vi "20191023_KEK_HEX5_events_new_config.vi"() -> ()   [LabVIEW 2017]
uses:
  <vilib>/DAQmx/create/channels.llb/DAQmx Create Channel (AI-Voltage-Basic).vi
  <vilib>/DAQmx/create/channels.llb/DAQmx Create Channel (AO-Voltage-Basic).vi
  <vilib>/DAQmx/miscellaneous.llb/DAQmx Fill In Error Info.vi
  Lake Shore Cryotronics 218.lvlib
panel:
  out "ref RAW":refnum<file>
  out "ref LSI-D":refnum<file>
  out "ref DAQ":refnum<file>
  in  "CSV filename suffix":string="Overnight_1030"
  in  "base path":path=path "C:/Users/TUCAN_rcnp/Desktop/Labview/KEK_20191023_HEX5/EXP"
  out "ref LSI-U":refnum<file>
  out "size(s)":i32[](array[numeric])=[11, 5]
  out "Cycle #":i32=311
  out "current time":timestamp=timestamp(3655268207.996145 s since 1904-01-01)
  in  "stop":bool
  in  "Tab Control":T1(tab)=enum." DAQ out"
  out "error out \n(LSIU)":errorcluster
  out "error out\n(file creation)":errorcluster
  out "error out\n(DAQ config)":errorcluster
  out "error out\n(DAQ OUT)":errorcluster
  out "error out \n(DAQ IN)":errorcluster
  out "error out \n(record LSIU)":errorcluster
  out "error out \n(record DAQ)":errorcluster
  out "error out DAQ close":errorcluster
  out "error out \n(LSID)":errorcluster
  out "error out \n(record LSID)":errorcluster
  out "errors plot cosmetic 1":errorcluster[](array[cluster])
  out "error plot content":errorcluster
  out "error plot cosmetic 2":errorcluster
  in  "comments DAQ (not recorded)":string[](array[string])=["", "", "", "", "", "", "The range of this is 0-10VDC", "", "", "", ""]
  in  "comments LSID (not recorded)":string[](array[string])=["", "", "", "", "Broken", "", "", ""]
  in  "comments LSIU (not recorded)":string[](array[string])=["", "", "", "", "", "", "", ""]
  in  "V_max(in)":dbl[](array[numeric])=[5.0, 0.15, 5.0, 5.0, 5.0, 5.0, 10.0, 5.0, 5.0, 5.0, 5.0]
  in  "NI DAQ AIN labels":string[](array[string])=["P_4KRES_COILIN", "LM_110", "DP_4He", "DP_3He", "FM_4He", "FM_3He", "LM_1700", "P_4He_IN", "Bar_anal", "bar_CDG1", "bar_CDG2"]
  in  "LSI-U CH labels":string[](array[string])=["4K_res", "HEX5_liq_IN", "HEX_liq_OUT", "1K_pot", "HEX5_gas_IN", "HEX5_gas_OUT", "JT_IN", "JT_OUT"]
  in  "LSI-D CH labels":string[](array[string])=["Hflex_low", "uper_duct", "Hflex_up", "DISABLED", "4K_res", "HEX5_liq_IN_PtCo", "HEX5_liq_OUT_PtCo", "1K_pot_PtCo"]
  in  "DAQ analog channels":tag[](array[tag])=["Dev1/ai1", "Dev1/ai2", "Dev1/ai3", "Dev1/ai4", "Dev1/ai5", "Dev1/ai6", "Dev1/ai7", "Dev1/ai16", "Dev1/ai18", "Dev1/ai19", "Dev1/ai20"]
  in  "V_min(in)":dbl[](array[numeric])=[0.0, 0.0, 0.0, 0.0, 0.0, 0.0, 0.0, 0.0, 0.0, 0.0, 0.0]
  out "DAQ CH OUT":string="O1"
  in  "DAQ  OUT":tag="Dev1/ao0"
  in  "DAQ OUT ON?":bool
  in  "V_min(out)":dbl
  in  "V_max(out)":dbl=5.0
  out "DAQ CH 2":string[](array[string])=["Q1", "Q2", "Q3", "Q4", "Q5", "Q6", "Q7", "Q8", "Q9", "Q10", "Q11"]
  out "LSI-D CH 2":string[](array[string])=["D1", "D2", "D3", "D4", "D5", "D6", "D7", "D8"]
  in  "DAQ sample #":i32=5
  out "LSI-U CH 2":string[](array[string])=["U1", "U2", "U3", "U4", "U5", "U6", "U7", "U8"]
  in  "VISA LSI218 UP":refnum<visa-resource-name>="GPIB0::3::INSTR"
  in  "VISA LSI218 DOWN":refnum<visa-resource-name>="GPIB0::11::INSTR"
  out "D idx":i32[](array[numeric])=[0, 1, 2, 3, 4, 5, 6, 7]
  out "LSI-U CH indic,":string[](array[string])=["4K_res", "HEX5_liq_IN", "HEX_liq_OUT", "1K_pot", "HEX5_gas_IN", "HEX5_gas_OUT", "JT_IN", "JT_OUT"]
  out "LSI-U out":dbl[](array[numeric])=[284.87, 0.0, 330.07, 0.718, 286.24, 89.901, 283.56, 272.5]
  in  "GraphU1 SEL":i32[](array[numeric])=[0, 1]
  out "LSI-D out":dbl[](array[numeric])=[296.51, 230.81, 237.57, 20.995, 4.242, 6.869, 297.3, 283.3]
  out "LSI-D CH indic.":string[](array[string])=["Hflex_low", "uper_duct", "Hflex_up", "DISABLED", "4K_res", "HEX5_liq_IN_PtCo", "HEX5_liq_OUT_PtCo", "1K_pot_PtCo"]
  in  "GraphU2 SEL":i32[](array[numeric])=[2, 3, 4]
  in  "GraphU3 SEL":i32[](array[numeric])=[5, 6, 6]
  in  "GraphD1 SEL":i32[](array[numeric])=[0, 1]
  in  "GraphD2 SEL":i32[](array[numeric])=[2, 3, 4]
  in  "GraphD3 SEL":i32[](array[numeric])=[5, 6, 6]
  out "LSI-D Grpah 1":cluster{dbl[], dbl[]}[](graph)=[{array[312 elements], [0.0, 296.61, 296.59, 296.63, 296.62, 296.61, 296.61, 296.61, 296.61, 296.61, 296.57, 296.65, 296.6, 296.66, 296.59, 296.6, 296.58, 296.64, 296.63, 296.66, 296.57, 296.61, 296.6, 296.6, 296.61, 296.61, 296.6, 296.6, 296.57, 296.62, 296.58, 296.59, 296.58, 296.61, 296.62, 296.57, 296.61, 296.63, 296.62, 296.64, 296.63, 296.6, 296.6, 296.57, 296.59, 296.59, 296.6, 296.59, 296.56, 296.6, 296.59, 296.61, 296.59, 296.58, 296.57, 296.59, 296.62, 296.59, 296.61, 296.6, 296.55, 296.6, 296.59, 296.59, 296.6, 296.61, 296.59, 296.57, 296.64, 296.67, 296.57, 296.62, 296.57, 296.58, 296.62, 296.61, 296.58, 296.55, 296.56, 296.59, 296.59, 296.6, 296.58, 296.57, 296.61, 296.58, 296.53, 296.54, 296.59, 296.55, 296.53, 296.59, 296.58, 296.58, 296.58, 296.55, 296.56, 296.56, 296.59, 296.53, 296.61, 296.62, 296.6, 296.58, 296.56, 296.53, 296.55, 296.59, 296.58, 296.6, 296.55, 296.59, 296.56, 296.56, 296.58, 296.57, 296.61, 296.55, 296.61, 296.57, 296.57, 296.58, 296.51, 296.55, 296.6, 296.6, 296.58, 296.56, 296.58, 296.57, 296.59, 296.55, 296.55, 296.56, 296.59, 296.52, 296.54, 296.58, 296.52, 296.54, 296.57, 296.54, 296.59, 296.52, 296.53, 296.55, 296.49, 296.54, 296.63, 296.56, 296.53, 296.54, 296.55, 296.58, 296.56, 296.51, 296.55, 296.57, 296.53, 296.52, 296.56, 296.58, 296.55, 296.61, 296.55, 296.58, 296.53, 296.58, 296.57, 296.52, 296.48, 296.53, 296.52, 296.54, 296.59, 296.53, 296.56, 296.55, 296.58, 296.56, 296.51, 296.52, 296.57, 296.54, 296.55, 296.55, 296.57, 296.59, 296.6, 296.55, 296.54, 296.51, 296.52, 296.55, 296.55, 296.54, 296.51, 296.49, 296.57, 296.55, 296.54, 296.56, 296.55, 296.53, 296.5, 296.55, 296.53, 296.54, 296.57, 296.52, 296.55, 296.55, 296.52, 296.5, 296.53, 296.53, 296.52, 296.54, 296.53, 296.52, 296.53, 296.51, 296.58, 296.49, 296.52, 296.55, 296.48, 296.51, 296.55, 296.48, 296.55, 296.5, 296.51, 296.55, 296.52, 296.54, 296.5, 296.54, 296.52, 296.53, 296.55, 296.53, 296.48, 296.58, 296.55, 296.52, 296.51, 296.49, 296.53, 296.5, 296.56, 296.53, 296.48, 296.54, 296.52, 296.56, 296.53, 296.5, 296.51, 296.5, 296.51, 296.47, 296.47, 296.57, 296.53, 296.49, 296.56, 296.55, 296.55, 296.51, 296.5, 296.52, 296.52, 296.48, 296.51, 296.54, 296.5, 296.49, 296.55, 296.5, 296.52, 296.54, 296.5, 296.51, 296.5, 296.53, 296.49, 296.51, 296.49, 296.54, 296.5, 296.51, 296.5, 296.54, 296.5, 296.48, 296.46, 296.5, 296.49, 296.49, 296.49, 296.51, 296.47, 296.49, 296.47, 296.49, 296.47, 296.49, 296.46, 296.49, 296.47, 296.51]}, {array[312 elements], [0.0, 246.36, 246.3, 246.25, 246.18, 246.13, 246.13, 246.1, 246.04, 246.01, 245.96, 245.88, 245.85, 245.76, 245.73, 245.71, 245.65, 245.59, 245.54, 245.5, 245.46, 245.41, 245.35, 245.32, 245.31, 245.24, 245.17, 245.15, 245.05, 245.05, 244.99, 244.94, 244.92, 244.85, 244.84, 244.72, 244.69, 244.62, 244.56, 244.56, 244.49, 244.46, 244.4, 244.4, 244.3, 244.3, 244.25, 244.17, 244.13, 244.08, 244.03, 243.99, 243.95, 243.89, 243.86, 243.79, 243.75, 243.69, 243.65, 243.6, 243.56, 243.49, 243.42, 243.43, 243.36, 243.34, 243.27, 243.21, 243.12, 243.17, 243.07, 243.05, 242.97, 242.87, 242.88, 242.8, 242.77, 242.72, 242.65, 242.64, 242.55, 242.51, 242.45, 242.46, 242.37, 242.29, 242.28, 242.21, 242.18, 242.14, 242.06, 242.07, 242.0, 241.92, 241.91, 241.84, 241.77, 241.71, 241.66, 241.64, 241.57, 241.52, 241.46, 241.4, 241.37, 241.32, 241.26, 241.23, 241.17, 241.15, 241.07, 241.0, 240.93, 240.92, 240.86, 240.78, 240.76, 240.7, 240.65, 240.57, 240.51, 240.46, 240.46, 240.37, 240.33, 240.29, 240.19, 240.16, 240.13, 240.09, 240.0, 239.96, 239.91, 239.87, 239.83, 239.75, 239.71, 239.63, 239.57, 239.52, 239.48, 239.39, 239.35, 239.35, 239.29, 239.2, 239.19, 239.07, 239.04, 239.02, 238.97, 238.87, 238.8, 238.79, 238.73, 238.67, 238.61, 238.57, 238.54, 238.45, 238.38, 238.36, 238.28, 238.24, 238.21, 238.17, 238.09, 238.05, 237.98, 237.95, 237.88, 237.82, 237.8, 237.73, 237.64, 237.6, 237.58, 237.52, 237.49, 237.43, 237.33, 237.29, 237.26, 237.22, 237.17, 237.11, 237.06, 237.01, 236.97, 236.91, 236.84, 236.8, 236.75, 236.69, 236.64, 236.56, 236.53, 236.45, 236.43, 236.38, 236.33, 236.28, 236.23, 236.16, 236.13, 236.07, 236.01, 235.93, 235.93, 235.88, 235.82, 235.78, 235.72, 235.63, 235.6, 235.57, 235.52, 235.47, 235.43, 235.34, 235.32, 235.25, 235.23, 235.16, 235.11, 235.07, 235.02, 234.92, 234.93, 234.85, 234.8, 234.75, 234.71, 234.65, 234.62, 234.52, 234.5, 234.47, 234.42, 234.38, 234.32, 234.23, 234.19, 234.14, 234.08, 234.06, 234.03, 233.95, 233.91, 233.85, 233.79, 233.74, 233.73, 233.68, 233.61, 233.58, 233.51, 233.46, 233.41, 233.36, 233.32, 233.27, 233.24, 233.16, 233.11, 233.11, 233.03, 232.95, 232.9, 232.89, 232.8, 232.8, 232.72, 232.69, 232.65, 232.58, 232.52, 232.5, 232.44, 232.38, 232.34, 232.26, 232.21, 232.17, 232.13, 232.11, 232.03, 231.97, 231.96, 231.91, 231.88, 231.82, 231.77, 231.7, 231.65, 231.59, 231.59, 231.49, 231.49, 231.38, 231.35, 231.31, 231.25, 231.21, 231.19, 231.16, 231.09, 230.99, 230.97, 230.95, 230.89, 230.81]}, {array[312 elements], [0.0, 251.98, 251.95, 251.89, 251.86, 251.82, 251.77, 251.73, 251.67, 251.64, 251.61, 251.56, 251.51, 251.45, 251.42, 251.36, 251.34, 251.3, 251.22, 251.19, 251.19, 251.14, 251.06, 251.04, 250.98, 250.95, 250.91, 250.87, 250.82, 250.77, 250.74, 250.67, 250.65, 250.6, 250.55, 250.52, 250.46, 250.41, 250.37, 250.34, 250.28, 250.24, 250.21, 250.15, 250.11, 250.08, 250.04, 249.99, 249.94, 249.87, 249.85, 249.81, 249.77, 249.73, 249.67, 249.63, 249.58, 249.55, 249.48, 249.47, 249.4, 249.35, 249.32, 249.28, 249.25, 249.19, 249.15, 249.1, 249.05, 249.01, 248.98, 248.92, 248.85, 248.82, 248.79, 248.76, 248.71, 248.65, 248.6, 248.55, 248.52, 248.47, 248.44, 248.38, 248.36, 248.3, 248.26, 248.19, 248.13, 248.12, 248.06, 248.03, 247.98, 247.93, 247.86, 247.85, 247.82, 247.74, 247.7, 247.66, 247.63, 247.58, 247.54, 247.48, 247.43, 247.4, 247.33, 247.3, 247.25, 247.2, 247.16, 247.1, 247.09, 247.02, 246.96, 246.93, 246.88, 246.85, 246.79, 246.76, 246.7, 246.66, 246.6, 246.58, 246.53, 246.47, 246.44, 246.4, 246.34, 246.28, 246.23, 246.18, 246.14, 246.1, 246.05, 246.01, 245.98, 245.94, 245.86, 245.85, 245.79, 245.72, 245.68, 245.65, 245.62, 245.54, 245.52, 245.46, 245.42, 245.37, 245.3, 245.28, 245.23, 245.15, 245.13, 245.08, 245.03, 244.97, 244.94, 244.89, 244.87, 244.8, 244.75, 244.71, 244.65, 244.62, 244.59, 244.53, 244.48, 244.4, 244.38, 244.32, 244.29, 244.25, 244.18, 244.15, 244.11, 244.06, 244.03, 243.93, 243.92, 243.85, 243.82, 243.75, 243.73, 243.67, 243.63, 243.57, 243.52, 243.49, 243.44, 243.38, 243.33, 243.29, 243.25, 243.21, 243.15, 243.11, 243.06, 243.0, 242.97, 242.92, 242.86, 242.83, 242.76, 242.74, 242.67, 242.61, 242.58, 242.55, 242.47, 242.45, 242.39, 242.34, 242.3, 242.25, 242.21, 242.16, 242.12, 242.06, 242.01, 241.94, 241.91, 241.86, 241.82, 241.76, 241.71, 241.67, 241.59, 241.56, 241.5, 241.48, 241.42, 241.38, 241.33, 241.29, 241.22, 241.18, 241.15, 241.09, 241.05, 241.0, 240.93, 240.9, 240.85, 240.8, 240.75, 240.71, 240.65, 240.62, 240.55, 240.52, 240.47, 240.41, 240.36, 240.3, 240.28, 240.21, 240.17, 240.11, 240.07, 240.03, 239.98, 239.93, 239.88, 239.83, 239.8, 239.73, 239.67, 239.63, 239.6, 239.54, 239.5, 239.42, 239.41, 239.36, 239.3, 239.24, 239.21, 239.16, 239.11, 239.04, 239.01, 238.94, 238.9, 238.85, 238.81, 238.76, 238.7, 238.67, 238.62, 238.56, 238.51, 238.48, 238.41, 238.38, 238.33, 238.28, 238.24, 238.17, 238.12, 238.07, 238.03, 237.95, 237.93, 237.88, 237.85, 237.78, 237.73, 237.68, 237.64, 237.57]}, {array[312 elements], [0.0, 22.529, 22.52, 22.516, 22.495, 22.486, 22.467, 22.467, 22.454, 22.443, 22.422, 22.419, 22.404, 22.383, 22.383, 22.362, 22.365, 22.347, 22.331, 22.329, 22.31, 22.305, 22.302, 22.294, 22.273, 22.277, 22.26, 22.241, 22.238, 22.231, 22.225, 22.194, 22.193, 22.182, 22.171, 22.163, 22.164, 22.165, 22.157, 22.138, 22.136, 22.124, 22.112, 22.109, 22.094, 22.078, 22.077, 22.076, 22.066, 22.067, 22.046, 22.048, 22.04, 22.032, 22.017, 22.004, 21.995, 21.997, 21.999, 21.975, 21.967, 21.961, 21.956, 21.949, 21.941, 21.93, 21.929, 21.91, 21.917, 21.916, 21.899, 21.888, 21.886, 21.878, 21.864, 21.846, 21.845, 21.839, 21.831, 21.821, 21.814, 21.797, 21.805, 21.796, 21.795, 21.776, 21.766, 21.78, 21.769, 21.767, 21.756, 21.738, 21.753, 21.729, 21.736, 21.73, 21.716, 21.707, 21.704, 21.702, 21.703, 21.689, 21.682, 21.682, 21.674, 21.661, 21.655, 21.66, 21.656, 21.646, 21.647, 21.634, 21.63, 21.626, 21.613, 21.616, 21.604, 21.603, 21.602, 21.592, 21.593, 21.589, 21.579, 21.575, 21.568, 21.561, 21.555, 21.557, 21.547, 21.541, 21.535, 21.531, 21.532, 21.53, 21.526, 21.523, 21.509, 21.503, 21.509, 21.501, 21.491, 21.505, 21.496, 21.496, 21.482, 21.483, 21.483, 21.473, 21.478, 21.485, 21.47, 21.473, 21.461, 21.459, 21.454, 21.442, 21.453, 21.462, 21.462, 21.456, 21.445, 21.445, 21.453, 21.457, 21.449, 21.449, 21.442, 21.447, 21.444, 21.446, 21.443, 21.446, 21.446, 21.449, 21.446, 21.449, 21.45, 21.455, 21.45, 21.446, 21.444, 21.442, 21.451, 21.44, 21.433, 21.45, 21.432, 21.441, 21.441, 21.44, 21.443, 21.43, 21.424, 21.421, 21.42, 21.43, 21.427, 21.416, 21.405, 21.406, 21.406, 21.414, 21.404, 21.417, 21.414, 21.406, 21.393, 21.401, 21.4, 21.393, 21.38, 21.369, 21.372, 21.379, 21.364, 21.376, 21.364, 21.347, 21.35, 21.365, 21.361, 21.346, 21.335, 21.349, 21.336, 21.321, 21.336, 21.331, 21.342, 21.335, 21.31, 21.331, 21.314, 21.324, 21.317, 21.292, 21.316, 21.282, 21.305, 21.298, 21.3, 21.286, 21.291, 21.278, 21.282, 21.28, 21.276, 21.255, 21.262, 21.269, 21.256, 21.241, 21.245, 21.239, 21.225, 21.233, 21.228, 21.23, 21.218, 21.218, 21.211, 21.215, 21.212, 21.213, 21.21, 21.2, 21.209, 21.204, 21.188, 21.2, 21.185, 21.18, 21.181, 21.166, 21.162, 21.166, 21.161, 21.139, 21.152, 21.143, 21.138, 21.131, 21.138, 21.133, 21.132, 21.123, 21.12, 21.119, 21.114, 21.107, 21.108, 21.1, 21.089, 21.091, 21.082, 21.083, 21.083, 21.073, 21.072, 21.059, 21.055, 21.048, 21.04, 21.044, 21.035, 21.02, 21.025, 21.009, 21.019, 21.009, 21.001, 20.995]}, {array[312 elements], [0.0, 4.244, 4.243, 4.243, 4.243, 4.243, 4.243, 4.243, 4.243, 4.243, 4.243, 4.243, 4.243, 4.243, 4.242, 4.243, 4.243, 4.243, 4.243, 4.242, 4.244, 4.243, 4.244, 4.243, 4.242, 4.243, 4.243, 4.243, 4.243, 4.243, 4.243, 4.243, 4.243, 4.243, 4.243, 4.243, 4.243, 4.243, 4.243, 4.243, 4.244, 4.244, 4.243, 4.243, 4.243, 4.244, 4.243, 4.243, 4.243, 4.243, 4.243, 4.243, 4.242, 4.243, 4.243, 4.243, 4.243, 4.243, 4.243, 4.243, 4.243, 4.243, 4.243, 4.243, 4.243, 4.243, 4.242, 4.243, 4.243, 4.242, 4.242, 4.242, 4.243, 4.243, 4.242, 4.243, 4.243, 4.242, 4.243, 4.243, 4.242, 4.243, 4.243, 4.243, 4.243, 4.243, 4.242, 4.243, 4.242, 4.242, 4.243, 4.243, 4.243, 4.242, 4.242, 4.243, 4.243, 4.242, 4.242, 4.242, 4.242, 4.242, 4.243, 4.243, 4.243, 4.243, 4.243, 4.243, 4.243, 4.243, 4.243, 4.242, 4.243, 4.243, 4.243, 4.242, 4.243, 4.242, 4.243, 4.243, 4.243, 4.243, 4.242, 4.242, 4.242, 4.243, 4.242, 4.243, 4.243, 4.242, 4.242, 4.242, 4.242, 4.242, 4.243, 4.243, 4.243, 4.242, 4.242, 4.242, 4.242, 4.243, 4.242, 4.242, 4.242, 4.242, 4.242, 4.242, 4.242, 4.243, 4.243, 4.242, 4.242, 4.242, 4.242, 4.242, 4.243, 4.242, 4.243, 4.243, 4.242, 4.242, 4.242, 4.242, 4.242, 4.243, 4.242, 4.243, 4.243, 4.243, 4.242, 4.243, 4.242, 4.243, 4.243, 4.242, 4.242, 4.242, 4.242, 4.242, 4.242, 4.242, 4.242, 4.242, 4.242, 4.242, 4.242, 4.242, 4.242, 4.242, 4.242, 4.242, 4.243, 4.242, 4.242, 4.242, 4.243, 4.242, 4.242, 4.242, 4.242, 4.242, 4.243, 4.242, 4.242, 4.242, 4.242, 4.242, 4.242, 4.242, 4.242, 4.242, 4.242, 4.242, 4.243, 4.242, 4.242, 4.242, 4.242, 4.241, 4.242, 4.242, 4.242, 4.242, 4.242, 4.242, 4.242, 4.242, 4.243, 4.242, 4.242, 4.242, 4.242, 4.242, 4.242, 4.242, 4.243, 4.242, 4.242, 4.242, 4.242, 4.241, 4.242, 4.242, 4.242, 4.242, 4.242, 4.242, 4.242, 4.242, 4.242, 4.243, 4.242, 4.242, 4.242, 4.242, 4.242, 4.242, 4.242, 4.242, 4.242, 4.242, 4.242, 4.241, 4.242, 4.241, 4.242, 4.242, 4.242, 4.242, 4.242, 4.242, 4.241, 4.241, 4.242, 4.242, 4.241, 4.241, 4.241, 4.242, 4.241, 4.242, 4.242, 4.242, 4.242, 4.242, 4.242, 4.242, 4.242, 4.242, 4.242, 4.242, 4.242, 4.241, 4.242, 4.242, 4.241, 4.242, 4.242, 4.242, 4.242, 4.241, 4.242, 4.241, 4.242, 4.242, 4.241, 4.242, 4.242, 4.241, 4.242, 4.242]}, {array[312 elements], [0.0, 6.751, 6.741, 6.737, 6.736, 6.748, 6.752, 6.743, 6.739, 6.737, 6.744, 6.752, 6.753, 6.747, 6.741, 6.737, 6.737, 6.741, 6.748, 6.755, 6.756, 6.755, 6.75, 6.748, 6.745, 6.744, 6.743, 6.746, 6.75, 6.755, 6.761, 6.761, 6.758, 6.752, 6.75, 6.747, 6.747, 6.745, 6.745, 6.747, 6.753, 6.756, 6.764, 6.764, 6.763, 6.76, 6.755, 6.754, 6.752, 6.752, 6.752, 6.752, 6.751, 6.751, 6.751, 6.751, 6.753, 6.757, 6.759, 6.76, 6.764, 6.766, 6.766, 6.77, 6.771, 6.769, 6.77, 6.769, 6.769, 6.769, 6.767, 6.768, 6.764, 6.764, 6.763, 6.759, 6.76, 6.759, 6.758, 6.759, 6.76, 6.762, 6.762, 6.763, 6.765, 6.767, 6.769, 6.771, 6.774, 6.779, 6.78, 6.78, 6.782, 6.782, 6.781, 6.777, 6.775, 6.772, 6.77, 6.768, 6.768, 6.771, 6.773, 6.773, 6.777, 6.78, 6.786, 6.788, 6.787, 6.78, 6.776, 6.773, 6.774, 6.776, 6.78, 6.786, 6.789, 6.79, 6.785, 6.776, 6.775, 6.778, 6.781, 6.788, 6.793, 6.79, 6.78, 6.775, 6.778, 6.782, 6.79, 6.794, 6.789, 6.78, 6.78, 6.782, 6.786, 6.795, 6.796, 6.788, 6.782, 6.784, 6.787, 6.794, 6.8, 6.792, 6.785, 6.788, 6.797, 6.802, 6.796, 6.785, 6.786, 6.79, 6.802, 6.8, 6.788, 6.789, 6.794, 6.804, 6.804, 6.792, 6.791, 6.795, 6.804, 6.804, 6.793, 6.792, 6.795, 6.803, 6.807, 6.796, 6.792, 6.797, 6.807, 6.8, 6.792, 6.799, 6.808, 6.797, 6.793, 6.803, 6.81, 6.794, 6.798, 6.809, 6.807, 6.797, 6.802, 6.812, 6.807, 6.816, 6.829, 6.84, 6.828, 6.828, 6.838, 6.838, 6.826, 6.831, 6.843, 6.831, 6.83, 6.84, 6.841, 6.828, 6.835, 6.846, 6.831, 6.833, 6.846, 6.839, 6.834, 6.842, 6.843, 6.833, 6.842, 6.849, 6.833, 6.843, 6.849, 6.834, 6.842, 6.85, 6.835, 6.843, 6.848, 6.836, 6.842, 6.849, 6.837, 6.848, 6.848, 6.839, 6.851, 6.846, 6.84, 6.85, 6.844, 6.841, 6.853, 6.84, 6.844, 6.856, 6.841, 6.845, 6.857, 6.84, 6.85, 6.85, 6.843, 6.856, 6.847, 6.845, 6.858, 6.844, 6.848, 6.858, 6.846, 6.858, 6.843, 6.852, 6.852, 6.846, 6.859, 6.845, 6.853, 6.853, 6.848, 6.86, 6.846, 6.858, 6.847, 6.852, 6.854, 6.849, 6.863, 6.848, 6.861, 6.847, 6.856, 6.855, 6.852, 6.861, 6.85, 6.864, 6.848, 6.863, 6.85, 6.854, 6.859, 6.851, 6.865, 6.851, 6.865, 6.851, 6.864, 6.853, 6.859, 6.855, 6.859, 6.862, 6.857, 6.867, 6.856, 6.869, 6.856, 6.87, 6.855, 6.871, 6.855, 6.869]}, {array[312 elements], [0.0, 295.97, 296.04, 295.97, 296.06, 295.86, 295.93, 296.04, 295.99, 296.15, 295.97, 296.14, 296.11, 296.03, 296.06, 296.03, 296.11, 296.2, 295.93, 296.04, 295.99, 296.02, 295.99, 296.1, 296.14, 295.73, 296.02, 296.15, 296.14, 295.92, 296.02, 296.15, 296.0, 296.04, 296.15, 296.25, 296.31, 296.02, 296.13, 296.22, 296.37, 296.22, 296.27, 296.35, 296.13, 296.22, 295.7, 296.18, 295.95, 296.22, 296.39, 296.14, 296.25, 296.1, 296.15, 296.13, 296.2, 296.14, 296.23, 296.2, 296.2, 296.06, 296.18, 296.27, 296.42, 296.31, 296.31, 296.31, 296.11, 296.22, 296.16, 296.23, 296.33, 296.14, 296.06, 296.43, 296.31, 296.2, 296.16, 296.13, 296.4, 296.23, 296.5, 296.4, 296.31, 296.1, 296.51, 296.42, 296.37, 296.43, 296.4, 296.31, 296.27, 296.54, 296.36, 296.27, 296.44, 296.35, 296.27, 296.42, 296.22, 296.43, 296.31, 296.54, 296.55, 296.4, 296.39, 296.31, 296.33, 296.5, 296.5, 296.44, 296.53, 296.47, 296.36, 296.49, 296.44, 296.58, 296.36, 296.31, 296.47, 296.49, 296.25, 296.47, 296.66, 296.51, 296.4, 296.49, 296.49, 296.18, 296.47, 296.56, 296.51, 296.55, 296.62, 296.6, 296.6, 296.47, 296.47, 296.58, 296.63, 296.58, 296.58, 296.56, 296.6, 296.47, 296.42, 296.37, 296.42, 296.49, 296.37, 296.53, 296.5, 296.6, 296.56, 296.63, 296.71, 296.58, 296.51, 296.43, 296.77, 296.36, 296.63, 296.44, 296.73, 296.73, 296.6, 296.74, 296.5, 296.51, 296.5, 296.42, 296.65, 296.58, 296.4, 296.31, 296.53, 296.43, 296.69, 296.66, 296.65, 296.62, 296.71, 296.6, 296.35, 296.7, 296.65, 296.6, 296.67, 296.63, 296.78, 296.91, 296.86, 296.69, 296.74, 296.55, 296.6, 296.91, 296.76, 296.67, 296.76, 296.71, 296.94, 296.63, 296.86, 296.63, 296.7, 296.82, 296.8, 296.74, 296.74, 296.73, 296.96, 296.76, 296.74, 296.8, 296.84, 296.86, 296.83, 296.77, 296.89, 296.65, 296.77, 296.84, 296.71, 296.76, 296.74, 296.89, 296.8, 296.74, 296.82, 296.87, 296.8, 297.0, 297.16, 297.09, 296.98, 296.83, 296.89, 296.89, 296.54, 296.89, 296.78, 296.87, 297.21, 297.14, 296.78, 296.73, 296.87, 297.14, 297.03, 297.14, 297.1, 297.09, 297.02, 296.78, 297.25, 297.21, 297.0, 297.03, 296.98, 296.94, 296.93, 296.93, 297.03, 297.07, 296.89, 297.05, 297.02, 296.98, 296.95, 296.96, 296.87, 296.95, 297.07, 297.13, 296.96, 297.07, 297.0, 297.16, 297.17, 297.05, 296.93, 296.91, 297.07, 296.98, 297.1, 297.03, 297.19, 297.05, 297.0, 297.07, 297.16, 297.13, 297.0, 297.21, 296.94, 297.3, 297.05, 297.12, 297.28, 297.21, 297.17, 297.23, 297.25, 297.25, 297.21, 297.21, 297.13, 297.17, 297.29, 297.3]}, {array[312 elements], [0.0, 281.87, 284.61, 281.99, 283.5, 282.29, 284.54, 281.98, 283.46, 284.72, 281.54, 282.9, 285.03, 283.14, 281.87, 281.54, 283.76, 284.61, 283.77, 283.35, 282.81, 281.49, 282.64, 284.24, 282.04, 283.31, 281.38, 284.43, 281.46, 284.59, 281.26, 283.93, 282.21, 282.76, 283.46, 282.65, 284.47, 281.69, 284.72, 282.51, 283.24, 282.89, 283.52, 281.43, 284.24, 281.77, 282.2, 284.47, 282.72, 282.56, 284.67, 281.3, 283.69, 282.76, 281.24, 284.17, 281.24, 283.14, 282.61, 281.26, 283.55, 282.98, 281.62, 283.87, 282.12, 282.56, 284.26, 281.95, 284.13, 281.11, 283.82, 280.96, 283.39, 282.37, 281.73, 283.39, 282.29, 283.76, 282.07, 283.87, 282.21, 282.35, 283.01, 281.11, 284.39, 281.29, 283.77, 281.26, 283.8, 280.91, 284.29, 281.18, 283.31, 281.79, 284.37, 282.32, 283.14, 282.61, 282.51, 283.77, 281.74, 283.06, 281.43, 284.09, 282.35, 281.98, 284.26, 282.65, 281.95, 284.88, 283.01, 281.07, 284.18, 283.55, 281.3, 282.68, 283.9, 283.11, 281.65, 282.59, 283.47, 283.01, 282.43, 281.41, 282.95, 284.1, 282.89, 281.13, 284.54, 282.24, 282.72, 282.68, 283.46, 281.74, 283.85, 283.03, 282.64, 283.01, 283.11, 282.17, 283.87, 281.82, 284.02, 282.12, 283.16, 284.39, 281.65, 284.13, 281.21, 283.47, 283.72, 281.49, 282.76, 284.77, 282.15, 282.4, 283.52, 284.13, 283.31, 282.28, 281.85, 282.9, 283.9, 284.29, 284.54, 284.51, 283.85, 283.03, 283.11, 283.9, 284.51, 282.98, 283.47, 284.67, 281.99, 282.53, 284.42, 283.31, 282.15, 284.8, 283.93, 281.66, 283.11, 284.8, 282.9, 283.35, 283.39, 282.61, 283.16, 281.73, 281.38, 283.76, 284.81, 284.81, 283.5, 283.01, 284.72, 282.53, 284.64, 282.83, 284.24, 282.83, 283.8, 283.82, 282.04, 284.13, 284.13, 282.59, 283.42, 285.13, 282.59, 281.99, 283.31, 282.32, 282.95, 283.16, 283.39, 284.54, 284.42, 281.66, 282.61, 284.39, 282.98, 281.54, 285.03, 283.38, 282.56, 284.72, 283.08, 282.76, 284.47, 283.08, 282.64, 283.8, 284.88, 284.61, 284.73, 283.63, 281.79, 281.54, 283.24, 283.27, 281.66, 282.61, 283.93, 284.39, 282.37, 283.39, 284.67, 281.91, 284.59, 283.38, 281.82, 284.96, 282.2, 284.88, 281.73, 284.09, 281.74, 285.05, 282.2, 282.45, 284.01, 281.18, 282.9, 282.48, 283.52, 282.98, 283.22, 282.32, 284.13, 283.85, 281.11, 282.37, 284.59, 284.8, 284.59, 282.98, 282.07, 282.28, 282.83, 283.72, 283.38, 282.83, 282.07, 283.01, 282.78, 283.3, 281.49, 283.06, 282.21, 283.39, 281.85, 283.22, 282.28, 283.42, 282.95, 283.64, 281.33, 284.77, 282.29, 282.12, 283.69, 284.05, 281.74, 283.08, 283.72, 282.59, 281.43, 282.59, 282.81, 283.3]}, {array[312 elements], []}]
  out "LSI-U Grpah 1":cluster{dbl[], dbl[]}[](graph)=[{array[312 elements], [286.85, 286.84, 286.82, 286.84, 286.77, 286.76, 286.74, 286.79, 286.78, 286.78, 286.83, 286.73, 286.76, 286.74, 286.76, 286.75, 286.72, 286.77, 286.72, 286.69, 286.75, 286.7, 286.68, 286.7, 286.64, 286.69, 286.65, 286.68, 286.7, 286.67, 286.64, 286.62, 286.64, 286.63, 286.64, 286.62, 286.6, 286.61, 286.63, 286.61, 286.59, 286.61, 286.59, 286.59, 286.59, 286.59, 286.54, 286.56, 286.54, 286.52, 286.56, 286.54, 286.54, 286.51, 286.51, 286.49, 286.53, 286.47, 286.51, 286.51, 286.5, 286.48, 286.47, 286.44, 286.47, 286.46, 286.46, 286.43, 286.41, 286.39, 286.43, 286.41, 286.4, 286.38, 286.4, 286.39, 286.36, 286.42, 286.38, 286.32, 286.36, 286.32, 286.37, 286.36, 286.3, 286.34, 286.33, 286.33, 286.31, 286.25, 286.27, 286.24, 286.28, 286.3, 286.31, 286.26, 286.26, 286.22, 286.23, 286.25, 286.23, 286.26, 286.2, 286.21, 286.22, 286.22, 286.2, 286.19, 286.19, 286.15, 286.18, 286.19, 286.17, 286.16, 286.17, 286.18, 286.15, 286.13, 286.17, 286.1, 286.08, 286.1, 286.14, 286.08, 286.11, 286.07, 286.08, 286.06, 286.08, 286.09, 286.04, 286.02, 286.03, 286.05, 286.01, 286.04, 286.04, 286.01, 286.01, 286.0, 285.98, 286.03, 286.0, 285.97, 285.98, 285.97, 286.0, 285.99, 285.91, 285.91, 285.89, 285.96, 285.95, 285.94, 285.93, 285.9, 285.89, 285.88, 285.89, 285.91, 285.88, 285.87, 285.85, 285.84, 285.84, 285.86, 285.84, 285.82, 285.81, 285.81, 285.79, 285.81, 285.81, 285.8, 285.77, 285.76, 285.81, 285.77, 285.79, 285.73, 285.76, 285.72, 285.71, 285.75, 285.71, 285.71, 285.73, 285.69, 285.74, 285.71, 285.7, 285.7, 285.64, 285.66, 285.63, 285.67, 285.69, 285.64, 285.63, 285.62, 285.63, 285.63, 285.61, 285.56, 285.55, 285.57, 285.57, 285.56, 285.55, 285.58, 285.54, 285.56, 285.52, 285.54, 285.55, 285.5, 285.54, 285.49, 285.51, 285.46, 285.45, 285.5, 285.52, 285.46, 285.47, 285.49, 285.47, 285.47, 285.42, 285.44, 285.42, 285.4, 285.41, 285.46, 285.4, 285.37, 285.39, 285.36, 285.37, 285.37, 285.37, 285.36, 285.39, 285.31, 285.32, 285.35, 285.29, 285.3, 285.29, 285.33, 285.3, 285.31, 285.28, 285.26, 285.29, 285.26, 285.22, 285.23, 285.23, 285.22, 285.28, 285.23, 285.2, 285.19, 285.2, 285.2, 285.16, 285.22, 285.18, 285.18, 285.17, 285.14, 285.13, 285.12, 285.13, 285.11, 285.16, 285.16, 285.1, 285.11, 285.09, 285.08, 285.09, 285.07, 285.08, 285.08, 285.05, 285.05, 285.02, 285.05, 285.05, 284.99, 285.04, 285.01, 285.01, 284.97, 284.99, 285.0, 284.95, 284.98, 284.95, 284.99, 284.94, 284.93, 284.92, 284.92, 284.91, 284.93, 284.88, 284.91, 284.9, 284.87]}, {array[312 elements], [0.0, 0.0, 0.0, 0.0, 0.0, 0.0, 0.0, 0.0, 0.0, 0.0, 0.0, 0.0, 0.0, 0.0, 0.0, 0.0, 0.0, 0.0, 0.0, 0.0, 0.0, 0.0, 0.0, 0.0, 0.0, 0.0, 0.0, 0.0, 0.0, 0.0, 0.0, 0.0, 0.0, 0.0, 0.0, 0.0, 0.0, 0.0, 0.0, 0.0, 0.0, 0.0, 0.0, 0.0, 0.0, 0.0, 0.0, 0.0, 0.0, 0.0, 0.0, 0.0, 0.0, 0.0, 0.0, 0.0, 0.0, 0.0, 0.0, 0.0, 0.0, 0.0, 0.0, 0.0, 0.0, 0.0, 0.0, 0.0, 0.0, 0.0, 0.0, 0.0, 0.0, 0.0, 0.0, 0.0, 0.0, 0.0, 0.0, 0.0, 0.0, 0.0, 0.0, 0.0, 0.0, 0.0, 0.0, 0.0, 0.0, 0.0, 0.0, 0.0, 0.0, 0.0, 0.0, 0.0, 0.0, 0.0, 0.0, 0.0, 0.0, 0.0, 0.0, 0.0, 0.0, 0.0, 0.0, 0.0, 0.0, 0.0, 0.0, 0.0, 0.0, 0.0, 0.0, 0.0, 0.0, 0.0, 0.0, 0.0, 0.0, 0.0, 0.0, 0.0, 0.0, 0.0, 0.0, 0.0, 0.0, 0.0, 0.0, 0.0, 0.0, 0.0, 0.0, 0.0, 0.0, 0.0, 0.0, 0.0, 0.0, 0.0, 0.0, 0.0, 0.0, 0.0, 0.0, 0.0, 0.0, 0.0, 0.0, 0.0, 0.0, 0.0, 0.0, 0.0, 0.0, 0.0, 0.0, 0.0, 0.0, 0.0, 0.0, 0.0, 0.0, 0.0, 0.0, 0.0, 0.0, 0.0, 0.0, 0.0, 0.0, 0.0, 0.0, 0.0, 0.0, 0.0, 0.0, 0.0, 0.0, 0.0, 0.0, 0.0, 0.0, 0.0, 0.0, 0.0, 0.0, 0.0, 0.0, 0.0, 0.0, 0.0, 0.0, 0.0, 0.0, 0.0, 0.0, 0.0, 0.0, 0.0, 0.0, 0.0, 0.0, 0.0, 0.0, 0.0, 0.0, 0.0, 0.0, 0.0, 0.0, 0.0, 0.0, 0.0, 0.0, 0.0, 0.0, 0.0, 0.0, 0.0, 0.0, 0.0, 0.0, 0.0, 0.0, 0.0, 0.0, 0.0, 0.0, 0.0, 0.0, 0.0, 0.0, 0.0, 0.0, 0.0, 0.0, 0.0, 0.0, 0.0, 0.0, 0.0, 0.0, 0.0, 0.0, 0.0, 0.0, 0.0, 0.0, 0.0, 0.0, 0.0, 0.0, 0.0, 0.0, 0.0, 0.0, 0.0, 0.0, 0.0, 0.0, 0.0, 0.0, 0.0, 0.0, 0.0, 0.0, 0.0, 0.0, 0.0, 0.0, 0.0, 0.0, 0.0, 0.0, 0.0, 0.0, 0.0, 0.0, 0.0, 0.0, 0.0, 0.0, 0.0, 0.0, 0.0, 0.0, 0.0, 0.0, 0.0, 0.0, 0.0, 0.0, 0.0, 0.0, 0.0, 0.0, 0.0, 0.0, 0.0, 0.0, 0.0, 0.0, 0.0, 0.0, 0.0, 0.0, 0.0, 0.0, 0.0]}, {array[312 elements], [330.07, 330.07, 330.07, 330.07, 330.07, 330.07, 330.07, 330.07, 330.07, 330.07, 330.07, 330.07, 330.07, 330.07, 330.07, 330.07, 330.07, 330.07, 330.07, 330.07, 330.07, 330.07, 330.07, 330.07, 330.07, 330.07, 330.07, 330.07, 330.07, 330.07, 330.07, 330.07, 330.07, 330.07, 330.07, 330.07, 330.07, 330.07, 330.07, 330.07, 330.07, 330.07, 330.07, 330.07, 330.07, 330.07, 330.07, 330.07, 330.07, 330.07, 330.07, 330.07, 330.07, 330.07, 330.07, 330.07, 330.07, 330.07, 330.07, 330.07, 330.07, 330.07, 330.07, 330.07, 330.07, 330.07, 330.07, 330.07, 330.07, 330.07, 330.07, 330.07, 330.07, 330.07, 330.07, 330.07, 330.07, 330.07, 330.07, 330.07, 330.07, 330.07, 330.07, 330.07, 330.07, 330.07, 330.07, 330.07, 330.07, 330.07, 330.07, 330.07, 330.07, 330.07, 330.07, 330.07, 330.07, 330.07, 330.07, 330.07, 330.07, 330.07, 330.07, 330.07, 330.07, 330.07, 330.07, 330.07, 330.07, 330.07, 330.07, 330.07, 330.07, 330.07, 330.07, 330.07, 330.07, 330.07, 330.07, 330.07, 330.07, 330.07, 330.07, 330.07, 330.07, 330.07, 330.07, 330.07, 330.07, 330.07, 330.07, 330.07, 330.07, 330.07, 330.07, 330.07, 330.07, 330.07, 330.07, 330.07, 330.07, 330.07, 330.07, 330.07, 330.07, 330.07, 330.07, 330.07, 330.07, 330.07, 330.07, 330.07, 330.07, 330.07, 330.07, 330.07, 330.07, 330.07, 330.07, 330.07, 330.07, 330.07, 330.07, 330.07, 330.07, 330.07, 330.07, 330.07, 330.07, 330.07, 330.07, 330.07, 330.07, 330.07, 330.07, 330.07, 330.07, 330.07, 330.07, 330.07, 330.07, 330.07, 330.07, 330.07, 330.07, 330.07, 330.07, 330.07, 330.07, 330.07, 330.07, 330.07, 330.07, 330.07, 330.07, 330.07, 330.07, 330.07, 330.07, 330.07, 330.07, 330.07, 330.07, 330.07, 330.07, 330.07, 330.07, 330.07, 330.07, 330.07, 330.07, 330.07, 330.07, 330.07, 330.07, 330.07, 330.07, 330.07, 330.07, 330.07, 330.07, 330.07, 330.07, 330.07, 330.07, 330.07, 330.07, 330.07, 330.07, 330.07, 330.07, 330.07, 330.07, 330.07, 330.07, 330.07, 330.07, 330.07, 330.07, 330.07, 330.07, 330.07, 330.07, 330.07, 330.07, 330.07, 330.07, 330.07, 330.07, 330.07, 330.07, 330.07, 330.07, 330.07, 330.07, 330.07, 330.07, 330.07, 330.07, 330.07, 330.07, 330.07, 330.07, 330.07, 330.07, 330.07, 330.07, 330.07, 330.07, 330.07, 330.07, 330.07, 330.07, 330.07, 330.07, 330.07, 330.07, 330.07, 330.07, 330.07, 330.07, 330.07, 330.07, 330.07, 330.07, 330.07, 330.07, 330.07, 330.07, 330.07, 330.07, 330.07, 330.07, 330.07, 330.07, 330.07, 330.07, 330.07, 330.07, 330.07, 330.07, 330.07, 330.07, 330.07, 330.07, 330.07, 330.07, 330.07, 330.07, 330.07, 330.07, 330.07]}, {array[312 elements], [0.718, 0.718, 0.718, 0.718, 0.718, 0.718, 0.718, 0.718, 0.718, 0.718, 0.718, 0.718, 0.718, 0.718, 0.718, 0.718, 0.718, 0.718, 0.718, 0.718, 0.718, 0.718, 0.718, 0.718, 0.718, 0.718, 0.718, 0.718, 0.718, 0.718, 0.718, 0.718, 0.718, 0.718, 0.718, 0.718, 0.718, 0.718, 0.718, 0.718, 0.718, 0.718, 0.718, 0.718, 0.718, 0.718, 0.718, 0.718, 0.718, 0.718, 0.718, 0.718, 0.718, 0.718, 0.718, 0.718, 0.718, 0.718, 0.718, 0.718, 0.718, 0.718, 0.718, 0.718, 0.718, 0.718, 0.718, 0.718, 0.718, 0.718, 0.718, 0.718, 0.718, 0.718, 0.718, 0.718, 0.718, 0.718, 0.718, 0.718, 0.718, 0.718, 0.718, 0.718, 0.718, 0.718, 0.718, 0.718, 0.718, 0.718, 0.718, 0.718, 0.718, 0.718, 0.718, 0.718, 0.718, 0.718, 0.718, 0.718, 0.718, 0.718, 0.718, 0.718, 0.718, 0.718, 0.718, 0.718, 0.718, 0.718, 0.718, 0.718, 0.718, 0.718, 0.718, 0.718, 0.718, 0.718, 0.718, 0.718, 0.718, 0.718, 0.718, 0.718, 0.718, 0.718, 0.718, 0.718, 0.718, 0.718, 0.718, 0.718, 0.718, 0.718, 0.718, 0.718, 0.718, 0.718, 0.718, 0.718, 0.718, 0.718, 0.718, 0.718, 0.718, 0.718, 0.718, 0.718, 0.718, 0.718, 0.718, 0.718, 0.718, 0.718, 0.718, 0.718, 0.718, 0.718, 0.718, 0.718, 0.718, 0.718, 0.718, 0.718, 0.718, 0.718, 0.718, 0.718, 0.718, 0.718, 0.718, 0.718, 0.718, 0.718, 0.718, 0.718, 0.718, 0.718, 0.718, 0.718, 0.718, 0.718, 0.718, 0.718, 0.718, 0.718, 0.718, 0.718, 0.718, 0.718, 0.718, 0.718, 0.718, 0.718, 0.718, 0.718, 0.718, 0.718, 0.718, 0.718, 0.718, 0.718, 0.718, 0.718, 0.718, 0.718, 0.718, 0.718, 0.718, 0.718, 0.718, 0.718, 0.718, 0.718, 0.718, 0.718, 0.718, 0.718, 0.718, 0.718, 0.718, 0.718, 0.718, 0.718, 0.718, 0.718, 0.718, 0.718, 0.718, 0.718, 0.718, 0.718, 0.718, 0.718, 0.718, 0.718, 0.718, 0.718, 0.718, 0.718, 0.718, 0.718, 0.718, 0.718, 0.718, 0.718, 0.718, 0.718, 0.718, 0.718, 0.718, 0.718, 0.718, 0.718, 0.718, 0.718, 0.718, 0.718, 0.718, 0.718, 0.718, 0.718, 0.718, 0.718, 0.718, 0.718, 0.718, 0.718, 0.718, 0.718, 0.718, 0.718, 0.718, 0.718, 0.718, 0.718, 0.718, 0.718, 0.718, 0.718, 0.718, 0.718, 0.718, 0.718, 0.718, 0.718, 0.718, 0.718, 0.718, 0.718, 0.718, 0.718, 0.718, 0.718, 0.718, 0.718, 0.718, 0.718, 0.718, 0.718, 0.718, 0.718, 0.718, 0.718, 0.718, 0.718, 0.718, 0.718, 0.718, 0.718, 0.718, 0.718]}, {array[312 elements], [288.19, 288.31, 287.72, 287.34, 288.17, 287.14, 288.1, 287.28, 287.57, 288.17, 286.38, 287.7, 287.69, 286.99, 287.06, 288.23, 288.52, 287.14, 286.56, 287.02, 287.27, 287.72, 288.17, 287.23, 287.53, 287.43, 287.99, 286.91, 287.47, 286.58, 288.29, 286.41, 288.36, 287.14, 287.67, 287.94, 286.58, 288.14, 286.59, 287.47, 288.1, 286.88, 288.27, 287.3, 287.23, 287.85, 286.61, 288.17, 286.96, 286.76, 288.14, 286.44, 288.44, 286.93, 287.73, 287.82, 286.29, 288.02, 286.56, 287.76, 287.55, 286.68, 288.19, 286.58, 287.78, 287.64, 287.05, 288.14, 286.98, 288.06, 287.27, 287.57, 287.72, 286.84, 288.26, 286.22, 287.68, 286.48, 287.69, 286.31, 287.77, 286.16, 288.19, 286.91, 287.11, 287.16, 287.08, 287.06, 287.21, 286.93, 288.12, 286.26, 287.91, 286.36, 287.64, 286.9, 286.83, 288.02, 287.08, 287.25, 288.07, 286.81, 288.07, 287.3, 287.08, 288.19, 286.76, 286.88, 287.91, 286.8, 286.34, 288.38, 287.13, 286.99, 287.83, 287.28, 286.37, 287.23, 288.07, 287.15, 286.41, 287.15, 287.74, 287.47, 287.04, 286.66, 287.33, 287.44, 286.16, 288.23, 286.26, 288.27, 287.07, 287.12, 287.66, 286.19, 288.26, 286.72, 288.23, 286.1, 287.47, 286.53, 287.13, 287.23, 286.51, 287.62, 286.31, 288.08, 286.83, 287.59, 287.36, 286.91, 288.16, 286.41, 286.84, 288.07, 287.29, 286.27, 287.05, 288.22, 287.44, 286.19, 286.25, 286.09, 286.78, 286.99, 288.29, 287.73, 286.07, 286.77, 287.98, 286.86, 286.51, 288.03, 286.48, 287.39, 288.04, 286.01, 286.91, 287.82, 286.93, 285.98, 287.68, 287.95, 286.56, 286.61, 286.03, 286.19, 286.36, 286.35, 287.45, 288.01, 287.25, 286.55, 287.13, 288.08, 286.08, 288.01, 286.19, 288.23, 286.4, 288.3, 286.19, 287.46, 286.9, 286.31, 288.07, 287.28, 286.25, 287.33, 287.23, 286.77, 286.16, 286.23, 286.86, 286.91, 288.11, 287.87, 286.26, 286.48, 288.21, 287.07, 286.68, 287.65, 287.0, 286.31, 287.68, 286.73, 286.51, 287.98, 286.63, 287.21, 288.09, 287.65, 286.93, 286.78, 286.06, 286.71, 287.32, 287.91, 286.8, 287.05, 288.08, 286.7, 286.16, 288.19, 287.03, 286.96, 288.14, 286.07, 287.34, 287.55, 286.81, 287.21, 286.76, 287.0, 286.98, 286.95, 286.98, 286.29, 288.06, 287.12, 286.74, 287.92, 286.73, 286.38, 287.85, 286.03, 287.92, 287.06, 286.75, 287.53, 287.13, 286.23, 285.9, 286.93, 287.02, 288.08, 287.87, 286.38, 286.03, 287.05, 287.73, 288.12, 286.83, 285.98, 287.64, 287.74, 286.34, 287.91, 286.63, 287.37, 286.26, 287.76, 286.93, 287.14, 287.42, 287.14, 287.18, 287.76, 286.35, 287.73, 286.83, 285.98, 288.02, 287.28, 286.16, 287.06, 288.12, 286.98, 286.83, 286.24]}, {array[312 elements], [107.79, 107.64, 106.9, 107.38, 106.8, 107.18, 106.66, 107.12, 106.47, 107.08, 106.74, 106.49, 106.74, 106.58, 106.34, 106.02, 106.44, 106.59, 106.12, 106.04, 105.82, 105.77, 105.86, 105.96, 105.31, 105.97, 105.25, 105.56, 105.29, 105.35, 105.28, 105.26, 105.33, 104.91, 105.39, 104.61, 104.88, 104.83, 104.39, 104.94, 104.32, 104.6, 104.16, 104.68, 104.0, 104.64, 104.18, 104.08, 104.46, 103.62, 103.94, 103.84, 103.65, 103.86, 103.28, 103.68, 103.34, 103.44, 103.46, 102.93, 103.64, 103.2, 103.09, 103.45, 102.6, 103.29, 102.82, 103.0, 102.67, 102.91, 102.47, 102.94, 102.11, 102.56, 102.2, 102.24, 102.24, 101.97, 102.17, 102.13, 102.0, 101.88, 101.67, 102.16, 101.36, 101.97, 101.23, 101.87, 101.11, 101.74, 101.04, 101.58, 101.22, 101.03, 101.16, 100.69, 101.37, 100.88, 100.82, 101.16, 100.41, 100.83, 100.32, 100.94, 100.42, 100.44, 100.75, 99.991, 100.26, 100.59, 99.936, 99.929, 100.3, 99.895, 99.831, 100.06, 99.818, 99.487, 99.678, 99.919, 99.587, 99.354, 99.367, 99.521, 99.53, 99.154, 98.888, 99.185, 98.947, 98.908, 98.955, 98.748, 98.776, 98.98, 98.564, 98.779, 98.72, 98.57, 98.567, 98.634, 98.027, 98.703, 97.978, 98.463, 97.938, 98.135, 98.077, 97.733, 98.121, 97.518, 98.207, 97.731, 97.754, 98.004, 97.257, 97.547, 97.814, 97.466, 97.089, 97.303, 97.647, 97.522, 97.419, 97.09, 96.973, 96.688, 96.826, 97.246, 97.049, 96.423, 96.707, 97.039, 96.293, 96.527, 96.561, 96.096, 96.643, 96.527, 95.957, 96.228, 96.519, 96.033, 95.733, 96.296, 96.336, 96.001, 95.996, 95.796, 95.784, 95.429, 95.301, 95.644, 95.81, 95.587, 95.232, 95.587, 95.41, 95.345, 95.303, 95.332, 95.134, 95.237, 95.119, 94.934, 95.311, 94.637, 94.658, 95.143, 94.762, 94.564, 94.832, 94.666, 94.555, 94.242, 94.259, 94.053, 94.162, 94.54, 94.517, 93.879, 94.07, 94.352, 93.972, 93.947, 94.272, 93.645, 93.823, 94.162, 93.416, 93.675, 93.733, 93.242, 93.456, 93.827, 93.802, 93.533, 93.423, 92.959, 93.082, 93.217, 93.308, 92.844, 93.147, 93.373, 92.734, 92.833, 93.12, 92.65, 92.866, 92.896, 92.317, 92.968, 92.234, 92.739, 92.158, 92.747, 92.093, 92.648, 92.007, 92.479, 92.313, 91.859, 92.176, 92.09, 91.683, 92.239, 91.932, 91.935, 91.84, 92.034, 91.637, 91.624, 91.873, 91.588, 91.384, 91.299, 91.115, 91.212, 91.61, 91.62, 91.206, 90.951, 90.877, 91.212, 91.424, 90.928, 90.671, 90.983, 90.909, 90.63, 90.892, 90.655, 90.726, 90.978, 90.368, 90.892, 90.199, 90.734, 90.144, 90.719, 90.353, 90.287, 90.622, 90.083, 89.966, 90.476, 90.1, 89.798, 90.189, 90.211, 90.11, 89.901]}, {array[312 elements], [285.22, 283.14, 283.7, 284.22, 282.94, 284.16, 283.12, 284.19, 283.77, 283.05, 284.75, 283.73, 284.03, 284.51, 284.36, 283.49, 282.81, 284.28, 284.63, 284.72, 284.28, 283.7, 283.06, 284.27, 283.77, 283.92, 283.05, 284.28, 282.64, 284.83, 283.27, 284.87, 282.69, 283.88, 283.65, 282.81, 284.65, 283.4, 283.89, 283.8, 282.66, 284.36, 282.73, 283.65, 283.53, 283.32, 284.39, 282.72, 284.12, 284.43, 283.06, 284.86, 282.72, 284.03, 283.2, 283.29, 284.36, 282.81, 284.39, 283.24, 283.09, 284.48, 282.45, 284.24, 283.85, 282.82, 283.89, 282.42, 283.97, 282.52, 283.97, 283.12, 283.14, 283.77, 282.22, 284.6, 282.69, 284.43, 283.21, 284.56, 282.24, 284.6, 282.15, 283.65, 283.61, 283.29, 283.49, 283.27, 283.56, 283.47, 283.35, 284.22, 282.37, 284.39, 282.72, 283.53, 283.53, 282.37, 283.7, 283.17, 282.39, 283.49, 282.34, 283.2, 283.27, 282.19, 283.52, 283.64, 282.1, 283.68, 283.97, 281.94, 282.93, 283.59, 282.72, 283.2, 283.92, 283.4, 282.13, 283.12, 283.92, 283.17, 282.46, 282.72, 283.09, 283.64, 282.88, 282.64, 284.28, 282.03, 284.04, 281.85, 284.15, 283.12, 282.66, 284.34, 281.94, 284.07, 281.85, 284.48, 282.82, 283.06, 283.05, 283.12, 283.97, 282.49, 284.04, 282.1, 283.37, 282.76, 282.49, 283.68, 281.86, 283.92, 283.4, 282.27, 283.09, 284.03, 283.2, 281.77, 282.69, 283.8, 283.88, 284.19, 283.24, 283.17, 281.38, 282.34, 283.73, 283.32, 281.82, 283.17, 283.7, 281.71, 283.41, 282.39, 281.64, 284.07, 283.06, 281.89, 282.54, 283.68, 282.18, 281.79, 283.47, 283.44, 284.22, 283.95, 283.85, 283.64, 282.61, 281.82, 282.72, 283.29, 282.85, 281.71, 283.95, 281.97, 283.89, 281.43, 283.89, 281.56, 284.1, 282.42, 282.76, 283.68, 281.67, 282.27, 283.49, 282.39, 282.37, 283.09, 283.73, 283.52, 282.82, 282.97, 281.38, 281.35, 283.49, 283.17, 281.16, 282.39, 283.06, 281.82, 282.57, 283.7, 281.89, 282.81, 283.2, 281.32, 282.97, 282.34, 281.2, 281.82, 282.76, 282.73, 283.64, 282.81, 282.27, 281.55, 282.49, 282.54, 281.11, 283.14, 283.8, 281.4, 282.61, 283.06, 281.4, 283.89, 282.39, 281.79, 282.78, 282.31, 283.41, 282.85, 282.57, 282.69, 282.52, 283.27, 281.28, 282.39, 282.78, 281.23, 282.88, 283.21, 281.59, 283.92, 281.49, 282.3, 282.85, 281.94, 282.64, 283.27, 283.61, 282.72, 282.52, 281.62, 281.49, 282.93, 283.41, 283.27, 281.77, 281.16, 282.69, 283.65, 281.91, 281.85, 283.32, 281.7, 282.78, 282.18, 283.49, 281.32, 282.45, 282.07, 282.07, 282.64, 282.52, 281.47, 283.41, 281.77, 282.42, 283.52, 281.38, 282.19, 283.64, 282.49, 281.35, 282.31, 282.69, 283.56]}, {array[312 elements], [274.45, 272.46, 276.98, 273.71, 276.19, 274.02, 276.37, 273.51, 276.45, 272.35, 274.14, 275.3, 273.26, 273.93, 276.9, 276.75, 273.51, 272.19, 274.23, 274.96, 275.72, 275.3, 274.33, 273.48, 276.87, 272.78, 275.9, 274.0, 274.93, 274.3, 274.48, 274.04, 272.81, 275.42, 272.24, 275.78, 274.45, 272.05, 276.33, 272.94, 275.49, 273.97, 275.8, 272.49, 276.4, 271.91, 274.26, 274.02, 271.8, 276.64, 273.9, 274.35, 274.99, 273.52, 276.36, 273.34, 275.38, 274.0, 273.67, 276.22, 271.9, 274.14, 273.89, 271.76, 276.52, 271.76, 274.56, 272.05, 274.51, 272.12, 275.06, 271.65, 276.26, 273.27, 274.62, 274.3, 273.38, 275.72, 273.65, 273.59, 273.45, 274.26, 274.51, 271.64, 276.36, 271.8, 275.96, 271.54, 275.94, 271.52, 275.51, 273.62, 273.67, 274.85, 273.3, 276.17, 271.59, 274.18, 274.41, 271.8, 275.82, 273.41, 275.39, 271.97, 274.79, 273.67, 271.45, 276.07, 273.86, 271.57, 275.03, 274.55, 272.38, 274.28, 274.02, 272.33, 273.69, 275.45, 273.82, 271.52, 273.2, 274.82, 274.14, 272.68, 272.05, 273.67, 274.92, 272.68, 274.3, 273.97, 273.59, 274.16, 274.35, 271.9, 274.44, 273.03, 272.56, 273.62, 272.96, 272.33, 275.33, 271.27, 275.23, 271.76, 275.0, 273.03, 273.31, 274.55, 272.35, 275.72, 270.91, 273.67, 272.85, 271.31, 275.65, 273.58, 271.43, 272.85, 275.42, 273.52, 270.73, 271.15, 271.65, 273.23, 273.59, 275.51, 273.93, 270.65, 271.61, 275.33, 273.19, 270.58, 275.12, 273.05, 272.24, 275.15, 271.64, 272.01, 273.93, 273.19, 270.66, 273.26, 275.23, 271.36, 270.8, 272.49, 272.22, 273.26, 273.05, 275.06, 275.39, 272.81, 271.54, 272.53, 274.62, 272.05, 272.45, 273.15, 272.61, 272.57, 272.92, 272.57, 272.39, 273.74, 270.66, 274.52, 274.35, 270.44, 272.75, 273.65, 271.83, 272.01, 272.53, 274.56, 273.86, 274.93, 274.07, 271.06, 270.88, 274.78, 273.59, 271.15, 273.41, 273.05, 270.66, 272.75, 273.27, 270.26, 275.0, 272.94, 271.69, 274.92, 273.26, 270.48, 270.19, 271.91, 272.22, 275.1, 273.85, 272.92, 271.64, 274.3, 272.31, 270.24, 274.07, 273.48, 271.17, 273.93, 272.22, 271.64, 274.96, 270.52, 275.19, 271.68, 274.82, 270.71, 274.96, 270.58, 274.92, 270.8, 272.33, 274.18, 271.86, 272.71, 274.96, 270.55, 272.96, 272.05, 272.57, 270.98, 272.99, 273.01, 270.98, 272.57, 273.59, 273.97, 274.85, 274.11, 270.71, 270.41, 272.75, 274.45, 274.4, 272.12, 270.14, 273.1, 274.71, 272.71, 272.35, 274.37, 271.68, 273.74, 272.18, 270.55, 274.16, 270.39, 274.93, 270.59, 274.51, 270.84, 272.71, 272.99, 270.32, 273.45, 274.16, 270.02, 272.38, 274.23, 273.15, 270.66, 271.09, 272.5]}, {array[312 elements], []}]
  out "LSI-D Grpah 2":cluster{dbl[], dbl[]}[](graph)=[{array[312 elements], [0.0, 296.61, 296.59, 296.63, 296.62, 296.61, 296.61, 296.61, 296.61, 296.61, 296.57, 296.65, 296.6, 296.66, 296.59, 296.6, 296.58, 296.64, 296.63, 296.66, 296.57, 296.61, 296.6, 296.6, 296.61, 296.61, 296.6, 296.6, 296.57, 296.62, 296.58, 296.59, 296.58, 296.61, 296.62, 296.57, 296.61, 296.63, 296.62, 296.64, 296.63, 296.6, 296.6, 296.57, 296.59, 296.59, 296.6, 296.59, 296.56, 296.6, 296.59, 296.61, 296.59, 296.58, 296.57, 296.59, 296.62, 296.59, 296.61, 296.6, 296.55, 296.6, 296.59, 296.59, 296.6, 296.61, 296.59, 296.57, 296.64, 296.67, 296.57, 296.62, 296.57, 296.58, 296.62, 296.61, 296.58, 296.55, 296.56, 296.59, 296.59, 296.6, 296.58, 296.57, 296.61, 296.58, 296.53, 296.54, 296.59, 296.55, 296.53, 296.59, 296.58, 296.58, 296.58, 296.55, 296.56, 296.56, 296.59, 296.53, 296.61, 296.62, 296.6, 296.58, 296.56, 296.53, 296.55, 296.59, 296.58, 296.6, 296.55, 296.59, 296.56, 296.56, 296.58, 296.57, 296.61, 296.55, 296.61, 296.57, 296.57, 296.58, 296.51, 296.55, 296.6, 296.6, 296.58, 296.56, 296.58, 296.57, 296.59, 296.55, 296.55, 296.56, 296.59, 296.52, 296.54, 296.58, 296.52, 296.54, 296.57, 296.54, 296.59, 296.52, 296.53, 296.55, 296.49, 296.54, 296.63, 296.56, 296.53, 296.54, 296.55, 296.58, 296.56, 296.51, 296.55, 296.57, 296.53, 296.52, 296.56, 296.58, 296.55, 296.61, 296.55, 296.58, 296.53, 296.58, 296.57, 296.52, 296.48, 296.53, 296.52, 296.54, 296.59, 296.53, 296.56, 296.55, 296.58, 296.56, 296.51, 296.52, 296.57, 296.54, 296.55, 296.55, 296.57, 296.59, 296.6, 296.55, 296.54, 296.51, 296.52, 296.55, 296.55, 296.54, 296.51, 296.49, 296.57, 296.55, 296.54, 296.56, 296.55, 296.53, 296.5, 296.55, 296.53, 296.54, 296.57, 296.52, 296.55, 296.55, 296.52, 296.5, 296.53, 296.53, 296.52, 296.54, 296.53, 296.52, 296.53, 296.51, 296.58, 296.49, 296.52, 296.55, 296.48, 296.51, 296.55, 296.48, 296.55, 296.5, 296.51, 296.55, 296.52, 296.54, 296.5, 296.54, 296.52, 296.53, 296.55, 296.53, 296.48, 296.58, 296.55, 296.52, 296.51, 296.49, 296.53, 296.5, 296.56, 296.53, 296.48, 296.54, 296.52, 296.56, 296.53, 296.5, 296.51, 296.5, 296.51, 296.47, 296.47, 296.57, 296.53, 296.49, 296.56, 296.55, 296.55, 296.51, 296.5, 296.52, 296.52, 296.48, 296.51, 296.54, 296.5, 296.49, 296.55, 296.5, 296.52, 296.54, 296.5, 296.51, 296.5, 296.53, 296.49, 296.51, 296.49, 296.54, 296.5, 296.51, 296.5, 296.54, 296.5, 296.48, 296.46, 296.5, 296.49, 296.49, 296.49, 296.51, 296.47, 296.49, 296.47, 296.49, 296.47, 296.49, 296.46, 296.49, 296.47, 296.51]}, {array[312 elements], [0.0, 246.36, 246.3, 246.25, 246.18, 246.13, 246.13, 246.1, 246.04, 246.01, 245.96, 245.88, 245.85, 245.76, 245.73, 245.71, 245.65, 245.59, 245.54, 245.5, 245.46, 245.41, 245.35, 245.32, 245.31, 245.24, 245.17, 245.15, 245.05, 245.05, 244.99, 244.94, 244.92, 244.85, 244.84, 244.72, 244.69, 244.62, 244.56, 244.56, 244.49, 244.46, 244.4, 244.4, 244.3, 244.3, 244.25, 244.17, 244.13, 244.08, 244.03, 243.99, 243.95, 243.89, 243.86, 243.79, 243.75, 243.69, 243.65, 243.6, 243.56, 243.49, 243.42, 243.43, 243.36, 243.34, 243.27, 243.21, 243.12, 243.17, 243.07, 243.05, 242.97, 242.87, 242.88, 242.8, 242.77, 242.72, 242.65, 242.64, 242.55, 242.51, 242.45, 242.46, 242.37, 242.29, 242.28, 242.21, 242.18, 242.14, 242.06, 242.07, 242.0, 241.92, 241.91, 241.84, 241.77, 241.71, 241.66, 241.64, 241.57, 241.52, 241.46, 241.4, 241.37, 241.32, 241.26, 241.23, 241.17, 241.15, 241.07, 241.0, 240.93, 240.92, 240.86, 240.78, 240.76, 240.7, 240.65, 240.57, 240.51, 240.46, 240.46, 240.37, 240.33, 240.29, 240.19, 240.16, 240.13, 240.09, 240.0, 239.96, 239.91, 239.87, 239.83, 239.75, 239.71, 239.63, 239.57, 239.52, 239.48, 239.39, 239.35, 239.35, 239.29, 239.2, 239.19, 239.07, 239.04, 239.02, 238.97, 238.87, 238.8, 238.79, 238.73, 238.67, 238.61, 238.57, 238.54, 238.45, 238.38, 238.36, 238.28, 238.24, 238.21, 238.17, 238.09, 238.05, 237.98, 237.95, 237.88, 237.82, 237.8, 237.73, 237.64, 237.6, 237.58, 237.52, 237.49, 237.43, 237.33, 237.29, 237.26, 237.22, 237.17, 237.11, 237.06, 237.01, 236.97, 236.91, 236.84, 236.8, 236.75, 236.69, 236.64, 236.56, 236.53, 236.45, 236.43, 236.38, 236.33, 236.28, 236.23, 236.16, 236.13, 236.07, 236.01, 235.93, 235.93, 235.88, 235.82, 235.78, 235.72, 235.63, 235.6, 235.57, 235.52, 235.47, 235.43, 235.34, 235.32, 235.25, 235.23, 235.16, 235.11, 235.07, 235.02, 234.92, 234.93, 234.85, 234.8, 234.75, 234.71, 234.65, 234.62, 234.52, 234.5, 234.47, 234.42, 234.38, 234.32, 234.23, 234.19, 234.14, 234.08, 234.06, 234.03, 233.95, 233.91, 233.85, 233.79, 233.74, 233.73, 233.68, 233.61, 233.58, 233.51, 233.46, 233.41, 233.36, 233.32, 233.27, 233.24, 233.16, 233.11, 233.11, 233.03, 232.95, 232.9, 232.89, 232.8, 232.8, 232.72, 232.69, 232.65, 232.58, 232.52, 232.5, 232.44, 232.38, 232.34, 232.26, 232.21, 232.17, 232.13, 232.11, 232.03, 231.97, 231.96, 231.91, 231.88, 231.82, 231.77, 231.7, 231.65, 231.59, 231.59, 231.49, 231.49, 231.38, 231.35, 231.31, 231.25, 231.21, 231.19, 231.16, 231.09, 230.99, 230.97, 230.95, 230.89, 230.81]}, {array[312 elements], [0.0, 251.98, 251.95, 251.89, 251.86, 251.82, 251.77, 251.73, 251.67, 251.64, 251.61, 251.56, 251.51, 251.45, 251.42, 251.36, 251.34, 251.3, 251.22, 251.19, 251.19, 251.14, 251.06, 251.04, 250.98, 250.95, 250.91, 250.87, 250.82, 250.77, 250.74, 250.67, 250.65, 250.6, 250.55, 250.52, 250.46, 250.41, 250.37, 250.34, 250.28, 250.24, 250.21, 250.15, 250.11, 250.08, 250.04, 249.99, 249.94, 249.87, 249.85, 249.81, 249.77, 249.73, 249.67, 249.63, 249.58, 249.55, 249.48, 249.47, 249.4, 249.35, 249.32, 249.28, 249.25, 249.19, 249.15, 249.1, 249.05, 249.01, 248.98, 248.92, 248.85, 248.82, 248.79, 248.76, 248.71, 248.65, 248.6, 248.55, 248.52, 248.47, 248.44, 248.38, 248.36, 248.3, 248.26, 248.19, 248.13, 248.12, 248.06, 248.03, 247.98, 247.93, 247.86, 247.85, 247.82, 247.74, 247.7, 247.66, 247.63, 247.58, 247.54, 247.48, 247.43, 247.4, 247.33, 247.3, 247.25, 247.2, 247.16, 247.1, 247.09, 247.02, 246.96, 246.93, 246.88, 246.85, 246.79, 246.76, 246.7, 246.66, 246.6, 246.58, 246.53, 246.47, 246.44, 246.4, 246.34, 246.28, 246.23, 246.18, 246.14, 246.1, 246.05, 246.01, 245.98, 245.94, 245.86, 245.85, 245.79, 245.72, 245.68, 245.65, 245.62, 245.54, 245.52, 245.46, 245.42, 245.37, 245.3, 245.28, 245.23, 245.15, 245.13, 245.08, 245.03, 244.97, 244.94, 244.89, 244.87, 244.8, 244.75, 244.71, 244.65, 244.62, 244.59, 244.53, 244.48, 244.4, 244.38, 244.32, 244.29, 244.25, 244.18, 244.15, 244.11, 244.06, 244.03, 243.93, 243.92, 243.85, 243.82, 243.75, 243.73, 243.67, 243.63, 243.57, 243.52, 243.49, 243.44, 243.38, 243.33, 243.29, 243.25, 243.21, 243.15, 243.11, 243.06, 243.0, 242.97, 242.92, 242.86, 242.83, 242.76, 242.74, 242.67, 242.61, 242.58, 242.55, 242.47, 242.45, 242.39, 242.34, 242.3, 242.25, 242.21, 242.16, 242.12, 242.06, 242.01, 241.94, 241.91, 241.86, 241.82, 241.76, 241.71, 241.67, 241.59, 241.56, 241.5, 241.48, 241.42, 241.38, 241.33, 241.29, 241.22, 241.18, 241.15, 241.09, 241.05, 241.0, 240.93, 240.9, 240.85, 240.8, 240.75, 240.71, 240.65, 240.62, 240.55, 240.52, 240.47, 240.41, 240.36, 240.3, 240.28, 240.21, 240.17, 240.11, 240.07, 240.03, 239.98, 239.93, 239.88, 239.83, 239.8, 239.73, 239.67, 239.63, 239.6, 239.54, 239.5, 239.42, 239.41, 239.36, 239.3, 239.24, 239.21, 239.16, 239.11, 239.04, 239.01, 238.94, 238.9, 238.85, 238.81, 238.76, 238.7, 238.67, 238.62, 238.56, 238.51, 238.48, 238.41, 238.38, 238.33, 238.28, 238.24, 238.17, 238.12, 238.07, 238.03, 237.95, 237.93, 237.88, 237.85, 237.78, 237.73, 237.68, 237.64, 237.57]}, {array[312 elements], [0.0, 22.529, 22.52, 22.516, 22.495, 22.486, 22.467, 22.467, 22.454, 22.443, 22.422, 22.419, 22.404, 22.383, 22.383, 22.362, 22.365, 22.347, 22.331, 22.329, 22.31, 22.305, 22.302, 22.294, 22.273, 22.277, 22.26, 22.241, 22.238, 22.231, 22.225, 22.194, 22.193, 22.182, 22.171, 22.163, 22.164, 22.165, 22.157, 22.138, 22.136, 22.124, 22.112, 22.109, 22.094, 22.078, 22.077, 22.076, 22.066, 22.067, 22.046, 22.048, 22.04, 22.032, 22.017, 22.004, 21.995, 21.997, 21.999, 21.975, 21.967, 21.961, 21.956, 21.949, 21.941, 21.93, 21.929, 21.91, 21.917, 21.916, 21.899, 21.888, 21.886, 21.878, 21.864, 21.846, 21.845, 21.839, 21.831, 21.821, 21.814, 21.797, 21.805, 21.796, 21.795, 21.776, 21.766, 21.78, 21.769, 21.767, 21.756, 21.738, 21.753, 21.729, 21.736, 21.73, 21.716, 21.707, 21.704, 21.702, 21.703, 21.689, 21.682, 21.682, 21.674, 21.661, 21.655, 21.66, 21.656, 21.646, 21.647, 21.634, 21.63, 21.626, 21.613, 21.616, 21.604, 21.603, 21.602, 21.592, 21.593, 21.589, 21.579, 21.575, 21.568, 21.561, 21.555, 21.557, 21.547, 21.541, 21.535, 21.531, 21.532, 21.53, 21.526, 21.523, 21.509, 21.503, 21.509, 21.501, 21.491, 21.505, 21.496, 21.496, 21.482, 21.483, 21.483, 21.473, 21.478, 21.485, 21.47, 21.473, 21.461, 21.459, 21.454, 21.442, 21.453, 21.462, 21.462, 21.456, 21.445, 21.445, 21.453, 21.457, 21.449, 21.449, 21.442, 21.447, 21.444, 21.446, 21.443, 21.446, 21.446, 21.449, 21.446, 21.449, 21.45, 21.455, 21.45, 21.446, 21.444, 21.442, 21.451, 21.44, 21.433, 21.45, 21.432, 21.441, 21.441, 21.44, 21.443, 21.43, 21.424, 21.421, 21.42, 21.43, 21.427, 21.416, 21.405, 21.406, 21.406, 21.414, 21.404, 21.417, 21.414, 21.406, 21.393, 21.401, 21.4, 21.393, 21.38, 21.369, 21.372, 21.379, 21.364, 21.376, 21.364, 21.347, 21.35, 21.365, 21.361, 21.346, 21.335, 21.349, 21.336, 21.321, 21.336, 21.331, 21.342, 21.335, 21.31, 21.331, 21.314, 21.324, 21.317, 21.292, 21.316, 21.282, 21.305, 21.298, 21.3, 21.286, 21.291, 21.278, 21.282, 21.28, 21.276, 21.255, 21.262, 21.269, 21.256, 21.241, 21.245, 21.239, 21.225, 21.233, 21.228, 21.23, 21.218, 21.218, 21.211, 21.215, 21.212, 21.213, 21.21, 21.2, 21.209, 21.204, 21.188, 21.2, 21.185, 21.18, 21.181, 21.166, 21.162, 21.166, 21.161, 21.139, 21.152, 21.143, 21.138, 21.131, 21.138, 21.133, 21.132, 21.123, 21.12, 21.119, 21.114, 21.107, 21.108, 21.1, 21.089, 21.091, 21.082, 21.083, 21.083, 21.073, 21.072, 21.059, 21.055, 21.048, 21.04, 21.044, 21.035, 21.02, 21.025, 21.009, 21.019, 21.009, 21.001, 20.995]}, {array[312 elements], [0.0, 4.244, 4.243, 4.243, 4.243, 4.243, 4.243, 4.243, 4.243, 4.243, 4.243, 4.243, 4.243, 4.243, 4.242, 4.243, 4.243, 4.243, 4.243, 4.242, 4.244, 4.243, 4.244, 4.243, 4.242, 4.243, 4.243, 4.243, 4.243, 4.243, 4.243, 4.243, 4.243, 4.243, 4.243, 4.243, 4.243, 4.243, 4.243, 4.243, 4.244, 4.244, 4.243, 4.243, 4.243, 4.244, 4.243, 4.243, 4.243, 4.243, 4.243, 4.243, 4.242, 4.243, 4.243, 4.243, 4.243, 4.243, 4.243, 4.243, 4.243, 4.243, 4.243, 4.243, 4.243, 4.243, 4.242, 4.243, 4.243, 4.242, 4.242, 4.242, 4.243, 4.243, 4.242, 4.243, 4.243, 4.242, 4.243, 4.243, 4.242, 4.243, 4.243, 4.243, 4.243, 4.243, 4.242, 4.243, 4.242, 4.242, 4.243, 4.243, 4.243, 4.242, 4.242, 4.243, 4.243, 4.242, 4.242, 4.242, 4.242, 4.242, 4.243, 4.243, 4.243, 4.243, 4.243, 4.243, 4.243, 4.243, 4.243, 4.242, 4.243, 4.243, 4.243, 4.242, 4.243, 4.242, 4.243, 4.243, 4.243, 4.243, 4.242, 4.242, 4.242, 4.243, 4.242, 4.243, 4.243, 4.242, 4.242, 4.242, 4.242, 4.242, 4.243, 4.243, 4.243, 4.242, 4.242, 4.242, 4.242, 4.243, 4.242, 4.242, 4.242, 4.242, 4.242, 4.242, 4.242, 4.243, 4.243, 4.242, 4.242, 4.242, 4.242, 4.242, 4.243, 4.242, 4.243, 4.243, 4.242, 4.242, 4.242, 4.242, 4.242, 4.243, 4.242, 4.243, 4.243, 4.243, 4.242, 4.243, 4.242, 4.243, 4.243, 4.242, 4.242, 4.242, 4.242, 4.242, 4.242, 4.242, 4.242, 4.242, 4.242, 4.242, 4.242, 4.242, 4.242, 4.242, 4.242, 4.242, 4.243, 4.242, 4.242, 4.242, 4.243, 4.242, 4.242, 4.242, 4.242, 4.242, 4.243, 4.242, 4.242, 4.242, 4.242, 4.242, 4.242, 4.242, 4.242, 4.242, 4.242, 4.242, 4.243, 4.242, 4.242, 4.242, 4.242, 4.241, 4.242, 4.242, 4.242, 4.242, 4.242, 4.242, 4.242, 4.242, 4.243, 4.242, 4.242, 4.242, 4.242, 4.242, 4.242, 4.242, 4.243, 4.242, 4.242, 4.242, 4.242, 4.241, 4.242, 4.242, 4.242, 4.242, 4.242, 4.242, 4.242, 4.242, 4.242, 4.243, 4.242, 4.242, 4.242, 4.242, 4.242, 4.242, 4.242, 4.242, 4.242, 4.242, 4.242, 4.241, 4.242, 4.241, 4.242, 4.242, 4.242, 4.242, 4.242, 4.242, 4.241, 4.241, 4.242, 4.242, 4.241, 4.241, 4.241, 4.242, 4.241, 4.242, 4.242, 4.242, 4.242, 4.242, 4.242, 4.242, 4.242, 4.242, 4.242, 4.242, 4.242, 4.241, 4.242, 4.242, 4.241, 4.242, 4.242, 4.242, 4.242, 4.241, 4.242, 4.241, 4.242, 4.242, 4.241, 4.242, 4.242, 4.241, 4.242, 4.242]}, {array[312 elements], [0.0, 6.751, 6.741, 6.737, 6.736, 6.748, 6.752, 6.743, 6.739, 6.737, 6.744, 6.752, 6.753, 6.747, 6.741, 6.737, 6.737, 6.741, 6.748, 6.755, 6.756, 6.755, 6.75, 6.748, 6.745, 6.744, 6.743, 6.746, 6.75, 6.755, 6.761, 6.761, 6.758, 6.752, 6.75, 6.747, 6.747, 6.745, 6.745, 6.747, 6.753, 6.756, 6.764, 6.764, 6.763, 6.76, 6.755, 6.754, 6.752, 6.752, 6.752, 6.752, 6.751, 6.751, 6.751, 6.751, 6.753, 6.757, 6.759, 6.76, 6.764, 6.766, 6.766, 6.77, 6.771, 6.769, 6.77, 6.769, 6.769, 6.769, 6.767, 6.768, 6.764, 6.764, 6.763, 6.759, 6.76, 6.759, 6.758, 6.759, 6.76, 6.762, 6.762, 6.763, 6.765, 6.767, 6.769, 6.771, 6.774, 6.779, 6.78, 6.78, 6.782, 6.782, 6.781, 6.777, 6.775, 6.772, 6.77, 6.768, 6.768, 6.771, 6.773, 6.773, 6.777, 6.78, 6.786, 6.788, 6.787, 6.78, 6.776, 6.773, 6.774, 6.776, 6.78, 6.786, 6.789, 6.79, 6.785, 6.776, 6.775, 6.778, 6.781, 6.788, 6.793, 6.79, 6.78, 6.775, 6.778, 6.782, 6.79, 6.794, 6.789, 6.78, 6.78, 6.782, 6.786, 6.795, 6.796, 6.788, 6.782, 6.784, 6.787, 6.794, 6.8, 6.792, 6.785, 6.788, 6.797, 6.802, 6.796, 6.785, 6.786, 6.79, 6.802, 6.8, 6.788, 6.789, 6.794, 6.804, 6.804, 6.792, 6.791, 6.795, 6.804, 6.804, 6.793, 6.792, 6.795, 6.803, 6.807, 6.796, 6.792, 6.797, 6.807, 6.8, 6.792, 6.799, 6.808, 6.797, 6.793, 6.803, 6.81, 6.794, 6.798, 6.809, 6.807, 6.797, 6.802, 6.812, 6.807, 6.816, 6.829, 6.84, 6.828, 6.828, 6.838, 6.838, 6.826, 6.831, 6.843, 6.831, 6.83, 6.84, 6.841, 6.828, 6.835, 6.846, 6.831, 6.833, 6.846, 6.839, 6.834, 6.842, 6.843, 6.833, 6.842, 6.849, 6.833, 6.843, 6.849, 6.834, 6.842, 6.85, 6.835, 6.843, 6.848, 6.836, 6.842, 6.849, 6.837, 6.848, 6.848, 6.839, 6.851, 6.846, 6.84, 6.85, 6.844, 6.841, 6.853, 6.84, 6.844, 6.856, 6.841, 6.845, 6.857, 6.84, 6.85, 6.85, 6.843, 6.856, 6.847, 6.845, 6.858, 6.844, 6.848, 6.858, 6.846, 6.858, 6.843, 6.852, 6.852, 6.846, 6.859, 6.845, 6.853, 6.853, 6.848, 6.86, 6.846, 6.858, 6.847, 6.852, 6.854, 6.849, 6.863, 6.848, 6.861, 6.847, 6.856, 6.855, 6.852, 6.861, 6.85, 6.864, 6.848, 6.863, 6.85, 6.854, 6.859, 6.851, 6.865, 6.851, 6.865, 6.851, 6.864, 6.853, 6.859, 6.855, 6.859, 6.862, 6.857, 6.867, 6.856, 6.869, 6.856, 6.87, 6.855, 6.871, 6.855, 6.869]}, {array[312 elements], [0.0, 295.97, 296.04, 295.97, 296.06, 295.86, 295.93, 296.04, 295.99, 296.15, 295.97, 296.14, 296.11, 296.03, 296.06, 296.03, 296.11, 296.2, 295.93, 296.04, 295.99, 296.02, 295.99, 296.1, 296.14, 295.73, 296.02, 296.15, 296.14, 295.92, 296.02, 296.15, 296.0, 296.04, 296.15, 296.25, 296.31, 296.02, 296.13, 296.22, 296.37, 296.22, 296.27, 296.35, 296.13, 296.22, 295.7, 296.18, 295.95, 296.22, 296.39, 296.14, 296.25, 296.1, 296.15, 296.13, 296.2, 296.14, 296.23, 296.2, 296.2, 296.06, 296.18, 296.27, 296.42, 296.31, 296.31, 296.31, 296.11, 296.22, 296.16, 296.23, 296.33, 296.14, 296.06, 296.43, 296.31, 296.2, 296.16, 296.13, 296.4, 296.23, 296.5, 296.4, 296.31, 296.1, 296.51, 296.42, 296.37, 296.43, 296.4, 296.31, 296.27, 296.54, 296.36, 296.27, 296.44, 296.35, 296.27, 296.42, 296.22, 296.43, 296.31, 296.54, 296.55, 296.4, 296.39, 296.31, 296.33, 296.5, 296.5, 296.44, 296.53, 296.47, 296.36, 296.49, 296.44, 296.58, 296.36, 296.31, 296.47, 296.49, 296.25, 296.47, 296.66, 296.51, 296.4, 296.49, 296.49, 296.18, 296.47, 296.56, 296.51, 296.55, 296.62, 296.6, 296.6, 296.47, 296.47, 296.58, 296.63, 296.58, 296.58, 296.56, 296.6, 296.47, 296.42, 296.37, 296.42, 296.49, 296.37, 296.53, 296.5, 296.6, 296.56, 296.63, 296.71, 296.58, 296.51, 296.43, 296.77, 296.36, 296.63, 296.44, 296.73, 296.73, 296.6, 296.74, 296.5, 296.51, 296.5, 296.42, 296.65, 296.58, 296.4, 296.31, 296.53, 296.43, 296.69, 296.66, 296.65, 296.62, 296.71, 296.6, 296.35, 296.7, 296.65, 296.6, 296.67, 296.63, 296.78, 296.91, 296.86, 296.69, 296.74, 296.55, 296.6, 296.91, 296.76, 296.67, 296.76, 296.71, 296.94, 296.63, 296.86, 296.63, 296.7, 296.82, 296.8, 296.74, 296.74, 296.73, 296.96, 296.76, 296.74, 296.8, 296.84, 296.86, 296.83, 296.77, 296.89, 296.65, 296.77, 296.84, 296.71, 296.76, 296.74, 296.89, 296.8, 296.74, 296.82, 296.87, 296.8, 297.0, 297.16, 297.09, 296.98, 296.83, 296.89, 296.89, 296.54, 296.89, 296.78, 296.87, 297.21, 297.14, 296.78, 296.73, 296.87, 297.14, 297.03, 297.14, 297.1, 297.09, 297.02, 296.78, 297.25, 297.21, 297.0, 297.03, 296.98, 296.94, 296.93, 296.93, 297.03, 297.07, 296.89, 297.05, 297.02, 296.98, 296.95, 296.96, 296.87, 296.95, 297.07, 297.13, 296.96, 297.07, 297.0, 297.16, 297.17, 297.05, 296.93, 296.91, 297.07, 296.98, 297.1, 297.03, 297.19, 297.05, 297.0, 297.07, 297.16, 297.13, 297.0, 297.21, 296.94, 297.3, 297.05, 297.12, 297.28, 297.21, 297.17, 297.23, 297.25, 297.25, 297.21, 297.21, 297.13, 297.17, 297.29, 297.3]}, {array[312 elements], [0.0, 281.87, 284.61, 281.99, 283.5, 282.29, 284.54, 281.98, 283.46, 284.72, 281.54, 282.9, 285.03, 283.14, 281.87, 281.54, 283.76, 284.61, 283.77, 283.35, 282.81, 281.49, 282.64, 284.24, 282.04, 283.31, 281.38, 284.43, 281.46, 284.59, 281.26, 283.93, 282.21, 282.76, 283.46, 282.65, 284.47, 281.69, 284.72, 282.51, 283.24, 282.89, 283.52, 281.43, 284.24, 281.77, 282.2, 284.47, 282.72, 282.56, 284.67, 281.3, 283.69, 282.76, 281.24, 284.17, 281.24, 283.14, 282.61, 281.26, 283.55, 282.98, 281.62, 283.87, 282.12, 282.56, 284.26, 281.95, 284.13, 281.11, 283.82, 280.96, 283.39, 282.37, 281.73, 283.39, 282.29, 283.76, 282.07, 283.87, 282.21, 282.35, 283.01, 281.11, 284.39, 281.29, 283.77, 281.26, 283.8, 280.91, 284.29, 281.18, 283.31, 281.79, 284.37, 282.32, 283.14, 282.61, 282.51, 283.77, 281.74, 283.06, 281.43, 284.09, 282.35, 281.98, 284.26, 282.65, 281.95, 284.88, 283.01, 281.07, 284.18, 283.55, 281.3, 282.68, 283.9, 283.11, 281.65, 282.59, 283.47, 283.01, 282.43, 281.41, 282.95, 284.1, 282.89, 281.13, 284.54, 282.24, 282.72, 282.68, 283.46, 281.74, 283.85, 283.03, 282.64, 283.01, 283.11, 282.17, 283.87, 281.82, 284.02, 282.12, 283.16, 284.39, 281.65, 284.13, 281.21, 283.47, 283.72, 281.49, 282.76, 284.77, 282.15, 282.4, 283.52, 284.13, 283.31, 282.28, 281.85, 282.9, 283.9, 284.29, 284.54, 284.51, 283.85, 283.03, 283.11, 283.9, 284.51, 282.98, 283.47, 284.67, 281.99, 282.53, 284.42, 283.31, 282.15, 284.8, 283.93, 281.66, 283.11, 284.8, 282.9, 283.35, 283.39, 282.61, 283.16, 281.73, 281.38, 283.76, 284.81, 284.81, 283.5, 283.01, 284.72, 282.53, 284.64, 282.83, 284.24, 282.83, 283.8, 283.82, 282.04, 284.13, 284.13, 282.59, 283.42, 285.13, 282.59, 281.99, 283.31, 282.32, 282.95, 283.16, 283.39, 284.54, 284.42, 281.66, 282.61, 284.39, 282.98, 281.54, 285.03, 283.38, 282.56, 284.72, 283.08, 282.76, 284.47, 283.08, 282.64, 283.8, 284.88, 284.61, 284.73, 283.63, 281.79, 281.54, 283.24, 283.27, 281.66, 282.61, 283.93, 284.39, 282.37, 283.39, 284.67, 281.91, 284.59, 283.38, 281.82, 284.96, 282.2, 284.88, 281.73, 284.09, 281.74, 285.05, 282.2, 282.45, 284.01, 281.18, 282.9, 282.48, 283.52, 282.98, 283.22, 282.32, 284.13, 283.85, 281.11, 282.37, 284.59, 284.8, 284.59, 282.98, 282.07, 282.28, 282.83, 283.72, 283.38, 282.83, 282.07, 283.01, 282.78, 283.3, 281.49, 283.06, 282.21, 283.39, 281.85, 283.22, 282.28, 283.42, 282.95, 283.64, 281.33, 284.77, 282.29, 282.12, 283.69, 284.05, 281.74, 283.08, 283.72, 282.59, 281.43, 282.59, 282.81, 283.3]}, {array[312 elements], []}]
  out "LSI-U Grpah 3":cluster{dbl[], dbl[]}[](graph)=[{array[312 elements], [286.85, 286.84, 286.82, 286.84, 286.77, 286.76, 286.74, 286.79, 286.78, 286.78, 286.83, 286.73, 286.76, 286.74, 286.76, 286.75, 286.72, 286.77, 286.72, 286.69, 286.75, 286.7, 286.68, 286.7, 286.64, 286.69, 286.65, 286.68, 286.7, 286.67, 286.64, 286.62, 286.64, 286.63, 286.64, 286.62, 286.6, 286.61, 286.63, 286.61, 286.59, 286.61, 286.59, 286.59, 286.59, 286.59, 286.54, 286.56, 286.54, 286.52, 286.56, 286.54, 286.54, 286.51, 286.51, 286.49, 286.53, 286.47, 286.51, 286.51, 286.5, 286.48, 286.47, 286.44, 286.47, 286.46, 286.46, 286.43, 286.41, 286.39, 286.43, 286.41, 286.4, 286.38, 286.4, 286.39, 286.36, 286.42, 286.38, 286.32, 286.36, 286.32, 286.37, 286.36, 286.3, 286.34, 286.33, 286.33, 286.31, 286.25, 286.27, 286.24, 286.28, 286.3, 286.31, 286.26, 286.26, 286.22, 286.23, 286.25, 286.23, 286.26, 286.2, 286.21, 286.22, 286.22, 286.2, 286.19, 286.19, 286.15, 286.18, 286.19, 286.17, 286.16, 286.17, 286.18, 286.15, 286.13, 286.17, 286.1, 286.08, 286.1, 286.14, 286.08, 286.11, 286.07, 286.08, 286.06, 286.08, 286.09, 286.04, 286.02, 286.03, 286.05, 286.01, 286.04, 286.04, 286.01, 286.01, 286.0, 285.98, 286.03, 286.0, 285.97, 285.98, 285.97, 286.0, 285.99, 285.91, 285.91, 285.89, 285.96, 285.95, 285.94, 285.93, 285.9, 285.89, 285.88, 285.89, 285.91, 285.88, 285.87, 285.85, 285.84, 285.84, 285.86, 285.84, 285.82, 285.81, 285.81, 285.79, 285.81, 285.81, 285.8, 285.77, 285.76, 285.81, 285.77, 285.79, 285.73, 285.76, 285.72, 285.71, 285.75, 285.71, 285.71, 285.73, 285.69, 285.74, 285.71, 285.7, 285.7, 285.64, 285.66, 285.63, 285.67, 285.69, 285.64, 285.63, 285.62, 285.63, 285.63, 285.61, 285.56, 285.55, 285.57, 285.57, 285.56, 285.55, 285.58, 285.54, 285.56, 285.52, 285.54, 285.55, 285.5, 285.54, 285.49, 285.51, 285.46, 285.45, 285.5, 285.52, 285.46, 285.47, 285.49, 285.47, 285.47, 285.42, 285.44, 285.42, 285.4, 285.41, 285.46, 285.4, 285.37, 285.39, 285.36, 285.37, 285.37, 285.37, 285.36, 285.39, 285.31, 285.32, 285.35, 285.29, 285.3, 285.29, 285.33, 285.3, 285.31, 285.28, 285.26, 285.29, 285.26, 285.22, 285.23, 285.23, 285.22, 285.28, 285.23, 285.2, 285.19, 285.2, 285.2, 285.16, 285.22, 285.18, 285.18, 285.17, 285.14, 285.13, 285.12, 285.13, 285.11, 285.16, 285.16, 285.1, 285.11, 285.09, 285.08, 285.09, 285.07, 285.08, 285.08, 285.05, 285.05, 285.02, 285.05, 285.05, 284.99, 285.04, 285.01, 285.01, 284.97, 284.99, 285.0, 284.95, 284.98, 284.95, 284.99, 284.94, 284.93, 284.92, 284.92, 284.91, 284.93, 284.88, 284.91, 284.9, 284.87]}, {array[312 elements], [0.0, 0.0, 0.0, 0.0, 0.0, 0.0, 0.0, 0.0, 0.0, 0.0, 0.0, 0.0, 0.0, 0.0, 0.0, 0.0, 0.0, 0.0, 0.0, 0.0, 0.0, 0.0, 0.0, 0.0, 0.0, 0.0, 0.0, 0.0, 0.0, 0.0, 0.0, 0.0, 0.0, 0.0, 0.0, 0.0, 0.0, 0.0, 0.0, 0.0, 0.0, 0.0, 0.0, 0.0, 0.0, 0.0, 0.0, 0.0, 0.0, 0.0, 0.0, 0.0, 0.0, 0.0, 0.0, 0.0, 0.0, 0.0, 0.0, 0.0, 0.0, 0.0, 0.0, 0.0, 0.0, 0.0, 0.0, 0.0, 0.0, 0.0, 0.0, 0.0, 0.0, 0.0, 0.0, 0.0, 0.0, 0.0, 0.0, 0.0, 0.0, 0.0, 0.0, 0.0, 0.0, 0.0, 0.0, 0.0, 0.0, 0.0, 0.0, 0.0, 0.0, 0.0, 0.0, 0.0, 0.0, 0.0, 0.0, 0.0, 0.0, 0.0, 0.0, 0.0, 0.0, 0.0, 0.0, 0.0, 0.0, 0.0, 0.0, 0.0, 0.0, 0.0, 0.0, 0.0, 0.0, 0.0, 0.0, 0.0, 0.0, 0.0, 0.0, 0.0, 0.0, 0.0, 0.0, 0.0, 0.0, 0.0, 0.0, 0.0, 0.0, 0.0, 0.0, 0.0, 0.0, 0.0, 0.0, 0.0, 0.0, 0.0, 0.0, 0.0, 0.0, 0.0, 0.0, 0.0, 0.0, 0.0, 0.0, 0.0, 0.0, 0.0, 0.0, 0.0, 0.0, 0.0, 0.0, 0.0, 0.0, 0.0, 0.0, 0.0, 0.0, 0.0, 0.0, 0.0, 0.0, 0.0, 0.0, 0.0, 0.0, 0.0, 0.0, 0.0, 0.0, 0.0, 0.0, 0.0, 0.0, 0.0, 0.0, 0.0, 0.0, 0.0, 0.0, 0.0, 0.0, 0.0, 0.0, 0.0, 0.0, 0.0, 0.0, 0.0, 0.0, 0.0, 0.0, 0.0, 0.0, 0.0, 0.0, 0.0, 0.0, 0.0, 0.0, 0.0, 0.0, 0.0, 0.0, 0.0, 0.0, 0.0, 0.0, 0.0, 0.0, 0.0, 0.0, 0.0, 0.0, 0.0, 0.0, 0.0, 0.0, 0.0, 0.0, 0.0, 0.0, 0.0, 0.0, 0.0, 0.0, 0.0, 0.0, 0.0, 0.0, 0.0, 0.0, 0.0, 0.0, 0.0, 0.0, 0.0, 0.0, 0.0, 0.0, 0.0, 0.0, 0.0, 0.0, 0.0, 0.0, 0.0, 0.0, 0.0, 0.0, 0.0, 0.0, 0.0, 0.0, 0.0, 0.0, 0.0, 0.0, 0.0, 0.0, 0.0, 0.0, 0.0, 0.0, 0.0, 0.0, 0.0, 0.0, 0.0, 0.0, 0.0, 0.0, 0.0, 0.0, 0.0, 0.0, 0.0, 0.0, 0.0, 0.0, 0.0, 0.0, 0.0, 0.0, 0.0, 0.0, 0.0, 0.0, 0.0, 0.0, 0.0, 0.0, 0.0, 0.0, 0.0, 0.0, 0.0, 0.0, 0.0, 0.0, 0.0, 0.0, 0.0, 0.0, 0.0]}, {array[312 elements], [330.07, 330.07, 330.07, 330.07, 330.07, 330.07, 330.07, 330.07, 330.07, 330.07, 330.07, 330.07, 330.07, 330.07, 330.07, 330.07, 330.07, 330.07, 330.07, 330.07, 330.07, 330.07, 330.07, 330.07, 330.07, 330.07, 330.07, 330.07, 330.07, 330.07, 330.07, 330.07, 330.07, 330.07, 330.07, 330.07, 330.07, 330.07, 330.07, 330.07, 330.07, 330.07, 330.07, 330.07, 330.07, 330.07, 330.07, 330.07, 330.07, 330.07, 330.07, 330.07, 330.07, 330.07, 330.07, 330.07, 330.07, 330.07, 330.07, 330.07, 330.07, 330.07, 330.07, 330.07, 330.07, 330.07, 330.07, 330.07, 330.07, 330.07, 330.07, 330.07, 330.07, 330.07, 330.07, 330.07, 330.07, 330.07, 330.07, 330.07, 330.07, 330.07, 330.07, 330.07, 330.07, 330.07, 330.07, 330.07, 330.07, 330.07, 330.07, 330.07, 330.07, 330.07, 330.07, 330.07, 330.07, 330.07, 330.07, 330.07, 330.07, 330.07, 330.07, 330.07, 330.07, 330.07, 330.07, 330.07, 330.07, 330.07, 330.07, 330.07, 330.07, 330.07, 330.07, 330.07, 330.07, 330.07, 330.07, 330.07, 330.07, 330.07, 330.07, 330.07, 330.07, 330.07, 330.07, 330.07, 330.07, 330.07, 330.07, 330.07, 330.07, 330.07, 330.07, 330.07, 330.07, 330.07, 330.07, 330.07, 330.07, 330.07, 330.07, 330.07, 330.07, 330.07, 330.07, 330.07, 330.07, 330.07, 330.07, 330.07, 330.07, 330.07, 330.07, 330.07, 330.07, 330.07, 330.07, 330.07, 330.07, 330.07, 330.07, 330.07, 330.07, 330.07, 330.07, 330.07, 330.07, 330.07, 330.07, 330.07, 330.07, 330.07, 330.07, 330.07, 330.07, 330.07, 330.07, 330.07, 330.07, 330.07, 330.07, 330.07, 330.07, 330.07, 330.07, 330.07, 330.07, 330.07, 330.07, 330.07, 330.07, 330.07, 330.07, 330.07, 330.07, 330.07, 330.07, 330.07, 330.07, 330.07, 330.07, 330.07, 330.07, 330.07, 330.07, 330.07, 330.07, 330.07, 330.07, 330.07, 330.07, 330.07, 330.07, 330.07, 330.07, 330.07, 330.07, 330.07, 330.07, 330.07, 330.07, 330.07, 330.07, 330.07, 330.07, 330.07, 330.07, 330.07, 330.07, 330.07, 330.07, 330.07, 330.07, 330.07, 330.07, 330.07, 330.07, 330.07, 330.07, 330.07, 330.07, 330.07, 330.07, 330.07, 330.07, 330.07, 330.07, 330.07, 330.07, 330.07, 330.07, 330.07, 330.07, 330.07, 330.07, 330.07, 330.07, 330.07, 330.07, 330.07, 330.07, 330.07, 330.07, 330.07, 330.07, 330.07, 330.07, 330.07, 330.07, 330.07, 330.07, 330.07, 330.07, 330.07, 330.07, 330.07, 330.07, 330.07, 330.07, 330.07, 330.07, 330.07, 330.07, 330.07, 330.07, 330.07, 330.07, 330.07, 330.07, 330.07, 330.07, 330.07, 330.07, 330.07, 330.07, 330.07, 330.07, 330.07, 330.07, 330.07, 330.07, 330.07, 330.07, 330.07, 330.07, 330.07, 330.07, 330.07, 330.07, 330.07]}, {array[312 elements], [0.718, 0.718, 0.718, 0.718, 0.718, 0.718, 0.718, 0.718, 0.718, 0.718, 0.718, 0.718, 0.718, 0.718, 0.718, 0.718, 0.718, 0.718, 0.718, 0.718, 0.718, 0.718, 0.718, 0.718, 0.718, 0.718, 0.718, 0.718, 0.718, 0.718, 0.718, 0.718, 0.718, 0.718, 0.718, 0.718, 0.718, 0.718, 0.718, 0.718, 0.718, 0.718, 0.718, 0.718, 0.718, 0.718, 0.718, 0.718, 0.718, 0.718, 0.718, 0.718, 0.718, 0.718, 0.718, 0.718, 0.718, 0.718, 0.718, 0.718, 0.718, 0.718, 0.718, 0.718, 0.718, 0.718, 0.718, 0.718, 0.718, 0.718, 0.718, 0.718, 0.718, 0.718, 0.718, 0.718, 0.718, 0.718, 0.718, 0.718, 0.718, 0.718, 0.718, 0.718, 0.718, 0.718, 0.718, 0.718, 0.718, 0.718, 0.718, 0.718, 0.718, 0.718, 0.718, 0.718, 0.718, 0.718, 0.718, 0.718, 0.718, 0.718, 0.718, 0.718, 0.718, 0.718, 0.718, 0.718, 0.718, 0.718, 0.718, 0.718, 0.718, 0.718, 0.718, 0.718, 0.718, 0.718, 0.718, 0.718, 0.718, 0.718, 0.718, 0.718, 0.718, 0.718, 0.718, 0.718, 0.718, 0.718, 0.718, 0.718, 0.718, 0.718, 0.718, 0.718, 0.718, 0.718, 0.718, 0.718, 0.718, 0.718, 0.718, 0.718, 0.718, 0.718, 0.718, 0.718, 0.718, 0.718, 0.718, 0.718, 0.718, 0.718, 0.718, 0.718, 0.718, 0.718, 0.718, 0.718, 0.718, 0.718, 0.718, 0.718, 0.718, 0.718, 0.718, 0.718, 0.718, 0.718, 0.718, 0.718, 0.718, 0.718, 0.718, 0.718, 0.718, 0.718, 0.718, 0.718, 0.718, 0.718, 0.718, 0.718, 0.718, 0.718, 0.718, 0.718, 0.718, 0.718, 0.718, 0.718, 0.718, 0.718, 0.718, 0.718, 0.718, 0.718, 0.718, 0.718, 0.718, 0.718, 0.718, 0.718, 0.718, 0.718, 0.718, 0.718, 0.718, 0.718, 0.718, 0.718, 0.718, 0.718, 0.718, 0.718, 0.718, 0.718, 0.718, 0.718, 0.718, 0.718, 0.718, 0.718, 0.718, 0.718, 0.718, 0.718, 0.718, 0.718, 0.718, 0.718, 0.718, 0.718, 0.718, 0.718, 0.718, 0.718, 0.718, 0.718, 0.718, 0.718, 0.718, 0.718, 0.718, 0.718, 0.718, 0.718, 0.718, 0.718, 0.718, 0.718, 0.718, 0.718, 0.718, 0.718, 0.718, 0.718, 0.718, 0.718, 0.718, 0.718, 0.718, 0.718, 0.718, 0.718, 0.718, 0.718, 0.718, 0.718, 0.718, 0.718, 0.718, 0.718, 0.718, 0.718, 0.718, 0.718, 0.718, 0.718, 0.718, 0.718, 0.718, 0.718, 0.718, 0.718, 0.718, 0.718, 0.718, 0.718, 0.718, 0.718, 0.718, 0.718, 0.718, 0.718, 0.718, 0.718, 0.718, 0.718, 0.718, 0.718, 0.718, 0.718, 0.718, 0.718, 0.718, 0.718, 0.718, 0.718, 0.718, 0.718]}, {array[312 elements], [288.19, 288.31, 287.72, 287.34, 288.17, 287.14, 288.1, 287.28, 287.57, 288.17, 286.38, 287.7, 287.69, 286.99, 287.06, 288.23, 288.52, 287.14, 286.56, 287.02, 287.27, 287.72, 288.17, 287.23, 287.53, 287.43, 287.99, 286.91, 287.47, 286.58, 288.29, 286.41, 288.36, 287.14, 287.67, 287.94, 286.58, 288.14, 286.59, 287.47, 288.1, 286.88, 288.27, 287.3, 287.23, 287.85, 286.61, 288.17, 286.96, 286.76, 288.14, 286.44, 288.44, 286.93, 287.73, 287.82, 286.29, 288.02, 286.56, 287.76, 287.55, 286.68, 288.19, 286.58, 287.78, 287.64, 287.05, 288.14, 286.98, 288.06, 287.27, 287.57, 287.72, 286.84, 288.26, 286.22, 287.68, 286.48, 287.69, 286.31, 287.77, 286.16, 288.19, 286.91, 287.11, 287.16, 287.08, 287.06, 287.21, 286.93, 288.12, 286.26, 287.91, 286.36, 287.64, 286.9, 286.83, 288.02, 287.08, 287.25, 288.07, 286.81, 288.07, 287.3, 287.08, 288.19, 286.76, 286.88, 287.91, 286.8, 286.34, 288.38, 287.13, 286.99, 287.83, 287.28, 286.37, 287.23, 288.07, 287.15, 286.41, 287.15, 287.74, 287.47, 287.04, 286.66, 287.33, 287.44, 286.16, 288.23, 286.26, 288.27, 287.07, 287.12, 287.66, 286.19, 288.26, 286.72, 288.23, 286.1, 287.47, 286.53, 287.13, 287.23, 286.51, 287.62, 286.31, 288.08, 286.83, 287.59, 287.36, 286.91, 288.16, 286.41, 286.84, 288.07, 287.29, 286.27, 287.05, 288.22, 287.44, 286.19, 286.25, 286.09, 286.78, 286.99, 288.29, 287.73, 286.07, 286.77, 287.98, 286.86, 286.51, 288.03, 286.48, 287.39, 288.04, 286.01, 286.91, 287.82, 286.93, 285.98, 287.68, 287.95, 286.56, 286.61, 286.03, 286.19, 286.36, 286.35, 287.45, 288.01, 287.25, 286.55, 287.13, 288.08, 286.08, 288.01, 286.19, 288.23, 286.4, 288.3, 286.19, 287.46, 286.9, 286.31, 288.07, 287.28, 286.25, 287.33, 287.23, 286.77, 286.16, 286.23, 286.86, 286.91, 288.11, 287.87, 286.26, 286.48, 288.21, 287.07, 286.68, 287.65, 287.0, 286.31, 287.68, 286.73, 286.51, 287.98, 286.63, 287.21, 288.09, 287.65, 286.93, 286.78, 286.06, 286.71, 287.32, 287.91, 286.8, 287.05, 288.08, 286.7, 286.16, 288.19, 287.03, 286.96, 288.14, 286.07, 287.34, 287.55, 286.81, 287.21, 286.76, 287.0, 286.98, 286.95, 286.98, 286.29, 288.06, 287.12, 286.74, 287.92, 286.73, 286.38, 287.85, 286.03, 287.92, 287.06, 286.75, 287.53, 287.13, 286.23, 285.9, 286.93, 287.02, 288.08, 287.87, 286.38, 286.03, 287.05, 287.73, 288.12, 286.83, 285.98, 287.64, 287.74, 286.34, 287.91, 286.63, 287.37, 286.26, 287.76, 286.93, 287.14, 287.42, 287.14, 287.18, 287.76, 286.35, 287.73, 286.83, 285.98, 288.02, 287.28, 286.16, 287.06, 288.12, 286.98, 286.83, 286.24]}, {array[312 elements], [107.79, 107.64, 106.9, 107.38, 106.8, 107.18, 106.66, 107.12, 106.47, 107.08, 106.74, 106.49, 106.74, 106.58, 106.34, 106.02, 106.44, 106.59, 106.12, 106.04, 105.82, 105.77, 105.86, 105.96, 105.31, 105.97, 105.25, 105.56, 105.29, 105.35, 105.28, 105.26, 105.33, 104.91, 105.39, 104.61, 104.88, 104.83, 104.39, 104.94, 104.32, 104.6, 104.16, 104.68, 104.0, 104.64, 104.18, 104.08, 104.46, 103.62, 103.94, 103.84, 103.65, 103.86, 103.28, 103.68, 103.34, 103.44, 103.46, 102.93, 103.64, 103.2, 103.09, 103.45, 102.6, 103.29, 102.82, 103.0, 102.67, 102.91, 102.47, 102.94, 102.11, 102.56, 102.2, 102.24, 102.24, 101.97, 102.17, 102.13, 102.0, 101.88, 101.67, 102.16, 101.36, 101.97, 101.23, 101.87, 101.11, 101.74, 101.04, 101.58, 101.22, 101.03, 101.16, 100.69, 101.37, 100.88, 100.82, 101.16, 100.41, 100.83, 100.32, 100.94, 100.42, 100.44, 100.75, 99.991, 100.26, 100.59, 99.936, 99.929, 100.3, 99.895, 99.831, 100.06, 99.818, 99.487, 99.678, 99.919, 99.587, 99.354, 99.367, 99.521, 99.53, 99.154, 98.888, 99.185, 98.947, 98.908, 98.955, 98.748, 98.776, 98.98, 98.564, 98.779, 98.72, 98.57, 98.567, 98.634, 98.027, 98.703, 97.978, 98.463, 97.938, 98.135, 98.077, 97.733, 98.121, 97.518, 98.207, 97.731, 97.754, 98.004, 97.257, 97.547, 97.814, 97.466, 97.089, 97.303, 97.647, 97.522, 97.419, 97.09, 96.973, 96.688, 96.826, 97.246, 97.049, 96.423, 96.707, 97.039, 96.293, 96.527, 96.561, 96.096, 96.643, 96.527, 95.957, 96.228, 96.519, 96.033, 95.733, 96.296, 96.336, 96.001, 95.996, 95.796, 95.784, 95.429, 95.301, 95.644, 95.81, 95.587, 95.232, 95.587, 95.41, 95.345, 95.303, 95.332, 95.134, 95.237, 95.119, 94.934, 95.311, 94.637, 94.658, 95.143, 94.762, 94.564, 94.832, 94.666, 94.555, 94.242, 94.259, 94.053, 94.162, 94.54, 94.517, 93.879, 94.07, 94.352, 93.972, 93.947, 94.272, 93.645, 93.823, 94.162, 93.416, 93.675, 93.733, 93.242, 93.456, 93.827, 93.802, 93.533, 93.423, 92.959, 93.082, 93.217, 93.308, 92.844, 93.147, 93.373, 92.734, 92.833, 93.12, 92.65, 92.866, 92.896, 92.317, 92.968, 92.234, 92.739, 92.158, 92.747, 92.093, 92.648, 92.007, 92.479, 92.313, 91.859, 92.176, 92.09, 91.683, 92.239, 91.932, 91.935, 91.84, 92.034, 91.637, 91.624, 91.873, 91.588, 91.384, 91.299, 91.115, 91.212, 91.61, 91.62, 91.206, 90.951, 90.877, 91.212, 91.424, 90.928, 90.671, 90.983, 90.909, 90.63, 90.892, 90.655, 90.726, 90.978, 90.368, 90.892, 90.199, 90.734, 90.144, 90.719, 90.353, 90.287, 90.622, 90.083, 89.966, 90.476, 90.1, 89.798, 90.189, 90.211, 90.11, 89.901]}, {array[312 elements], [285.22, 283.14, 283.7, 284.22, 282.94, 284.16, 283.12, 284.19, 283.77, 283.05, 284.75, 283.73, 284.03, 284.51, 284.36, 283.49, 282.81, 284.28, 284.63, 284.72, 284.28, 283.7, 283.06, 284.27, 283.77, 283.92, 283.05, 284.28, 282.64, 284.83, 283.27, 284.87, 282.69, 283.88, 283.65, 282.81, 284.65, 283.4, 283.89, 283.8, 282.66, 284.36, 282.73, 283.65, 283.53, 283.32, 284.39, 282.72, 284.12, 284.43, 283.06, 284.86, 282.72, 284.03, 283.2, 283.29, 284.36, 282.81, 284.39, 283.24, 283.09, 284.48, 282.45, 284.24, 283.85, 282.82, 283.89, 282.42, 283.97, 282.52, 283.97, 283.12, 283.14, 283.77, 282.22, 284.6, 282.69, 284.43, 283.21, 284.56, 282.24, 284.6, 282.15, 283.65, 283.61, 283.29, 283.49, 283.27, 283.56, 283.47, 283.35, 284.22, 282.37, 284.39, 282.72, 283.53, 283.53, 282.37, 283.7, 283.17, 282.39, 283.49, 282.34, 283.2, 283.27, 282.19, 283.52, 283.64, 282.1, 283.68, 283.97, 281.94, 282.93, 283.59, 282.72, 283.2, 283.92, 283.4, 282.13, 283.12, 283.92, 283.17, 282.46, 282.72, 283.09, 283.64, 282.88, 282.64, 284.28, 282.03, 284.04, 281.85, 284.15, 283.12, 282.66, 284.34, 281.94, 284.07, 281.85, 284.48, 282.82, 283.06, 283.05, 283.12, 283.97, 282.49, 284.04, 282.1, 283.37, 282.76, 282.49, 283.68, 281.86, 283.92, 283.4, 282.27, 283.09, 284.03, 283.2, 281.77, 282.69, 283.8, 283.88, 284.19, 283.24, 283.17, 281.38, 282.34, 283.73, 283.32, 281.82, 283.17, 283.7, 281.71, 283.41, 282.39, 281.64, 284.07, 283.06, 281.89, 282.54, 283.68, 282.18, 281.79, 283.47, 283.44, 284.22, 283.95, 283.85, 283.64, 282.61, 281.82, 282.72, 283.29, 282.85, 281.71, 283.95, 281.97, 283.89, 281.43, 283.89, 281.56, 284.1, 282.42, 282.76, 283.68, 281.67, 282.27, 283.49, 282.39, 282.37, 283.09, 283.73, 283.52, 282.82, 282.97, 281.38, 281.35, 283.49, 283.17, 281.16, 282.39, 283.06, 281.82, 282.57, 283.7, 281.89, 282.81, 283.2, 281.32, 282.97, 282.34, 281.2, 281.82, 282.76, 282.73, 283.64, 282.81, 282.27, 281.55, 282.49, 282.54, 281.11, 283.14, 283.8, 281.4, 282.61, 283.06, 281.4, 283.89, 282.39, 281.79, 282.78, 282.31, 283.41, 282.85, 282.57, 282.69, 282.52, 283.27, 281.28, 282.39, 282.78, 281.23, 282.88, 283.21, 281.59, 283.92, 281.49, 282.3, 282.85, 281.94, 282.64, 283.27, 283.61, 282.72, 282.52, 281.62, 281.49, 282.93, 283.41, 283.27, 281.77, 281.16, 282.69, 283.65, 281.91, 281.85, 283.32, 281.7, 282.78, 282.18, 283.49, 281.32, 282.45, 282.07, 282.07, 282.64, 282.52, 281.47, 283.41, 281.77, 282.42, 283.52, 281.38, 282.19, 283.64, 282.49, 281.35, 282.31, 282.69, 283.56]}, {array[312 elements], [274.45, 272.46, 276.98, 273.71, 276.19, 274.02, 276.37, 273.51, 276.45, 272.35, 274.14, 275.3, 273.26, 273.93, 276.9, 276.75, 273.51, 272.19, 274.23, 274.96, 275.72, 275.3, 274.33, 273.48, 276.87, 272.78, 275.9, 274.0, 274.93, 274.3, 274.48, 274.04, 272.81, 275.42, 272.24, 275.78, 274.45, 272.05, 276.33, 272.94, 275.49, 273.97, 275.8, 272.49, 276.4, 271.91, 274.26, 274.02, 271.8, 276.64, 273.9, 274.35, 274.99, 273.52, 276.36, 273.34, 275.38, 274.0, 273.67, 276.22, 271.9, 274.14, 273.89, 271.76, 276.52, 271.76, 274.56, 272.05, 274.51, 272.12, 275.06, 271.65, 276.26, 273.27, 274.62, 274.3, 273.38, 275.72, 273.65, 273.59, 273.45, 274.26, 274.51, 271.64, 276.36, 271.8, 275.96, 271.54, 275.94, 271.52, 275.51, 273.62, 273.67, 274.85, 273.3, 276.17, 271.59, 274.18, 274.41, 271.8, 275.82, 273.41, 275.39, 271.97, 274.79, 273.67, 271.45, 276.07, 273.86, 271.57, 275.03, 274.55, 272.38, 274.28, 274.02, 272.33, 273.69, 275.45, 273.82, 271.52, 273.2, 274.82, 274.14, 272.68, 272.05, 273.67, 274.92, 272.68, 274.3, 273.97, 273.59, 274.16, 274.35, 271.9, 274.44, 273.03, 272.56, 273.62, 272.96, 272.33, 275.33, 271.27, 275.23, 271.76, 275.0, 273.03, 273.31, 274.55, 272.35, 275.72, 270.91, 273.67, 272.85, 271.31, 275.65, 273.58, 271.43, 272.85, 275.42, 273.52, 270.73, 271.15, 271.65, 273.23, 273.59, 275.51, 273.93, 270.65, 271.61, 275.33, 273.19, 270.58, 275.12, 273.05, 272.24, 275.15, 271.64, 272.01, 273.93, 273.19, 270.66, 273.26, 275.23, 271.36, 270.8, 272.49, 272.22, 273.26, 273.05, 275.06, 275.39, 272.81, 271.54, 272.53, 274.62, 272.05, 272.45, 273.15, 272.61, 272.57, 272.92, 272.57, 272.39, 273.74, 270.66, 274.52, 274.35, 270.44, 272.75, 273.65, 271.83, 272.01, 272.53, 274.56, 273.86, 274.93, 274.07, 271.06, 270.88, 274.78, 273.59, 271.15, 273.41, 273.05, 270.66, 272.75, 273.27, 270.26, 275.0, 272.94, 271.69, 274.92, 273.26, 270.48, 270.19, 271.91, 272.22, 275.1, 273.85, 272.92, 271.64, 274.3, 272.31, 270.24, 274.07, 273.48, 271.17, 273.93, 272.22, 271.64, 274.96, 270.52, 275.19, 271.68, 274.82, 270.71, 274.96, 270.58, 274.92, 270.8, 272.33, 274.18, 271.86, 272.71, 274.96, 270.55, 272.96, 272.05, 272.57, 270.98, 272.99, 273.01, 270.98, 272.57, 273.59, 273.97, 274.85, 274.11, 270.71, 270.41, 272.75, 274.45, 274.4, 272.12, 270.14, 273.1, 274.71, 272.71, 272.35, 274.37, 271.68, 273.74, 272.18, 270.55, 274.16, 270.39, 274.93, 270.59, 274.51, 270.84, 272.71, 272.99, 270.32, 273.45, 274.16, 270.02, 272.38, 274.23, 273.15, 270.66, 271.09, 272.5]}, {array[312 elements], []}]
  out "LSI-U Grpah 2":cluster{dbl[], dbl[]}[](graph)=[{array[312 elements], [286.85, 286.84, 286.82, 286.84, 286.77, 286.76, 286.74, 286.79, 286.78, 286.78, 286.83, 286.73, 286.76, 286.74, 286.76, 286.75, 286.72, 286.77, 286.72, 286.69, 286.75, 286.7, 286.68, 286.7, 286.64, 286.69, 286.65, 286.68, 286.7, 286.67, 286.64, 286.62, 286.64, 286.63, 286.64, 286.62, 286.6, 286.61, 286.63, 286.61, 286.59, 286.61, 286.59, 286.59, 286.59, 286.59, 286.54, 286.56, 286.54, 286.52, 286.56, 286.54, 286.54, 286.51, 286.51, 286.49, 286.53, 286.47, 286.51, 286.51, 286.5, 286.48, 286.47, 286.44, 286.47, 286.46, 286.46, 286.43, 286.41, 286.39, 286.43, 286.41, 286.4, 286.38, 286.4, 286.39, 286.36, 286.42, 286.38, 286.32, 286.36, 286.32, 286.37, 286.36, 286.3, 286.34, 286.33, 286.33, 286.31, 286.25, 286.27, 286.24, 286.28, 286.3, 286.31, 286.26, 286.26, 286.22, 286.23, 286.25, 286.23, 286.26, 286.2, 286.21, 286.22, 286.22, 286.2, 286.19, 286.19, 286.15, 286.18, 286.19, 286.17, 286.16, 286.17, 286.18, 286.15, 286.13, 286.17, 286.1, 286.08, 286.1, 286.14, 286.08, 286.11, 286.07, 286.08, 286.06, 286.08, 286.09, 286.04, 286.02, 286.03, 286.05, 286.01, 286.04, 286.04, 286.01, 286.01, 286.0, 285.98, 286.03, 286.0, 285.97, 285.98, 285.97, 286.0, 285.99, 285.91, 285.91, 285.89, 285.96, 285.95, 285.94, 285.93, 285.9, 285.89, 285.88, 285.89, 285.91, 285.88, 285.87, 285.85, 285.84, 285.84, 285.86, 285.84, 285.82, 285.81, 285.81, 285.79, 285.81, 285.81, 285.8, 285.77, 285.76, 285.81, 285.77, 285.79, 285.73, 285.76, 285.72, 285.71, 285.75, 285.71, 285.71, 285.73, 285.69, 285.74, 285.71, 285.7, 285.7, 285.64, 285.66, 285.63, 285.67, 285.69, 285.64, 285.63, 285.62, 285.63, 285.63, 285.61, 285.56, 285.55, 285.57, 285.57, 285.56, 285.55, 285.58, 285.54, 285.56, 285.52, 285.54, 285.55, 285.5, 285.54, 285.49, 285.51, 285.46, 285.45, 285.5, 285.52, 285.46, 285.47, 285.49, 285.47, 285.47, 285.42, 285.44, 285.42, 285.4, 285.41, 285.46, 285.4, 285.37, 285.39, 285.36, 285.37, 285.37, 285.37, 285.36, 285.39, 285.31, 285.32, 285.35, 285.29, 285.3, 285.29, 285.33, 285.3, 285.31, 285.28, 285.26, 285.29, 285.26, 285.22, 285.23, 285.23, 285.22, 285.28, 285.23, 285.2, 285.19, 285.2, 285.2, 285.16, 285.22, 285.18, 285.18, 285.17, 285.14, 285.13, 285.12, 285.13, 285.11, 285.16, 285.16, 285.1, 285.11, 285.09, 285.08, 285.09, 285.07, 285.08, 285.08, 285.05, 285.05, 285.02, 285.05, 285.05, 284.99, 285.04, 285.01, 285.01, 284.97, 284.99, 285.0, 284.95, 284.98, 284.95, 284.99, 284.94, 284.93, 284.92, 284.92, 284.91, 284.93, 284.88, 284.91, 284.9, 284.87]}, {array[312 elements], [0.0, 0.0, 0.0, 0.0, 0.0, 0.0, 0.0, 0.0, 0.0, 0.0, 0.0, 0.0, 0.0, 0.0, 0.0, 0.0, 0.0, 0.0, 0.0, 0.0, 0.0, 0.0, 0.0, 0.0, 0.0, 0.0, 0.0, 0.0, 0.0, 0.0, 0.0, 0.0, 0.0, 0.0, 0.0, 0.0, 0.0, 0.0, 0.0, 0.0, 0.0, 0.0, 0.0, 0.0, 0.0, 0.0, 0.0, 0.0, 0.0, 0.0, 0.0, 0.0, 0.0, 0.0, 0.0, 0.0, 0.0, 0.0, 0.0, 0.0, 0.0, 0.0, 0.0, 0.0, 0.0, 0.0, 0.0, 0.0, 0.0, 0.0, 0.0, 0.0, 0.0, 0.0, 0.0, 0.0, 0.0, 0.0, 0.0, 0.0, 0.0, 0.0, 0.0, 0.0, 0.0, 0.0, 0.0, 0.0, 0.0, 0.0, 0.0, 0.0, 0.0, 0.0, 0.0, 0.0, 0.0, 0.0, 0.0, 0.0, 0.0, 0.0, 0.0, 0.0, 0.0, 0.0, 0.0, 0.0, 0.0, 0.0, 0.0, 0.0, 0.0, 0.0, 0.0, 0.0, 0.0, 0.0, 0.0, 0.0, 0.0, 0.0, 0.0, 0.0, 0.0, 0.0, 0.0, 0.0, 0.0, 0.0, 0.0, 0.0, 0.0, 0.0, 0.0, 0.0, 0.0, 0.0, 0.0, 0.0, 0.0, 0.0, 0.0, 0.0, 0.0, 0.0, 0.0, 0.0, 0.0, 0.0, 0.0, 0.0, 0.0, 0.0, 0.0, 0.0, 0.0, 0.0, 0.0, 0.0, 0.0, 0.0, 0.0, 0.0, 0.0, 0.0, 0.0, 0.0, 0.0, 0.0, 0.0, 0.0, 0.0, 0.0, 0.0, 0.0, 0.0, 0.0, 0.0, 0.0, 0.0, 0.0, 0.0, 0.0, 0.0, 0.0, 0.0, 0.0, 0.0, 0.0, 0.0, 0.0, 0.0, 0.0, 0.0, 0.0, 0.0, 0.0, 0.0, 0.0, 0.0, 0.0, 0.0, 0.0, 0.0, 0.0, 0.0, 0.0, 0.0, 0.0, 0.0, 0.0, 0.0, 0.0, 0.0, 0.0, 0.0, 0.0, 0.0, 0.0, 0.0, 0.0, 0.0, 0.0, 0.0, 0.0, 0.0, 0.0, 0.0, 0.0, 0.0, 0.0, 0.0, 0.0, 0.0, 0.0, 0.0, 0.0, 0.0, 0.0, 0.0, 0.0, 0.0, 0.0, 0.0, 0.0, 0.0, 0.0, 0.0, 0.0, 0.0, 0.0, 0.0, 0.0, 0.0, 0.0, 0.0, 0.0, 0.0, 0.0, 0.0, 0.0, 0.0, 0.0, 0.0, 0.0, 0.0, 0.0, 0.0, 0.0, 0.0, 0.0, 0.0, 0.0, 0.0, 0.0, 0.0, 0.0, 0.0, 0.0, 0.0, 0.0, 0.0, 0.0, 0.0, 0.0, 0.0, 0.0, 0.0, 0.0, 0.0, 0.0, 0.0, 0.0, 0.0, 0.0, 0.0, 0.0, 0.0, 0.0, 0.0, 0.0, 0.0, 0.0, 0.0, 0.0, 0.0, 0.0, 0.0, 0.0, 0.0, 0.0]}, {array[312 elements], [330.07, 330.07, 330.07, 330.07, 330.07, 330.07, 330.07, 330.07, 330.07, 330.07, 330.07, 330.07, 330.07, 330.07, 330.07, 330.07, 330.07, 330.07, 330.07, 330.07, 330.07, 330.07, 330.07, 330.07, 330.07, 330.07, 330.07, 330.07, 330.07, 330.07, 330.07, 330.07, 330.07, 330.07, 330.07, 330.07, 330.07, 330.07, 330.07, 330.07, 330.07, 330.07, 330.07, 330.07, 330.07, 330.07, 330.07, 330.07, 330.07, 330.07, 330.07, 330.07, 330.07, 330.07, 330.07, 330.07, 330.07, 330.07, 330.07, 330.07, 330.07, 330.07, 330.07, 330.07, 330.07, 330.07, 330.07, 330.07, 330.07, 330.07, 330.07, 330.07, 330.07, 330.07, 330.07, 330.07, 330.07, 330.07, 330.07, 330.07, 330.07, 330.07, 330.07, 330.07, 330.07, 330.07, 330.07, 330.07, 330.07, 330.07, 330.07, 330.07, 330.07, 330.07, 330.07, 330.07, 330.07, 330.07, 330.07, 330.07, 330.07, 330.07, 330.07, 330.07, 330.07, 330.07, 330.07, 330.07, 330.07, 330.07, 330.07, 330.07, 330.07, 330.07, 330.07, 330.07, 330.07, 330.07, 330.07, 330.07, 330.07, 330.07, 330.07, 330.07, 330.07, 330.07, 330.07, 330.07, 330.07, 330.07, 330.07, 330.07, 330.07, 330.07, 330.07, 330.07, 330.07, 330.07, 330.07, 330.07, 330.07, 330.07, 330.07, 330.07, 330.07, 330.07, 330.07, 330.07, 330.07, 330.07, 330.07, 330.07, 330.07, 330.07, 330.07, 330.07, 330.07, 330.07, 330.07, 330.07, 330.07, 330.07, 330.07, 330.07, 330.07, 330.07, 330.07, 330.07, 330.07, 330.07, 330.07, 330.07, 330.07, 330.07, 330.07, 330.07, 330.07, 330.07, 330.07, 330.07, 330.07, 330.07, 330.07, 330.07, 330.07, 330.07, 330.07, 330.07, 330.07, 330.07, 330.07, 330.07, 330.07, 330.07, 330.07, 330.07, 330.07, 330.07, 330.07, 330.07, 330.07, 330.07, 330.07, 330.07, 330.07, 330.07, 330.07, 330.07, 330.07, 330.07, 330.07, 330.07, 330.07, 330.07, 330.07, 330.07, 330.07, 330.07, 330.07, 330.07, 330.07, 330.07, 330.07, 330.07, 330.07, 330.07, 330.07, 330.07, 330.07, 330.07, 330.07, 330.07, 330.07, 330.07, 330.07, 330.07, 330.07, 330.07, 330.07, 330.07, 330.07, 330.07, 330.07, 330.07, 330.07, 330.07, 330.07, 330.07, 330.07, 330.07, 330.07, 330.07, 330.07, 330.07, 330.07, 330.07, 330.07, 330.07, 330.07, 330.07, 330.07, 330.07, 330.07, 330.07, 330.07, 330.07, 330.07, 330.07, 330.07, 330.07, 330.07, 330.07, 330.07, 330.07, 330.07, 330.07, 330.07, 330.07, 330.07, 330.07, 330.07, 330.07, 330.07, 330.07, 330.07, 330.07, 330.07, 330.07, 330.07, 330.07, 330.07, 330.07, 330.07, 330.07, 330.07, 330.07, 330.07, 330.07, 330.07, 330.07, 330.07, 330.07, 330.07, 330.07, 330.07, 330.07, 330.07, 330.07, 330.07, 330.07, 330.07, 330.07]}, {array[312 elements], [0.718, 0.718, 0.718, 0.718, 0.718, 0.718, 0.718, 0.718, 0.718, 0.718, 0.718, 0.718, 0.718, 0.718, 0.718, 0.718, 0.718, 0.718, 0.718, 0.718, 0.718, 0.718, 0.718, 0.718, 0.718, 0.718, 0.718, 0.718, 0.718, 0.718, 0.718, 0.718, 0.718, 0.718, 0.718, 0.718, 0.718, 0.718, 0.718, 0.718, 0.718, 0.718, 0.718, 0.718, 0.718, 0.718, 0.718, 0.718, 0.718, 0.718, 0.718, 0.718, 0.718, 0.718, 0.718, 0.718, 0.718, 0.718, 0.718, 0.718, 0.718, 0.718, 0.718, 0.718, 0.718, 0.718, 0.718, 0.718, 0.718, 0.718, 0.718, 0.718, 0.718, 0.718, 0.718, 0.718, 0.718, 0.718, 0.718, 0.718, 0.718, 0.718, 0.718, 0.718, 0.718, 0.718, 0.718, 0.718, 0.718, 0.718, 0.718, 0.718, 0.718, 0.718, 0.718, 0.718, 0.718, 0.718, 0.718, 0.718, 0.718, 0.718, 0.718, 0.718, 0.718, 0.718, 0.718, 0.718, 0.718, 0.718, 0.718, 0.718, 0.718, 0.718, 0.718, 0.718, 0.718, 0.718, 0.718, 0.718, 0.718, 0.718, 0.718, 0.718, 0.718, 0.718, 0.718, 0.718, 0.718, 0.718, 0.718, 0.718, 0.718, 0.718, 0.718, 0.718, 0.718, 0.718, 0.718, 0.718, 0.718, 0.718, 0.718, 0.718, 0.718, 0.718, 0.718, 0.718, 0.718, 0.718, 0.718, 0.718, 0.718, 0.718, 0.718, 0.718, 0.718, 0.718, 0.718, 0.718, 0.718, 0.718, 0.718, 0.718, 0.718, 0.718, 0.718, 0.718, 0.718, 0.718, 0.718, 0.718, 0.718, 0.718, 0.718, 0.718, 0.718, 0.718, 0.718, 0.718, 0.718, 0.718, 0.718, 0.718, 0.718, 0.718, 0.718, 0.718, 0.718, 0.718, 0.718, 0.718, 0.718, 0.718, 0.718, 0.718, 0.718, 0.718, 0.718, 0.718, 0.718, 0.718, 0.718, 0.718, 0.718, 0.718, 0.718, 0.718, 0.718, 0.718, 0.718, 0.718, 0.718, 0.718, 0.718, 0.718, 0.718, 0.718, 0.718, 0.718, 0.718, 0.718, 0.718, 0.718, 0.718, 0.718, 0.718, 0.718, 0.718, 0.718, 0.718, 0.718, 0.718, 0.718, 0.718, 0.718, 0.718, 0.718, 0.718, 0.718, 0.718, 0.718, 0.718, 0.718, 0.718, 0.718, 0.718, 0.718, 0.718, 0.718, 0.718, 0.718, 0.718, 0.718, 0.718, 0.718, 0.718, 0.718, 0.718, 0.718, 0.718, 0.718, 0.718, 0.718, 0.718, 0.718, 0.718, 0.718, 0.718, 0.718, 0.718, 0.718, 0.718, 0.718, 0.718, 0.718, 0.718, 0.718, 0.718, 0.718, 0.718, 0.718, 0.718, 0.718, 0.718, 0.718, 0.718, 0.718, 0.718, 0.718, 0.718, 0.718, 0.718, 0.718, 0.718, 0.718, 0.718, 0.718, 0.718, 0.718, 0.718, 0.718, 0.718, 0.718, 0.718, 0.718, 0.718, 0.718, 0.718, 0.718, 0.718, 0.718]}, {array[312 elements], [288.19, 288.31, 287.72, 287.34, 288.17, 287.14, 288.1, 287.28, 287.57, 288.17, 286.38, 287.7, 287.69, 286.99, 287.06, 288.23, 288.52, 287.14, 286.56, 287.02, 287.27, 287.72, 288.17, 287.23, 287.53, 287.43, 287.99, 286.91, 287.47, 286.58, 288.29, 286.41, 288.36, 287.14, 287.67, 287.94, 286.58, 288.14, 286.59, 287.47, 288.1, 286.88, 288.27, 287.3, 287.23, 287.85, 286.61, 288.17, 286.96, 286.76, 288.14, 286.44, 288.44, 286.93, 287.73, 287.82, 286.29, 288.02, 286.56, 287.76, 287.55, 286.68, 288.19, 286.58, 287.78, 287.64, 287.05, 288.14, 286.98, 288.06, 287.27, 287.57, 287.72, 286.84, 288.26, 286.22, 287.68, 286.48, 287.69, 286.31, 287.77, 286.16, 288.19, 286.91, 287.11, 287.16, 287.08, 287.06, 287.21, 286.93, 288.12, 286.26, 287.91, 286.36, 287.64, 286.9, 286.83, 288.02, 287.08, 287.25, 288.07, 286.81, 288.07, 287.3, 287.08, 288.19, 286.76, 286.88, 287.91, 286.8, 286.34, 288.38, 287.13, 286.99, 287.83, 287.28, 286.37, 287.23, 288.07, 287.15, 286.41, 287.15, 287.74, 287.47, 287.04, 286.66, 287.33, 287.44, 286.16, 288.23, 286.26, 288.27, 287.07, 287.12, 287.66, 286.19, 288.26, 286.72, 288.23, 286.1, 287.47, 286.53, 287.13, 287.23, 286.51, 287.62, 286.31, 288.08, 286.83, 287.59, 287.36, 286.91, 288.16, 286.41, 286.84, 288.07, 287.29, 286.27, 287.05, 288.22, 287.44, 286.19, 286.25, 286.09, 286.78, 286.99, 288.29, 287.73, 286.07, 286.77, 287.98, 286.86, 286.51, 288.03, 286.48, 287.39, 288.04, 286.01, 286.91, 287.82, 286.93, 285.98, 287.68, 287.95, 286.56, 286.61, 286.03, 286.19, 286.36, 286.35, 287.45, 288.01, 287.25, 286.55, 287.13, 288.08, 286.08, 288.01, 286.19, 288.23, 286.4, 288.3, 286.19, 287.46, 286.9, 286.31, 288.07, 287.28, 286.25, 287.33, 287.23, 286.77, 286.16, 286.23, 286.86, 286.91, 288.11, 287.87, 286.26, 286.48, 288.21, 287.07, 286.68, 287.65, 287.0, 286.31, 287.68, 286.73, 286.51, 287.98, 286.63, 287.21, 288.09, 287.65, 286.93, 286.78, 286.06, 286.71, 287.32, 287.91, 286.8, 287.05, 288.08, 286.7, 286.16, 288.19, 287.03, 286.96, 288.14, 286.07, 287.34, 287.55, 286.81, 287.21, 286.76, 287.0, 286.98, 286.95, 286.98, 286.29, 288.06, 287.12, 286.74, 287.92, 286.73, 286.38, 287.85, 286.03, 287.92, 287.06, 286.75, 287.53, 287.13, 286.23, 285.9, 286.93, 287.02, 288.08, 287.87, 286.38, 286.03, 287.05, 287.73, 288.12, 286.83, 285.98, 287.64, 287.74, 286.34, 287.91, 286.63, 287.37, 286.26, 287.76, 286.93, 287.14, 287.42, 287.14, 287.18, 287.76, 286.35, 287.73, 286.83, 285.98, 288.02, 287.28, 286.16, 287.06, 288.12, 286.98, 286.83, 286.24]}, {array[312 elements], [107.79, 107.64, 106.9, 107.38, 106.8, 107.18, 106.66, 107.12, 106.47, 107.08, 106.74, 106.49, 106.74, 106.58, 106.34, 106.02, 106.44, 106.59, 106.12, 106.04, 105.82, 105.77, 105.86, 105.96, 105.31, 105.97, 105.25, 105.56, 105.29, 105.35, 105.28, 105.26, 105.33, 104.91, 105.39, 104.61, 104.88, 104.83, 104.39, 104.94, 104.32, 104.6, 104.16, 104.68, 104.0, 104.64, 104.18, 104.08, 104.46, 103.62, 103.94, 103.84, 103.65, 103.86, 103.28, 103.68, 103.34, 103.44, 103.46, 102.93, 103.64, 103.2, 103.09, 103.45, 102.6, 103.29, 102.82, 103.0, 102.67, 102.91, 102.47, 102.94, 102.11, 102.56, 102.2, 102.24, 102.24, 101.97, 102.17, 102.13, 102.0, 101.88, 101.67, 102.16, 101.36, 101.97, 101.23, 101.87, 101.11, 101.74, 101.04, 101.58, 101.22, 101.03, 101.16, 100.69, 101.37, 100.88, 100.82, 101.16, 100.41, 100.83, 100.32, 100.94, 100.42, 100.44, 100.75, 99.991, 100.26, 100.59, 99.936, 99.929, 100.3, 99.895, 99.831, 100.06, 99.818, 99.487, 99.678, 99.919, 99.587, 99.354, 99.367, 99.521, 99.53, 99.154, 98.888, 99.185, 98.947, 98.908, 98.955, 98.748, 98.776, 98.98, 98.564, 98.779, 98.72, 98.57, 98.567, 98.634, 98.027, 98.703, 97.978, 98.463, 97.938, 98.135, 98.077, 97.733, 98.121, 97.518, 98.207, 97.731, 97.754, 98.004, 97.257, 97.547, 97.814, 97.466, 97.089, 97.303, 97.647, 97.522, 97.419, 97.09, 96.973, 96.688, 96.826, 97.246, 97.049, 96.423, 96.707, 97.039, 96.293, 96.527, 96.561, 96.096, 96.643, 96.527, 95.957, 96.228, 96.519, 96.033, 95.733, 96.296, 96.336, 96.001, 95.996, 95.796, 95.784, 95.429, 95.301, 95.644, 95.81, 95.587, 95.232, 95.587, 95.41, 95.345, 95.303, 95.332, 95.134, 95.237, 95.119, 94.934, 95.311, 94.637, 94.658, 95.143, 94.762, 94.564, 94.832, 94.666, 94.555, 94.242, 94.259, 94.053, 94.162, 94.54, 94.517, 93.879, 94.07, 94.352, 93.972, 93.947, 94.272, 93.645, 93.823, 94.162, 93.416, 93.675, 93.733, 93.242, 93.456, 93.827, 93.802, 93.533, 93.423, 92.959, 93.082, 93.217, 93.308, 92.844, 93.147, 93.373, 92.734, 92.833, 93.12, 92.65, 92.866, 92.896, 92.317, 92.968, 92.234, 92.739, 92.158, 92.747, 92.093, 92.648, 92.007, 92.479, 92.313, 91.859, 92.176, 92.09, 91.683, 92.239, 91.932, 91.935, 91.84, 92.034, 91.637, 91.624, 91.873, 91.588, 91.384, 91.299, 91.115, 91.212, 91.61, 91.62, 91.206, 90.951, 90.877, 91.212, 91.424, 90.928, 90.671, 90.983, 90.909, 90.63, 90.892, 90.655, 90.726, 90.978, 90.368, 90.892, 90.199, 90.734, 90.144, 90.719, 90.353, 90.287, 90.622, 90.083, 89.966, 90.476, 90.1, 89.798, 90.189, 90.211, 90.11, 89.901]}, {array[312 elements], [285.22, 283.14, 283.7, 284.22, 282.94, 284.16, 283.12, 284.19, 283.77, 283.05, 284.75, 283.73, 284.03, 284.51, 284.36, 283.49, 282.81, 284.28, 284.63, 284.72, 284.28, 283.7, 283.06, 284.27, 283.77, 283.92, 283.05, 284.28, 282.64, 284.83, 283.27, 284.87, 282.69, 283.88, 283.65, 282.81, 284.65, 283.4, 283.89, 283.8, 282.66, 284.36, 282.73, 283.65, 283.53, 283.32, 284.39, 282.72, 284.12, 284.43, 283.06, 284.86, 282.72, 284.03, 283.2, 283.29, 284.36, 282.81, 284.39, 283.24, 283.09, 284.48, 282.45, 284.24, 283.85, 282.82, 283.89, 282.42, 283.97, 282.52, 283.97, 283.12, 283.14, 283.77, 282.22, 284.6, 282.69, 284.43, 283.21, 284.56, 282.24, 284.6, 282.15, 283.65, 283.61, 283.29, 283.49, 283.27, 283.56, 283.47, 283.35, 284.22, 282.37, 284.39, 282.72, 283.53, 283.53, 282.37, 283.7, 283.17, 282.39, 283.49, 282.34, 283.2, 283.27, 282.19, 283.52, 283.64, 282.1, 283.68, 283.97, 281.94, 282.93, 283.59, 282.72, 283.2, 283.92, 283.4, 282.13, 283.12, 283.92, 283.17, 282.46, 282.72, 283.09, 283.64, 282.88, 282.64, 284.28, 282.03, 284.04, 281.85, 284.15, 283.12, 282.66, 284.34, 281.94, 284.07, 281.85, 284.48, 282.82, 283.06, 283.05, 283.12, 283.97, 282.49, 284.04, 282.1, 283.37, 282.76, 282.49, 283.68, 281.86, 283.92, 283.4, 282.27, 283.09, 284.03, 283.2, 281.77, 282.69, 283.8, 283.88, 284.19, 283.24, 283.17, 281.38, 282.34, 283.73, 283.32, 281.82, 283.17, 283.7, 281.71, 283.41, 282.39, 281.64, 284.07, 283.06, 281.89, 282.54, 283.68, 282.18, 281.79, 283.47, 283.44, 284.22, 283.95, 283.85, 283.64, 282.61, 281.82, 282.72, 283.29, 282.85, 281.71, 283.95, 281.97, 283.89, 281.43, 283.89, 281.56, 284.1, 282.42, 282.76, 283.68, 281.67, 282.27, 283.49, 282.39, 282.37, 283.09, 283.73, 283.52, 282.82, 282.97, 281.38, 281.35, 283.49, 283.17, 281.16, 282.39, 283.06, 281.82, 282.57, 283.7, 281.89, 282.81, 283.2, 281.32, 282.97, 282.34, 281.2, 281.82, 282.76, 282.73, 283.64, 282.81, 282.27, 281.55, 282.49, 282.54, 281.11, 283.14, 283.8, 281.4, 282.61, 283.06, 281.4, 283.89, 282.39, 281.79, 282.78, 282.31, 283.41, 282.85, 282.57, 282.69, 282.52, 283.27, 281.28, 282.39, 282.78, 281.23, 282.88, 283.21, 281.59, 283.92, 281.49, 282.3, 282.85, 281.94, 282.64, 283.27, 283.61, 282.72, 282.52, 281.62, 281.49, 282.93, 283.41, 283.27, 281.77, 281.16, 282.69, 283.65, 281.91, 281.85, 283.32, 281.7, 282.78, 282.18, 283.49, 281.32, 282.45, 282.07, 282.07, 282.64, 282.52, 281.47, 283.41, 281.77, 282.42, 283.52, 281.38, 282.19, 283.64, 282.49, 281.35, 282.31, 282.69, 283.56]}, {array[312 elements], [274.45, 272.46, 276.98, 273.71, 276.19, 274.02, 276.37, 273.51, 276.45, 272.35, 274.14, 275.3, 273.26, 273.93, 276.9, 276.75, 273.51, 272.19, 274.23, 274.96, 275.72, 275.3, 274.33, 273.48, 276.87, 272.78, 275.9, 274.0, 274.93, 274.3, 274.48, 274.04, 272.81, 275.42, 272.24, 275.78, 274.45, 272.05, 276.33, 272.94, 275.49, 273.97, 275.8, 272.49, 276.4, 271.91, 274.26, 274.02, 271.8, 276.64, 273.9, 274.35, 274.99, 273.52, 276.36, 273.34, 275.38, 274.0, 273.67, 276.22, 271.9, 274.14, 273.89, 271.76, 276.52, 271.76, 274.56, 272.05, 274.51, 272.12, 275.06, 271.65, 276.26, 273.27, 274.62, 274.3, 273.38, 275.72, 273.65, 273.59, 273.45, 274.26, 274.51, 271.64, 276.36, 271.8, 275.96, 271.54, 275.94, 271.52, 275.51, 273.62, 273.67, 274.85, 273.3, 276.17, 271.59, 274.18, 274.41, 271.8, 275.82, 273.41, 275.39, 271.97, 274.79, 273.67, 271.45, 276.07, 273.86, 271.57, 275.03, 274.55, 272.38, 274.28, 274.02, 272.33, 273.69, 275.45, 273.82, 271.52, 273.2, 274.82, 274.14, 272.68, 272.05, 273.67, 274.92, 272.68, 274.3, 273.97, 273.59, 274.16, 274.35, 271.9, 274.44, 273.03, 272.56, 273.62, 272.96, 272.33, 275.33, 271.27, 275.23, 271.76, 275.0, 273.03, 273.31, 274.55, 272.35, 275.72, 270.91, 273.67, 272.85, 271.31, 275.65, 273.58, 271.43, 272.85, 275.42, 273.52, 270.73, 271.15, 271.65, 273.23, 273.59, 275.51, 273.93, 270.65, 271.61, 275.33, 273.19, 270.58, 275.12, 273.05, 272.24, 275.15, 271.64, 272.01, 273.93, 273.19, 270.66, 273.26, 275.23, 271.36, 270.8, 272.49, 272.22, 273.26, 273.05, 275.06, 275.39, 272.81, 271.54, 272.53, 274.62, 272.05, 272.45, 273.15, 272.61, 272.57, 272.92, 272.57, 272.39, 273.74, 270.66, 274.52, 274.35, 270.44, 272.75, 273.65, 271.83, 272.01, 272.53, 274.56, 273.86, 274.93, 274.07, 271.06, 270.88, 274.78, 273.59, 271.15, 273.41, 273.05, 270.66, 272.75, 273.27, 270.26, 275.0, 272.94, 271.69, 274.92, 273.26, 270.48, 270.19, 271.91, 272.22, 275.1, 273.85, 272.92, 271.64, 274.3, 272.31, 270.24, 274.07, 273.48, 271.17, 273.93, 272.22, 271.64, 274.96, 270.52, 275.19, 271.68, 274.82, 270.71, 274.96, 270.58, 274.92, 270.8, 272.33, 274.18, 271.86, 272.71, 274.96, 270.55, 272.96, 272.05, 272.57, 270.98, 272.99, 273.01, 270.98, 272.57, 273.59, 273.97, 274.85, 274.11, 270.71, 270.41, 272.75, 274.45, 274.4, 272.12, 270.14, 273.1, 274.71, 272.71, 272.35, 274.37, 271.68, 273.74, 272.18, 270.55, 274.16, 270.39, 274.93, 270.59, 274.51, 270.84, 272.71, 272.99, 270.32, 273.45, 274.16, 270.02, 272.38, 274.23, 273.15, 270.66, 271.09, 272.5]}, {array[312 elements], []}]
  out "LSI-D Grpah 3":cluster{dbl[], dbl[]}[](graph)=[{array[312 elements], [0.0, 296.61, 296.59, 296.63, 296.62, 296.61, 296.61, 296.61, 296.61, 296.61, 296.57, 296.65, 296.6, 296.66, 296.59, 296.6, 296.58, 296.64, 296.63, 296.66, 296.57, 296.61, 296.6, 296.6, 296.61, 296.61, 296.6, 296.6, 296.57, 296.62, 296.58, 296.59, 296.58, 296.61, 296.62, 296.57, 296.61, 296.63, 296.62, 296.64, 296.63, 296.6, 296.6, 296.57, 296.59, 296.59, 296.6, 296.59, 296.56, 296.6, 296.59, 296.61, 296.59, 296.58, 296.57, 296.59, 296.62, 296.59, 296.61, 296.6, 296.55, 296.6, 296.59, 296.59, 296.6, 296.61, 296.59, 296.57, 296.64, 296.67, 296.57, 296.62, 296.57, 296.58, 296.62, 296.61, 296.58, 296.55, 296.56, 296.59, 296.59, 296.6, 296.58, 296.57, 296.61, 296.58, 296.53, 296.54, 296.59, 296.55, 296.53, 296.59, 296.58, 296.58, 296.58, 296.55, 296.56, 296.56, 296.59, 296.53, 296.61, 296.62, 296.6, 296.58, 296.56, 296.53, 296.55, 296.59, 296.58, 296.6, 296.55, 296.59, 296.56, 296.56, 296.58, 296.57, 296.61, 296.55, 296.61, 296.57, 296.57, 296.58, 296.51, 296.55, 296.6, 296.6, 296.58, 296.56, 296.58, 296.57, 296.59, 296.55, 296.55, 296.56, 296.59, 296.52, 296.54, 296.58, 296.52, 296.54, 296.57, 296.54, 296.59, 296.52, 296.53, 296.55, 296.49, 296.54, 296.63, 296.56, 296.53, 296.54, 296.55, 296.58, 296.56, 296.51, 296.55, 296.57, 296.53, 296.52, 296.56, 296.58, 296.55, 296.61, 296.55, 296.58, 296.53, 296.58, 296.57, 296.52, 296.48, 296.53, 296.52, 296.54, 296.59, 296.53, 296.56, 296.55, 296.58, 296.56, 296.51, 296.52, 296.57, 296.54, 296.55, 296.55, 296.57, 296.59, 296.6, 296.55, 296.54, 296.51, 296.52, 296.55, 296.55, 296.54, 296.51, 296.49, 296.57, 296.55, 296.54, 296.56, 296.55, 296.53, 296.5, 296.55, 296.53, 296.54, 296.57, 296.52, 296.55, 296.55, 296.52, 296.5, 296.53, 296.53, 296.52, 296.54, 296.53, 296.52, 296.53, 296.51, 296.58, 296.49, 296.52, 296.55, 296.48, 296.51, 296.55, 296.48, 296.55, 296.5, 296.51, 296.55, 296.52, 296.54, 296.5, 296.54, 296.52, 296.53, 296.55, 296.53, 296.48, 296.58, 296.55, 296.52, 296.51, 296.49, 296.53, 296.5, 296.56, 296.53, 296.48, 296.54, 296.52, 296.56, 296.53, 296.5, 296.51, 296.5, 296.51, 296.47, 296.47, 296.57, 296.53, 296.49, 296.56, 296.55, 296.55, 296.51, 296.5, 296.52, 296.52, 296.48, 296.51, 296.54, 296.5, 296.49, 296.55, 296.5, 296.52, 296.54, 296.5, 296.51, 296.5, 296.53, 296.49, 296.51, 296.49, 296.54, 296.5, 296.51, 296.5, 296.54, 296.5, 296.48, 296.46, 296.5, 296.49, 296.49, 296.49, 296.51, 296.47, 296.49, 296.47, 296.49, 296.47, 296.49, 296.46, 296.49, 296.47, 296.51]}, {array[312 elements], [0.0, 246.36, 246.3, 246.25, 246.18, 246.13, 246.13, 246.1, 246.04, 246.01, 245.96, 245.88, 245.85, 245.76, 245.73, 245.71, 245.65, 245.59, 245.54, 245.5, 245.46, 245.41, 245.35, 245.32, 245.31, 245.24, 245.17, 245.15, 245.05, 245.05, 244.99, 244.94, 244.92, 244.85, 244.84, 244.72, 244.69, 244.62, 244.56, 244.56, 244.49, 244.46, 244.4, 244.4, 244.3, 244.3, 244.25, 244.17, 244.13, 244.08, 244.03, 243.99, 243.95, 243.89, 243.86, 243.79, 243.75, 243.69, 243.65, 243.6, 243.56, 243.49, 243.42, 243.43, 243.36, 243.34, 243.27, 243.21, 243.12, 243.17, 243.07, 243.05, 242.97, 242.87, 242.88, 242.8, 242.77, 242.72, 242.65, 242.64, 242.55, 242.51, 242.45, 242.46, 242.37, 242.29, 242.28, 242.21, 242.18, 242.14, 242.06, 242.07, 242.0, 241.92, 241.91, 241.84, 241.77, 241.71, 241.66, 241.64, 241.57, 241.52, 241.46, 241.4, 241.37, 241.32, 241.26, 241.23, 241.17, 241.15, 241.07, 241.0, 240.93, 240.92, 240.86, 240.78, 240.76, 240.7, 240.65, 240.57, 240.51, 240.46, 240.46, 240.37, 240.33, 240.29, 240.19, 240.16, 240.13, 240.09, 240.0, 239.96, 239.91, 239.87, 239.83, 239.75, 239.71, 239.63, 239.57, 239.52, 239.48, 239.39, 239.35, 239.35, 239.29, 239.2, 239.19, 239.07, 239.04, 239.02, 238.97, 238.87, 238.8, 238.79, 238.73, 238.67, 238.61, 238.57, 238.54, 238.45, 238.38, 238.36, 238.28, 238.24, 238.21, 238.17, 238.09, 238.05, 237.98, 237.95, 237.88, 237.82, 237.8, 237.73, 237.64, 237.6, 237.58, 237.52, 237.49, 237.43, 237.33, 237.29, 237.26, 237.22, 237.17, 237.11, 237.06, 237.01, 236.97, 236.91, 236.84, 236.8, 236.75, 236.69, 236.64, 236.56, 236.53, 236.45, 236.43, 236.38, 236.33, 236.28, 236.23, 236.16, 236.13, 236.07, 236.01, 235.93, 235.93, 235.88, 235.82, 235.78, 235.72, 235.63, 235.6, 235.57, 235.52, 235.47, 235.43, 235.34, 235.32, 235.25, 235.23, 235.16, 235.11, 235.07, 235.02, 234.92, 234.93, 234.85, 234.8, 234.75, 234.71, 234.65, 234.62, 234.52, 234.5, 234.47, 234.42, 234.38, 234.32, 234.23, 234.19, 234.14, 234.08, 234.06, 234.03, 233.95, 233.91, 233.85, 233.79, 233.74, 233.73, 233.68, 233.61, 233.58, 233.51, 233.46, 233.41, 233.36, 233.32, 233.27, 233.24, 233.16, 233.11, 233.11, 233.03, 232.95, 232.9, 232.89, 232.8, 232.8, 232.72, 232.69, 232.65, 232.58, 232.52, 232.5, 232.44, 232.38, 232.34, 232.26, 232.21, 232.17, 232.13, 232.11, 232.03, 231.97, 231.96, 231.91, 231.88, 231.82, 231.77, 231.7, 231.65, 231.59, 231.59, 231.49, 231.49, 231.38, 231.35, 231.31, 231.25, 231.21, 231.19, 231.16, 231.09, 230.99, 230.97, 230.95, 230.89, 230.81]}, {array[312 elements], [0.0, 251.98, 251.95, 251.89, 251.86, 251.82, 251.77, 251.73, 251.67, 251.64, 251.61, 251.56, 251.51, 251.45, 251.42, 251.36, 251.34, 251.3, 251.22, 251.19, 251.19, 251.14, 251.06, 251.04, 250.98, 250.95, 250.91, 250.87, 250.82, 250.77, 250.74, 250.67, 250.65, 250.6, 250.55, 250.52, 250.46, 250.41, 250.37, 250.34, 250.28, 250.24, 250.21, 250.15, 250.11, 250.08, 250.04, 249.99, 249.94, 249.87, 249.85, 249.81, 249.77, 249.73, 249.67, 249.63, 249.58, 249.55, 249.48, 249.47, 249.4, 249.35, 249.32, 249.28, 249.25, 249.19, 249.15, 249.1, 249.05, 249.01, 248.98, 248.92, 248.85, 248.82, 248.79, 248.76, 248.71, 248.65, 248.6, 248.55, 248.52, 248.47, 248.44, 248.38, 248.36, 248.3, 248.26, 248.19, 248.13, 248.12, 248.06, 248.03, 247.98, 247.93, 247.86, 247.85, 247.82, 247.74, 247.7, 247.66, 247.63, 247.58, 247.54, 247.48, 247.43, 247.4, 247.33, 247.3, 247.25, 247.2, 247.16, 247.1, 247.09, 247.02, 246.96, 246.93, 246.88, 246.85, 246.79, 246.76, 246.7, 246.66, 246.6, 246.58, 246.53, 246.47, 246.44, 246.4, 246.34, 246.28, 246.23, 246.18, 246.14, 246.1, 246.05, 246.01, 245.98, 245.94, 245.86, 245.85, 245.79, 245.72, 245.68, 245.65, 245.62, 245.54, 245.52, 245.46, 245.42, 245.37, 245.3, 245.28, 245.23, 245.15, 245.13, 245.08, 245.03, 244.97, 244.94, 244.89, 244.87, 244.8, 244.75, 244.71, 244.65, 244.62, 244.59, 244.53, 244.48, 244.4, 244.38, 244.32, 244.29, 244.25, 244.18, 244.15, 244.11, 244.06, 244.03, 243.93, 243.92, 243.85, 243.82, 243.75, 243.73, 243.67, 243.63, 243.57, 243.52, 243.49, 243.44, 243.38, 243.33, 243.29, 243.25, 243.21, 243.15, 243.11, 243.06, 243.0, 242.97, 242.92, 242.86, 242.83, 242.76, 242.74, 242.67, 242.61, 242.58, 242.55, 242.47, 242.45, 242.39, 242.34, 242.3, 242.25, 242.21, 242.16, 242.12, 242.06, 242.01, 241.94, 241.91, 241.86, 241.82, 241.76, 241.71, 241.67, 241.59, 241.56, 241.5, 241.48, 241.42, 241.38, 241.33, 241.29, 241.22, 241.18, 241.15, 241.09, 241.05, 241.0, 240.93, 240.9, 240.85, 240.8, 240.75, 240.71, 240.65, 240.62, 240.55, 240.52, 240.47, 240.41, 240.36, 240.3, 240.28, 240.21, 240.17, 240.11, 240.07, 240.03, 239.98, 239.93, 239.88, 239.83, 239.8, 239.73, 239.67, 239.63, 239.6, 239.54, 239.5, 239.42, 239.41, 239.36, 239.3, 239.24, 239.21, 239.16, 239.11, 239.04, 239.01, 238.94, 238.9, 238.85, 238.81, 238.76, 238.7, 238.67, 238.62, 238.56, 238.51, 238.48, 238.41, 238.38, 238.33, 238.28, 238.24, 238.17, 238.12, 238.07, 238.03, 237.95, 237.93, 237.88, 237.85, 237.78, 237.73, 237.68, 237.64, 237.57]}, {array[312 elements], [0.0, 22.529, 22.52, 22.516, 22.495, 22.486, 22.467, 22.467, 22.454, 22.443, 22.422, 22.419, 22.404, 22.383, 22.383, 22.362, 22.365, 22.347, 22.331, 22.329, 22.31, 22.305, 22.302, 22.294, 22.273, 22.277, 22.26, 22.241, 22.238, 22.231, 22.225, 22.194, 22.193, 22.182, 22.171, 22.163, 22.164, 22.165, 22.157, 22.138, 22.136, 22.124, 22.112, 22.109, 22.094, 22.078, 22.077, 22.076, 22.066, 22.067, 22.046, 22.048, 22.04, 22.032, 22.017, 22.004, 21.995, 21.997, 21.999, 21.975, 21.967, 21.961, 21.956, 21.949, 21.941, 21.93, 21.929, 21.91, 21.917, 21.916, 21.899, 21.888, 21.886, 21.878, 21.864, 21.846, 21.845, 21.839, 21.831, 21.821, 21.814, 21.797, 21.805, 21.796, 21.795, 21.776, 21.766, 21.78, 21.769, 21.767, 21.756, 21.738, 21.753, 21.729, 21.736, 21.73, 21.716, 21.707, 21.704, 21.702, 21.703, 21.689, 21.682, 21.682, 21.674, 21.661, 21.655, 21.66, 21.656, 21.646, 21.647, 21.634, 21.63, 21.626, 21.613, 21.616, 21.604, 21.603, 21.602, 21.592, 21.593, 21.589, 21.579, 21.575, 21.568, 21.561, 21.555, 21.557, 21.547, 21.541, 21.535, 21.531, 21.532, 21.53, 21.526, 21.523, 21.509, 21.503, 21.509, 21.501, 21.491, 21.505, 21.496, 21.496, 21.482, 21.483, 21.483, 21.473, 21.478, 21.485, 21.47, 21.473, 21.461, 21.459, 21.454, 21.442, 21.453, 21.462, 21.462, 21.456, 21.445, 21.445, 21.453, 21.457, 21.449, 21.449, 21.442, 21.447, 21.444, 21.446, 21.443, 21.446, 21.446, 21.449, 21.446, 21.449, 21.45, 21.455, 21.45, 21.446, 21.444, 21.442, 21.451, 21.44, 21.433, 21.45, 21.432, 21.441, 21.441, 21.44, 21.443, 21.43, 21.424, 21.421, 21.42, 21.43, 21.427, 21.416, 21.405, 21.406, 21.406, 21.414, 21.404, 21.417, 21.414, 21.406, 21.393, 21.401, 21.4, 21.393, 21.38, 21.369, 21.372, 21.379, 21.364, 21.376, 21.364, 21.347, 21.35, 21.365, 21.361, 21.346, 21.335, 21.349, 21.336, 21.321, 21.336, 21.331, 21.342, 21.335, 21.31, 21.331, 21.314, 21.324, 21.317, 21.292, 21.316, 21.282, 21.305, 21.298, 21.3, 21.286, 21.291, 21.278, 21.282, 21.28, 21.276, 21.255, 21.262, 21.269, 21.256, 21.241, 21.245, 21.239, 21.225, 21.233, 21.228, 21.23, 21.218, 21.218, 21.211, 21.215, 21.212, 21.213, 21.21, 21.2, 21.209, 21.204, 21.188, 21.2, 21.185, 21.18, 21.181, 21.166, 21.162, 21.166, 21.161, 21.139, 21.152, 21.143, 21.138, 21.131, 21.138, 21.133, 21.132, 21.123, 21.12, 21.119, 21.114, 21.107, 21.108, 21.1, 21.089, 21.091, 21.082, 21.083, 21.083, 21.073, 21.072, 21.059, 21.055, 21.048, 21.04, 21.044, 21.035, 21.02, 21.025, 21.009, 21.019, 21.009, 21.001, 20.995]}, {array[312 elements], [0.0, 4.244, 4.243, 4.243, 4.243, 4.243, 4.243, 4.243, 4.243, 4.243, 4.243, 4.243, 4.243, 4.243, 4.242, 4.243, 4.243, 4.243, 4.243, 4.242, 4.244, 4.243, 4.244, 4.243, 4.242, 4.243, 4.243, 4.243, 4.243, 4.243, 4.243, 4.243, 4.243, 4.243, 4.243, 4.243, 4.243, 4.243, 4.243, 4.243, 4.244, 4.244, 4.243, 4.243, 4.243, 4.244, 4.243, 4.243, 4.243, 4.243, 4.243, 4.243, 4.242, 4.243, 4.243, 4.243, 4.243, 4.243, 4.243, 4.243, 4.243, 4.243, 4.243, 4.243, 4.243, 4.243, 4.242, 4.243, 4.243, 4.242, 4.242, 4.242, 4.243, 4.243, 4.242, 4.243, 4.243, 4.242, 4.243, 4.243, 4.242, 4.243, 4.243, 4.243, 4.243, 4.243, 4.242, 4.243, 4.242, 4.242, 4.243, 4.243, 4.243, 4.242, 4.242, 4.243, 4.243, 4.242, 4.242, 4.242, 4.242, 4.242, 4.243, 4.243, 4.243, 4.243, 4.243, 4.243, 4.243, 4.243, 4.243, 4.242, 4.243, 4.243, 4.243, 4.242, 4.243, 4.242, 4.243, 4.243, 4.243, 4.243, 4.242, 4.242, 4.242, 4.243, 4.242, 4.243, 4.243, 4.242, 4.242, 4.242, 4.242, 4.242, 4.243, 4.243, 4.243, 4.242, 4.242, 4.242, 4.242, 4.243, 4.242, 4.242, 4.242, 4.242, 4.242, 4.242, 4.242, 4.243, 4.243, 4.242, 4.242, 4.242, 4.242, 4.242, 4.243, 4.242, 4.243, 4.243, 4.242, 4.242, 4.242, 4.242, 4.242, 4.243, 4.242, 4.243, 4.243, 4.243, 4.242, 4.243, 4.242, 4.243, 4.243, 4.242, 4.242, 4.242, 4.242, 4.242, 4.242, 4.242, 4.242, 4.242, 4.242, 4.242, 4.242, 4.242, 4.242, 4.242, 4.242, 4.242, 4.243, 4.242, 4.242, 4.242, 4.243, 4.242, 4.242, 4.242, 4.242, 4.242, 4.243, 4.242, 4.242, 4.242, 4.242, 4.242, 4.242, 4.242, 4.242, 4.242, 4.242, 4.242, 4.243, 4.242, 4.242, 4.242, 4.242, 4.241, 4.242, 4.242, 4.242, 4.242, 4.242, 4.242, 4.242, 4.242, 4.243, 4.242, 4.242, 4.242, 4.242, 4.242, 4.242, 4.242, 4.243, 4.242, 4.242, 4.242, 4.242, 4.241, 4.242, 4.242, 4.242, 4.242, 4.242, 4.242, 4.242, 4.242, 4.242, 4.243, 4.242, 4.242, 4.242, 4.242, 4.242, 4.242, 4.242, 4.242, 4.242, 4.242, 4.242, 4.241, 4.242, 4.241, 4.242, 4.242, 4.242, 4.242, 4.242, 4.242, 4.241, 4.241, 4.242, 4.242, 4.241, 4.241, 4.241, 4.242, 4.241, 4.242, 4.242, 4.242, 4.242, 4.242, 4.242, 4.242, 4.242, 4.242, 4.242, 4.242, 4.242, 4.241, 4.242, 4.242, 4.241, 4.242, 4.242, 4.242, 4.242, 4.241, 4.242, 4.241, 4.242, 4.242, 4.241, 4.242, 4.242, 4.241, 4.242, 4.242]}, {array[312 elements], [0.0, 6.751, 6.741, 6.737, 6.736, 6.748, 6.752, 6.743, 6.739, 6.737, 6.744, 6.752, 6.753, 6.747, 6.741, 6.737, 6.737, 6.741, 6.748, 6.755, 6.756, 6.755, 6.75, 6.748, 6.745, 6.744, 6.743, 6.746, 6.75, 6.755, 6.761, 6.761, 6.758, 6.752, 6.75, 6.747, 6.747, 6.745, 6.745, 6.747, 6.753, 6.756, 6.764, 6.764, 6.763, 6.76, 6.755, 6.754, 6.752, 6.752, 6.752, 6.752, 6.751, 6.751, 6.751, 6.751, 6.753, 6.757, 6.759, 6.76, 6.764, 6.766, 6.766, 6.77, 6.771, 6.769, 6.77, 6.769, 6.769, 6.769, 6.767, 6.768, 6.764, 6.764, 6.763, 6.759, 6.76, 6.759, 6.758, 6.759, 6.76, 6.762, 6.762, 6.763, 6.765, 6.767, 6.769, 6.771, 6.774, 6.779, 6.78, 6.78, 6.782, 6.782, 6.781, 6.777, 6.775, 6.772, 6.77, 6.768, 6.768, 6.771, 6.773, 6.773, 6.777, 6.78, 6.786, 6.788, 6.787, 6.78, 6.776, 6.773, 6.774, 6.776, 6.78, 6.786, 6.789, 6.79, 6.785, 6.776, 6.775, 6.778, 6.781, 6.788, 6.793, 6.79, 6.78, 6.775, 6.778, 6.782, 6.79, 6.794, 6.789, 6.78, 6.78, 6.782, 6.786, 6.795, 6.796, 6.788, 6.782, 6.784, 6.787, 6.794, 6.8, 6.792, 6.785, 6.788, 6.797, 6.802, 6.796, 6.785, 6.786, 6.79, 6.802, 6.8, 6.788, 6.789, 6.794, 6.804, 6.804, 6.792, 6.791, 6.795, 6.804, 6.804, 6.793, 6.792, 6.795, 6.803, 6.807, 6.796, 6.792, 6.797, 6.807, 6.8, 6.792, 6.799, 6.808, 6.797, 6.793, 6.803, 6.81, 6.794, 6.798, 6.809, 6.807, 6.797, 6.802, 6.812, 6.807, 6.816, 6.829, 6.84, 6.828, 6.828, 6.838, 6.838, 6.826, 6.831, 6.843, 6.831, 6.83, 6.84, 6.841, 6.828, 6.835, 6.846, 6.831, 6.833, 6.846, 6.839, 6.834, 6.842, 6.843, 6.833, 6.842, 6.849, 6.833, 6.843, 6.849, 6.834, 6.842, 6.85, 6.835, 6.843, 6.848, 6.836, 6.842, 6.849, 6.837, 6.848, 6.848, 6.839, 6.851, 6.846, 6.84, 6.85, 6.844, 6.841, 6.853, 6.84, 6.844, 6.856, 6.841, 6.845, 6.857, 6.84, 6.85, 6.85, 6.843, 6.856, 6.847, 6.845, 6.858, 6.844, 6.848, 6.858, 6.846, 6.858, 6.843, 6.852, 6.852, 6.846, 6.859, 6.845, 6.853, 6.853, 6.848, 6.86, 6.846, 6.858, 6.847, 6.852, 6.854, 6.849, 6.863, 6.848, 6.861, 6.847, 6.856, 6.855, 6.852, 6.861, 6.85, 6.864, 6.848, 6.863, 6.85, 6.854, 6.859, 6.851, 6.865, 6.851, 6.865, 6.851, 6.864, 6.853, 6.859, 6.855, 6.859, 6.862, 6.857, 6.867, 6.856, 6.869, 6.856, 6.87, 6.855, 6.871, 6.855, 6.869]}, {array[312 elements], [0.0, 295.97, 296.04, 295.97, 296.06, 295.86, 295.93, 296.04, 295.99, 296.15, 295.97, 296.14, 296.11, 296.03, 296.06, 296.03, 296.11, 296.2, 295.93, 296.04, 295.99, 296.02, 295.99, 296.1, 296.14, 295.73, 296.02, 296.15, 296.14, 295.92, 296.02, 296.15, 296.0, 296.04, 296.15, 296.25, 296.31, 296.02, 296.13, 296.22, 296.37, 296.22, 296.27, 296.35, 296.13, 296.22, 295.7, 296.18, 295.95, 296.22, 296.39, 296.14, 296.25, 296.1, 296.15, 296.13, 296.2, 296.14, 296.23, 296.2, 296.2, 296.06, 296.18, 296.27, 296.42, 296.31, 296.31, 296.31, 296.11, 296.22, 296.16, 296.23, 296.33, 296.14, 296.06, 296.43, 296.31, 296.2, 296.16, 296.13, 296.4, 296.23, 296.5, 296.4, 296.31, 296.1, 296.51, 296.42, 296.37, 296.43, 296.4, 296.31, 296.27, 296.54, 296.36, 296.27, 296.44, 296.35, 296.27, 296.42, 296.22, 296.43, 296.31, 296.54, 296.55, 296.4, 296.39, 296.31, 296.33, 296.5, 296.5, 296.44, 296.53, 296.47, 296.36, 296.49, 296.44, 296.58, 296.36, 296.31, 296.47, 296.49, 296.25, 296.47, 296.66, 296.51, 296.4, 296.49, 296.49, 296.18, 296.47, 296.56, 296.51, 296.55, 296.62, 296.6, 296.6, 296.47, 296.47, 296.58, 296.63, 296.58, 296.58, 296.56, 296.6, 296.47, 296.42, 296.37, 296.42, 296.49, 296.37, 296.53, 296.5, 296.6, 296.56, 296.63, 296.71, 296.58, 296.51, 296.43, 296.77, 296.36, 296.63, 296.44, 296.73, 296.73, 296.6, 296.74, 296.5, 296.51, 296.5, 296.42, 296.65, 296.58, 296.4, 296.31, 296.53, 296.43, 296.69, 296.66, 296.65, 296.62, 296.71, 296.6, 296.35, 296.7, 296.65, 296.6, 296.67, 296.63, 296.78, 296.91, 296.86, 296.69, 296.74, 296.55, 296.6, 296.91, 296.76, 296.67, 296.76, 296.71, 296.94, 296.63, 296.86, 296.63, 296.7, 296.82, 296.8, 296.74, 296.74, 296.73, 296.96, 296.76, 296.74, 296.8, 296.84, 296.86, 296.83, 296.77, 296.89, 296.65, 296.77, 296.84, 296.71, 296.76, 296.74, 296.89, 296.8, 296.74, 296.82, 296.87, 296.8, 297.0, 297.16, 297.09, 296.98, 296.83, 296.89, 296.89, 296.54, 296.89, 296.78, 296.87, 297.21, 297.14, 296.78, 296.73, 296.87, 297.14, 297.03, 297.14, 297.1, 297.09, 297.02, 296.78, 297.25, 297.21, 297.0, 297.03, 296.98, 296.94, 296.93, 296.93, 297.03, 297.07, 296.89, 297.05, 297.02, 296.98, 296.95, 296.96, 296.87, 296.95, 297.07, 297.13, 296.96, 297.07, 297.0, 297.16, 297.17, 297.05, 296.93, 296.91, 297.07, 296.98, 297.1, 297.03, 297.19, 297.05, 297.0, 297.07, 297.16, 297.13, 297.0, 297.21, 296.94, 297.3, 297.05, 297.12, 297.28, 297.21, 297.17, 297.23, 297.25, 297.25, 297.21, 297.21, 297.13, 297.17, 297.29, 297.3]}, {array[312 elements], [0.0, 281.87, 284.61, 281.99, 283.5, 282.29, 284.54, 281.98, 283.46, 284.72, 281.54, 282.9, 285.03, 283.14, 281.87, 281.54, 283.76, 284.61, 283.77, 283.35, 282.81, 281.49, 282.64, 284.24, 282.04, 283.31, 281.38, 284.43, 281.46, 284.59, 281.26, 283.93, 282.21, 282.76, 283.46, 282.65, 284.47, 281.69, 284.72, 282.51, 283.24, 282.89, 283.52, 281.43, 284.24, 281.77, 282.2, 284.47, 282.72, 282.56, 284.67, 281.3, 283.69, 282.76, 281.24, 284.17, 281.24, 283.14, 282.61, 281.26, 283.55, 282.98, 281.62, 283.87, 282.12, 282.56, 284.26, 281.95, 284.13, 281.11, 283.82, 280.96, 283.39, 282.37, 281.73, 283.39, 282.29, 283.76, 282.07, 283.87, 282.21, 282.35, 283.01, 281.11, 284.39, 281.29, 283.77, 281.26, 283.8, 280.91, 284.29, 281.18, 283.31, 281.79, 284.37, 282.32, 283.14, 282.61, 282.51, 283.77, 281.74, 283.06, 281.43, 284.09, 282.35, 281.98, 284.26, 282.65, 281.95, 284.88, 283.01, 281.07, 284.18, 283.55, 281.3, 282.68, 283.9, 283.11, 281.65, 282.59, 283.47, 283.01, 282.43, 281.41, 282.95, 284.1, 282.89, 281.13, 284.54, 282.24, 282.72, 282.68, 283.46, 281.74, 283.85, 283.03, 282.64, 283.01, 283.11, 282.17, 283.87, 281.82, 284.02, 282.12, 283.16, 284.39, 281.65, 284.13, 281.21, 283.47, 283.72, 281.49, 282.76, 284.77, 282.15, 282.4, 283.52, 284.13, 283.31, 282.28, 281.85, 282.9, 283.9, 284.29, 284.54, 284.51, 283.85, 283.03, 283.11, 283.9, 284.51, 282.98, 283.47, 284.67, 281.99, 282.53, 284.42, 283.31, 282.15, 284.8, 283.93, 281.66, 283.11, 284.8, 282.9, 283.35, 283.39, 282.61, 283.16, 281.73, 281.38, 283.76, 284.81, 284.81, 283.5, 283.01, 284.72, 282.53, 284.64, 282.83, 284.24, 282.83, 283.8, 283.82, 282.04, 284.13, 284.13, 282.59, 283.42, 285.13, 282.59, 281.99, 283.31, 282.32, 282.95, 283.16, 283.39, 284.54, 284.42, 281.66, 282.61, 284.39, 282.98, 281.54, 285.03, 283.38, 282.56, 284.72, 283.08, 282.76, 284.47, 283.08, 282.64, 283.8, 284.88, 284.61, 284.73, 283.63, 281.79, 281.54, 283.24, 283.27, 281.66, 282.61, 283.93, 284.39, 282.37, 283.39, 284.67, 281.91, 284.59, 283.38, 281.82, 284.96, 282.2, 284.88, 281.73, 284.09, 281.74, 285.05, 282.2, 282.45, 284.01, 281.18, 282.9, 282.48, 283.52, 282.98, 283.22, 282.32, 284.13, 283.85, 281.11, 282.37, 284.59, 284.8, 284.59, 282.98, 282.07, 282.28, 282.83, 283.72, 283.38, 282.83, 282.07, 283.01, 282.78, 283.3, 281.49, 283.06, 282.21, 283.39, 281.85, 283.22, 282.28, 283.42, 282.95, 283.64, 281.33, 284.77, 282.29, 282.12, 283.69, 284.05, 281.74, 283.08, 283.72, 282.59, 281.43, 282.59, 282.81, 283.3]}, {array[312 elements], []}]
  out "U idx":i32[](array[numeric])=[0, 1, 2, 3, 4, 5, 6, 7]
  out "RAW (V)":dbl[](array[numeric])=[3.032151866923436, 0.034825050655990085, 2.8213985627597147, 1.7252180376553732, 1.7220945469955173, -0.0027308305231602686, 0.00973684653660363, -0.00010051949347097966, 3.9496354659744695, 4.458928369173362, 5.447101175410158] format="%#_3f"
  out "DAQ CONV. OUT":dbl[](array[numeric])=[101716.09348282787, 34.79347639713247, 458.6457435799443, 181.31272912551344, 173.5870784692008, 0.20508894588428317, 0.14209303805052026, -50008.31386345759, 101793.91904862555, 58185.26026544768, 105090.96406177872] format="%#_9f"
  out "NI-DAQ CH indic.":string[](array[string])=["P_4KRES_COILIN", "LM_110", "DP_4He", "DP_3He", "FM_4He", "FM_3He", "LM_1700", "P_4He_IN", "Bar_anal", "bar_CDG1", "bar_CDG2"]
  out "Graph S. 1":cluster{dbl[], dbl[]}[](graph)
  in  "log/linear 4":bool
  in  "log/linear 1":bool
  out "Graph S. 3":cluster{dbl[], dbl[]}[](graph)
  in  "log/linear 6":bool
  in  "log/linear 3":bool
  in  "log/linear 2":bool
  out "Graph S. 6":cluster{dbl[], dbl[]}[](graph)
  out "Graph S. 5":cluster{dbl[], dbl[]}[](graph)
  in  "log/linear 5":bool
  in  "S.5 SEL":i32[](array[numeric])=[0, 2, 3]
  out "Graph S. 4":cluster{dbl[], dbl[]}[](graph)
  in  "S.1 SEL":i32[](array[numeric])=[8, 3, 8]
  in  "S.2 SEL":i32[](array[numeric])=[1]
  out "Graph S. 2":cluster{dbl[], dbl[]}[](graph)
  in  "S.3 SEL":i32[](array[numeric])=[0, 2, 3]
  in  "S.4 SEL":i32[](array[numeric])=[0, 2, 3]
  in  "S.6 SEL":i32[](array[numeric])=[0, 2, 3]
  in  "DAQ OUT SET Volt":dbl[](array[numeric])=[2.0] format="%0.2f"
  out "DAQ OUT \nsample #":u32=1
  out "Q idx":i32[](array[numeric])=[0, 1, 2, 3, 4, 5, 6, 7, 8, 9, 10]
  in  "idx 10 Vbar offset":dbl=1.49877
  in  "idx 9 Vbar offset":dbl=0.642064
  in  "idx 8 Vbar offset":dbl=0.0077
  out "V10 - V9":dbl=0.9850821974083006 format="%#_9g"
  out "V9 - V8":dbl=0.5129095731647313 format="%#_9g"
  out "V10 - V8":dbl=1.497991770573032 format="%#_9g"
  out "date/time string":string="20191030_165052_"
  in  "Wait (s)":i32=5
  # "Record Config"
  # "Some time needed until program stops!"
  # "Error states"
  # "Inputs on this page have to be filled before the start of the program"
  # "LSI VISA addresses"
  # "Defines # of measurements \n taken for averaging (only ested w 5)"
  # "NI DAQ OUT"
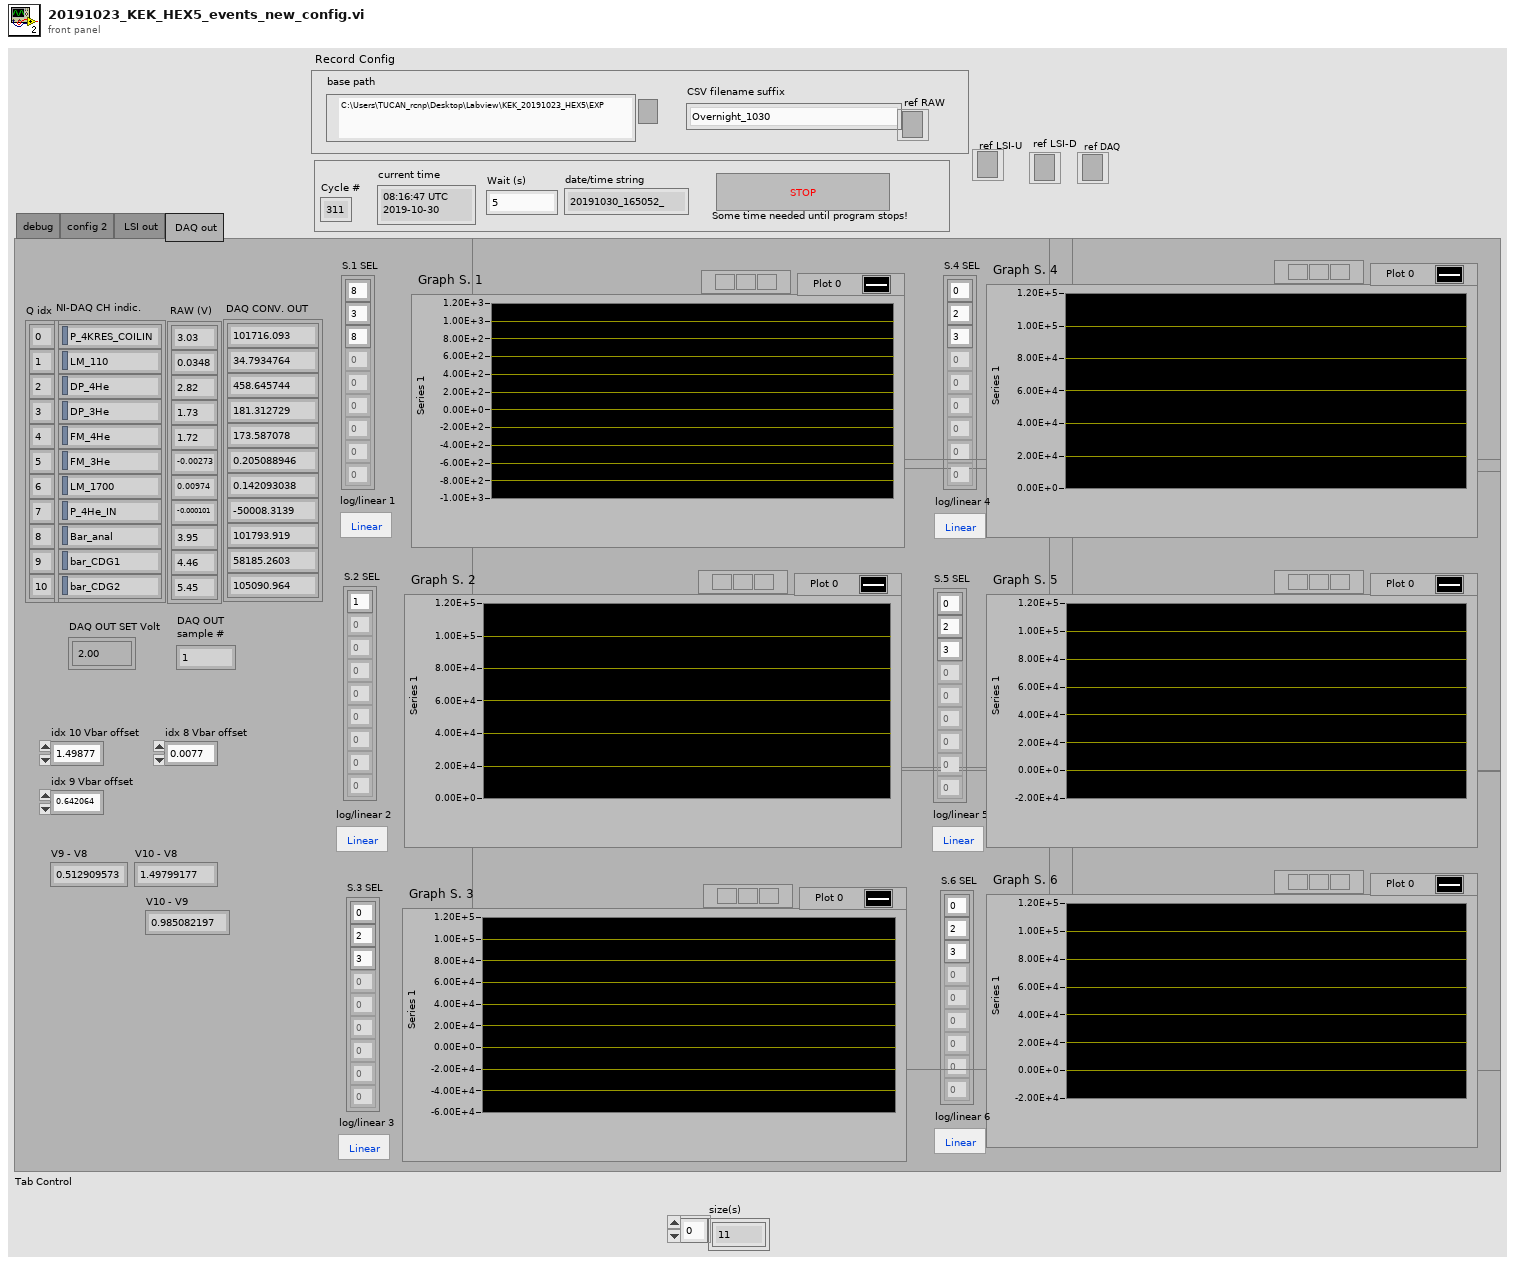
[diagram p1: front panel]
types:
  T1 = enum32{"debug", "config 2", " LSI out", " DAQ out"}
  T2 = enum16{"open", "replace", "create", "open or create", "replace or create", "replace or create with confirmation"}
  T3 = cluster{"LSI-U CH labels[0]":string, "LSI-U CH labels[1]":string, "LSI-U CH labels[2]":string, "LSI-U CH labels[3]":string, "LSI-U CH labels[4]":string, "LSI-U CH labels[5]":string, "LSI-U CH labels[6]":string, "LSI-U CH labels[7]":string, "LSI-U CH labels[8]":string}
  T4 = cluster{"LSI-D CH labels[0]":string, "LSI-D CH labels[1]":string, "LSI-D CH labels[2]":string, "LSI-D CH labels[3]":string, "LSI-D CH labels[4]":string, "LSI-D CH labels[5]":string, "LSI-D CH labels[6]":string, "LSI-D CH labels[7]":string, "LSI-D CH labels[8]":string}
  T5 = cluster{"LSI-D out[0]":dbl, "LSI-D out[1]":dbl, "LSI-D out[2]":dbl, "LSI-D out[3]":dbl, "LSI-D out[4]":dbl, "LSI-D out[5]":dbl, "LSI-D out[6]":dbl, "LSI-D out[7]":dbl, "LSI-D out[8]":dbl}
  T6 = cluster{"LSI-U out[0]":dbl, "LSI-U out[1]":dbl, "LSI-U out[2]":dbl, "LSI-U out[3]":dbl, "LSI-U out[4]":dbl, "LSI-U out[5]":dbl, "LSI-U out[6]":dbl, "LSI-U out[7]":dbl, "LSI-U out[8]":dbl}
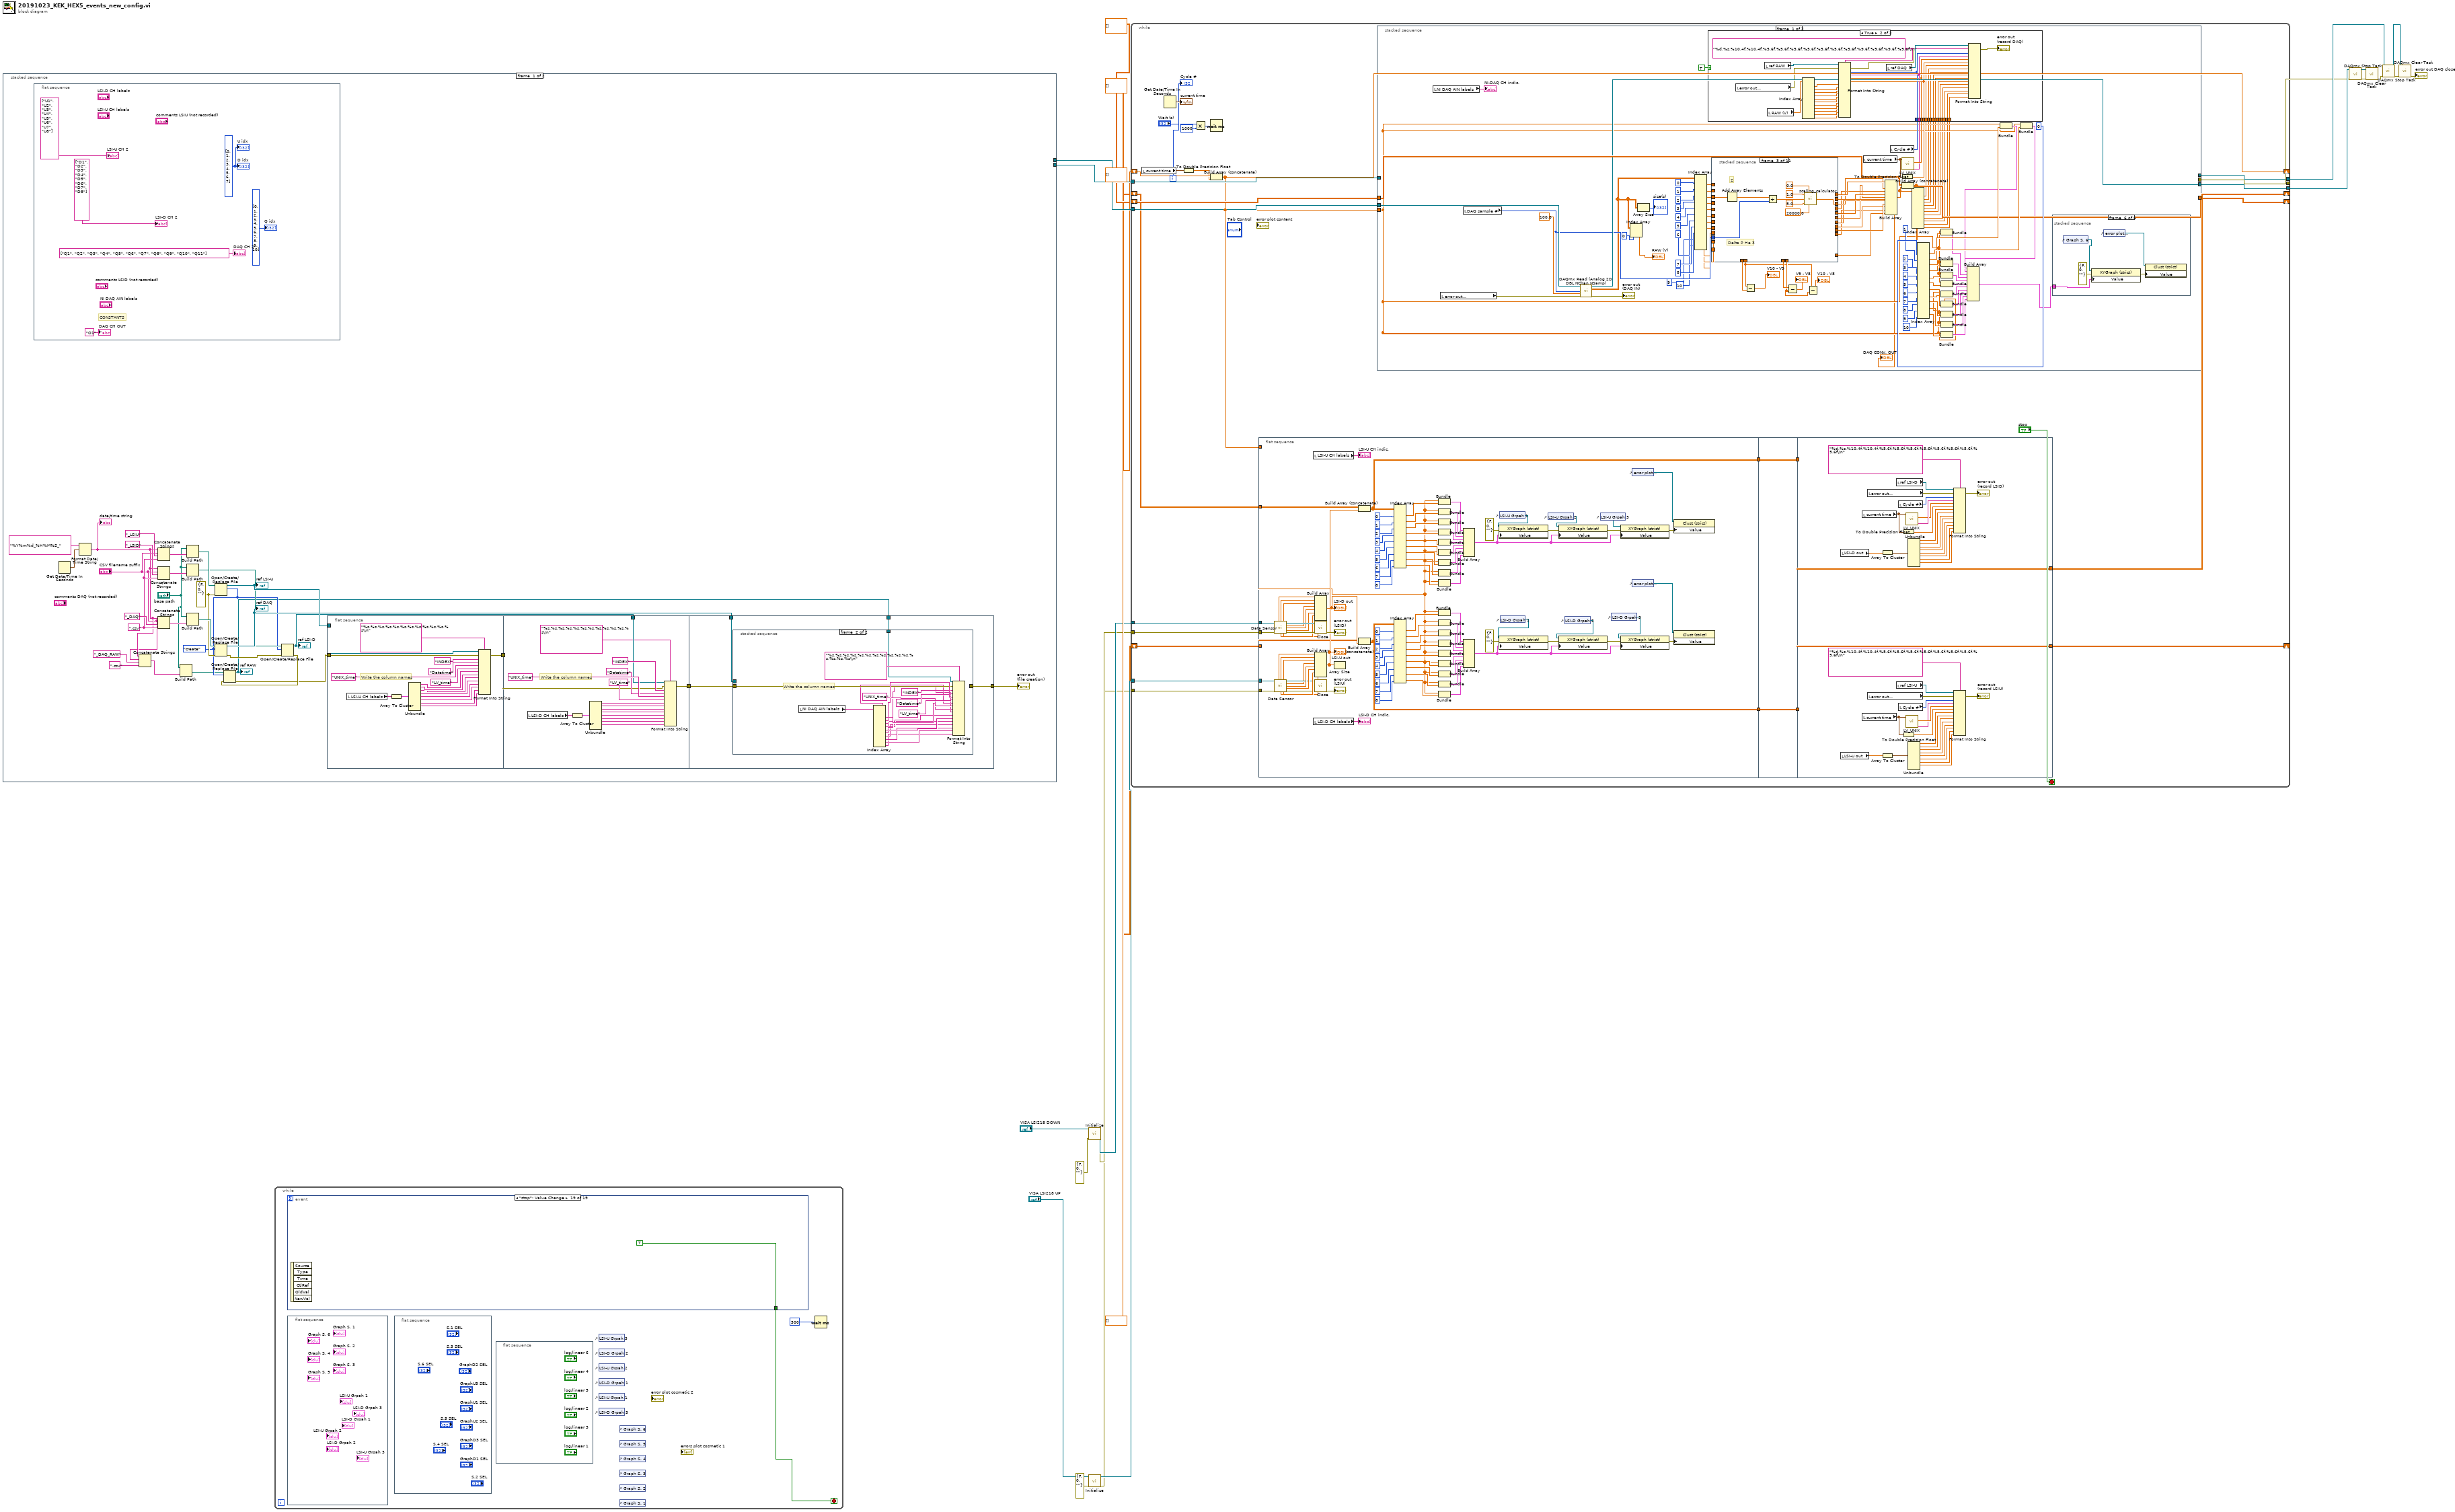
[diagram p0: block diagram]
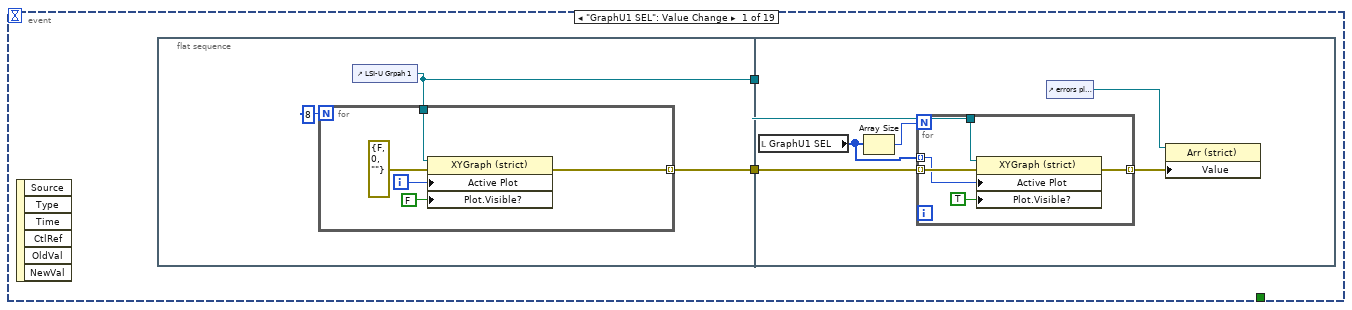
[diagram p2: hidden frame]
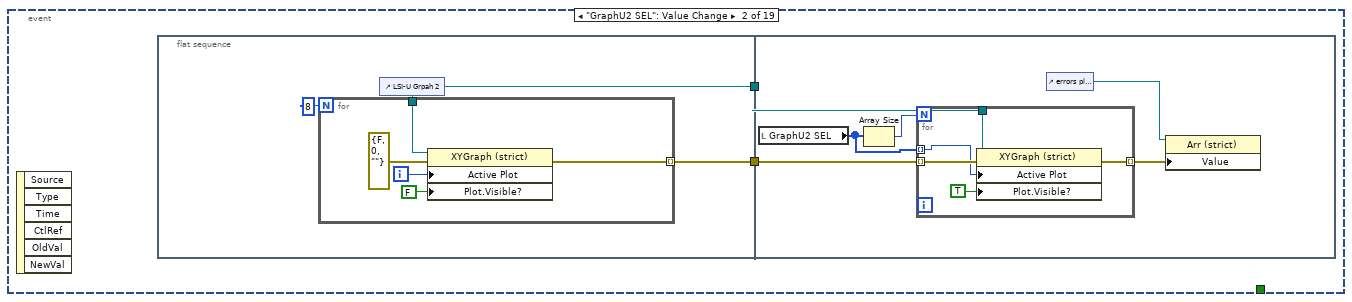
[diagram p3: hidden frame]
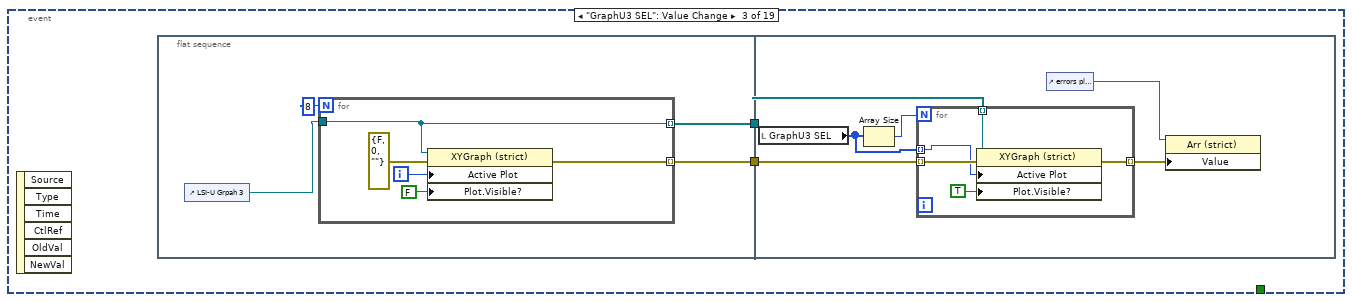
[diagram p4: hidden frame]
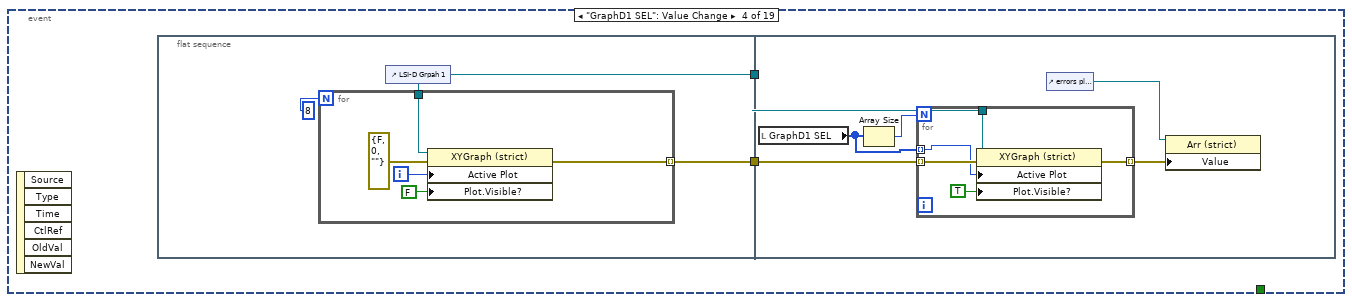
[diagram p5: hidden frame]
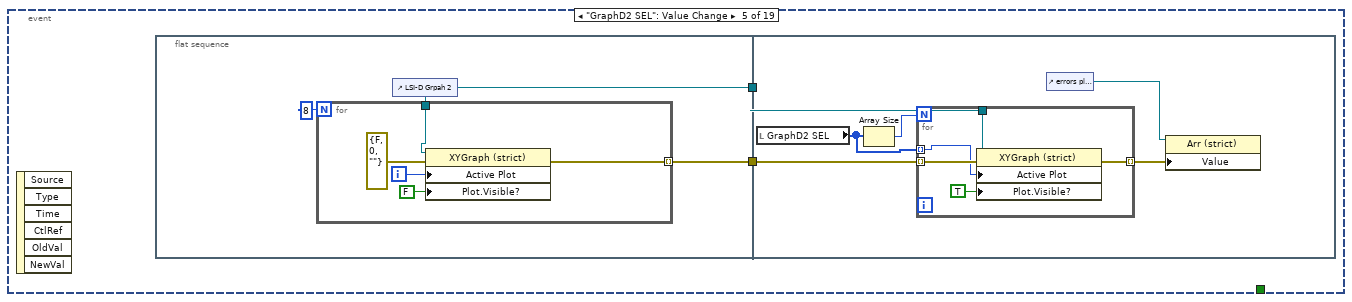
[diagram p6: hidden frame]
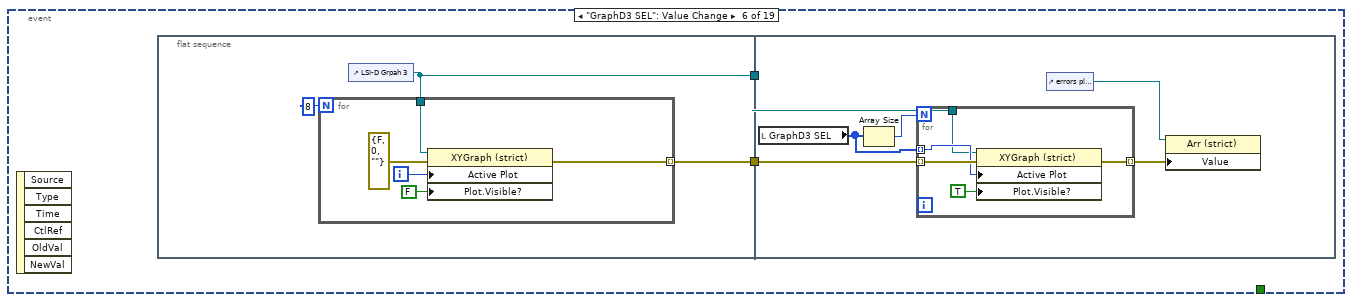
[diagram p7: hidden frame]
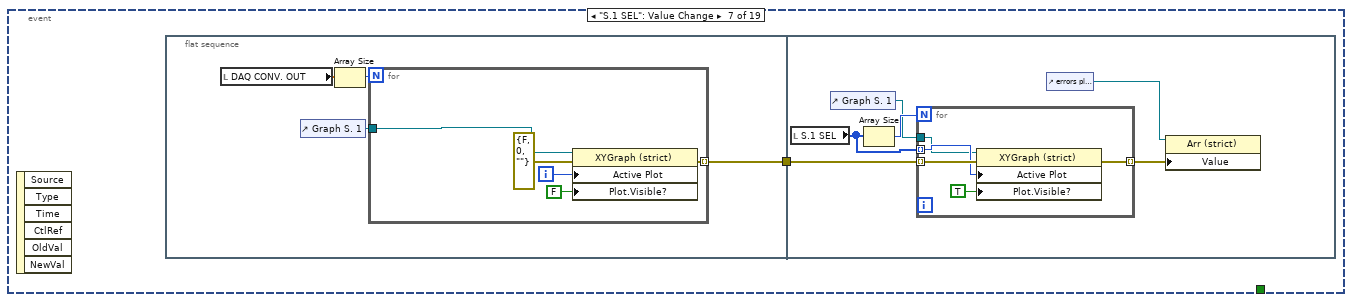
[diagram p8: hidden frame]
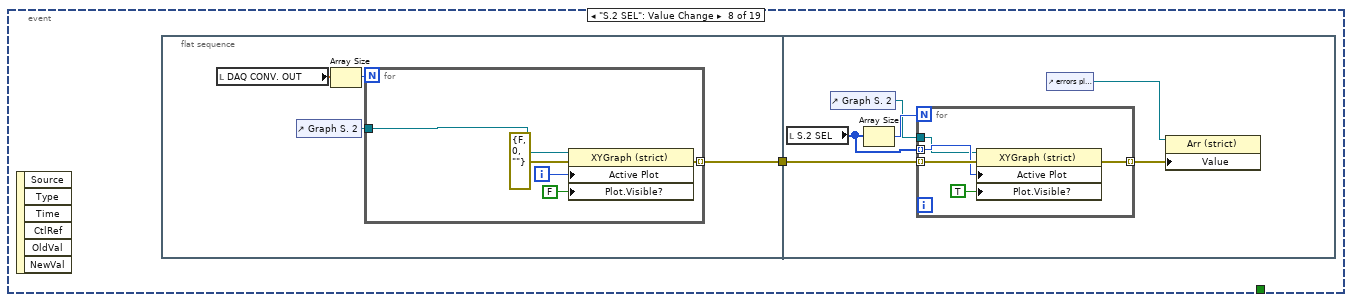
[diagram p9: hidden frame]
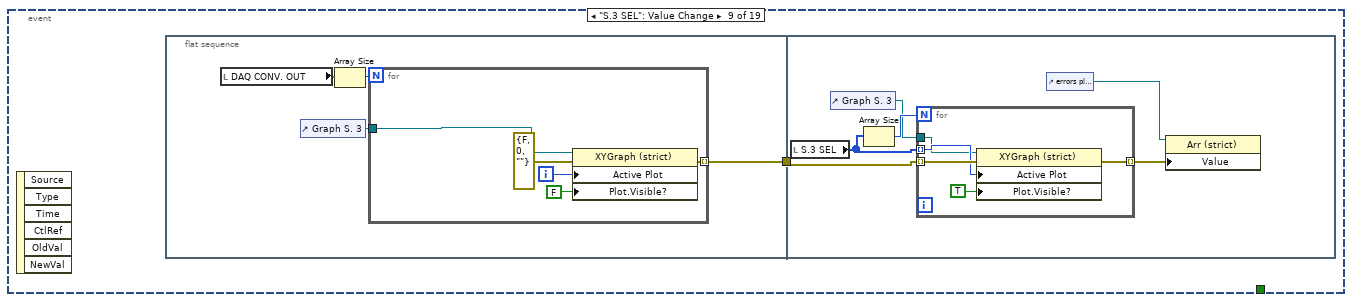
[diagram p10: hidden frame]
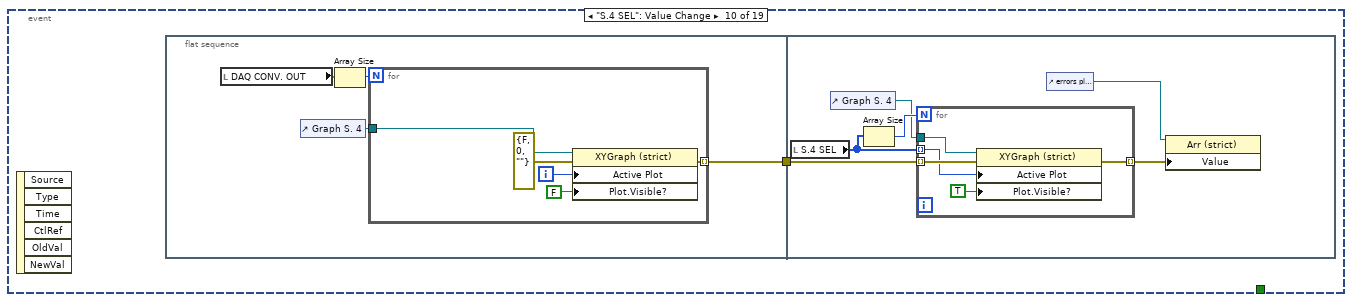
[diagram p11: hidden frame]
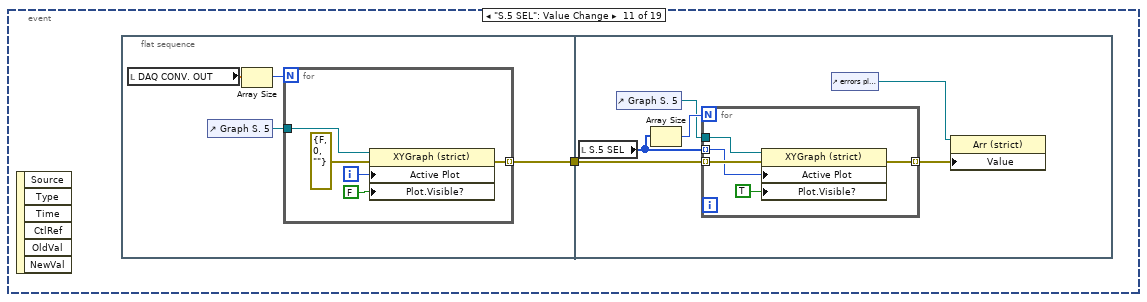
[diagram p12: hidden frame]
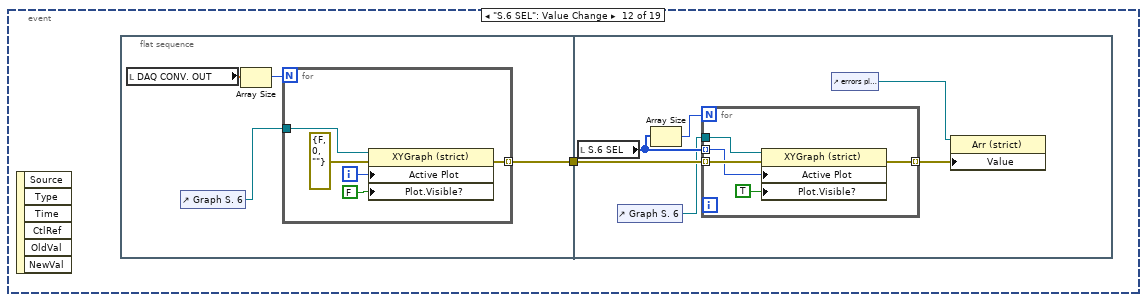
[diagram p13: hidden frame]
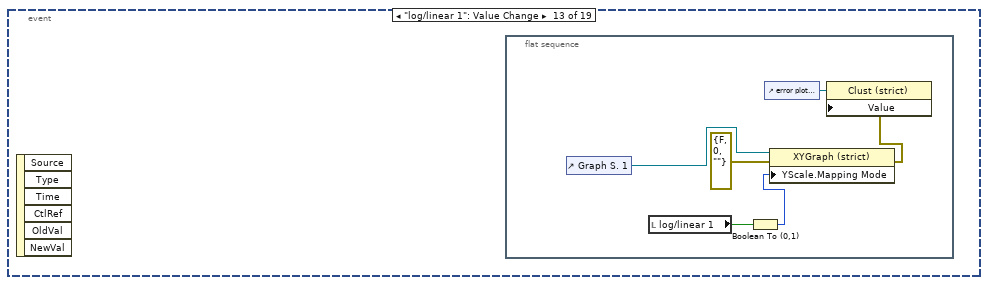
[diagram p14: hidden frame]
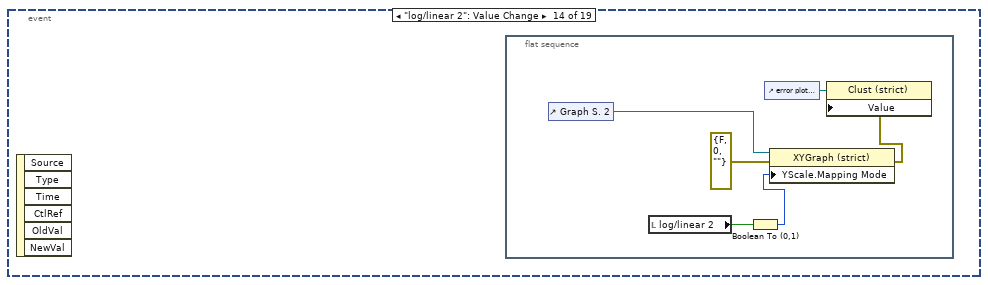
[diagram p15: hidden frame]
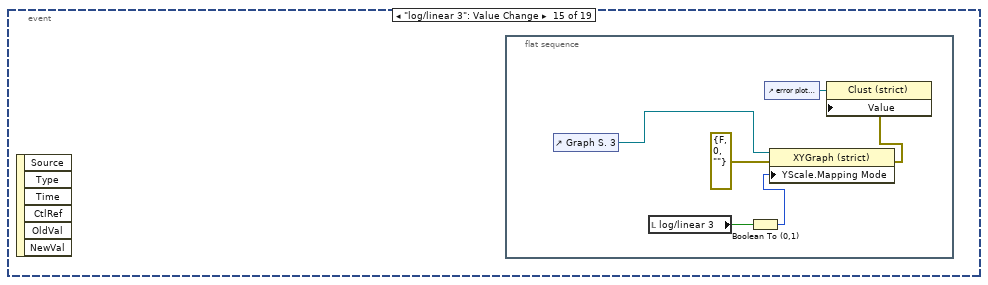
[diagram p16: hidden frame]
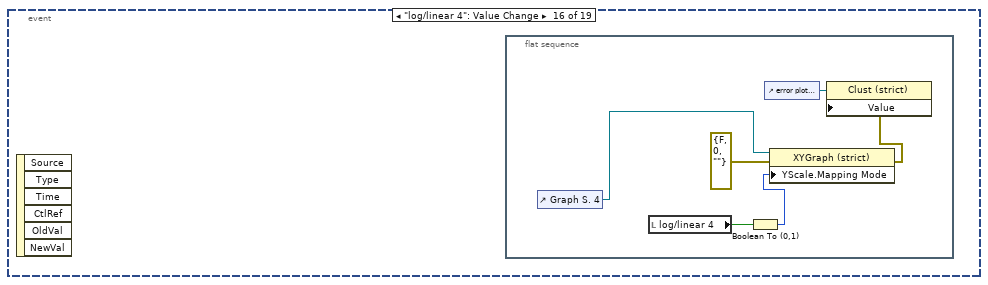
[diagram p17: hidden frame]
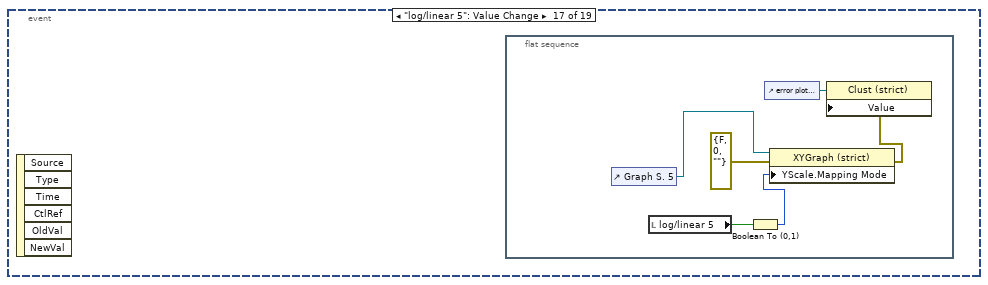
[diagram p18: hidden frame]
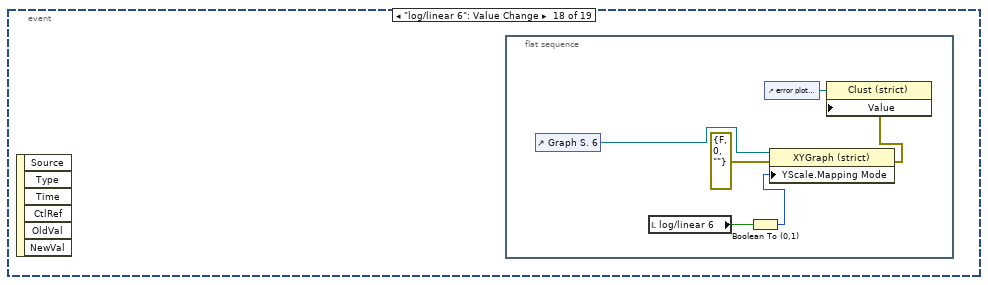
[diagram p19: hidden frame]
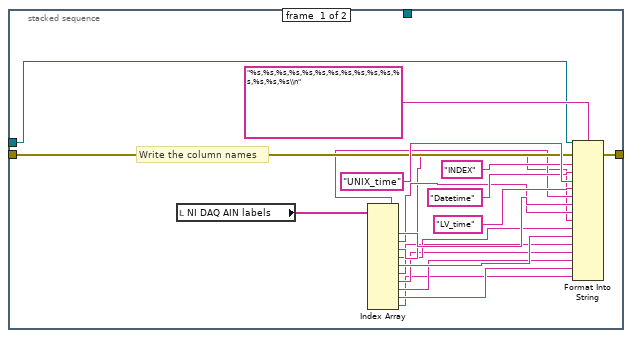
[diagram p20: hidden frame]
diagram:
  n1 = stacked-sequence {
    tunnel: [_ w144] -> w23
    tunnel: [_ w143] -> w22
    frame #0 {
      w46 = errorcluster {"status"=FALSE, "code"=0, "source"=""} ("error in")
      w41 = ".csv" ("string")
      w28 = T2."create" ("operation (0:open)")
      n2 = flat-sequence {
        frame #0 {
          w60 = i32[] [0, 1, 2, 3, 4, 5, 6, 7] ("idx in")
          # "CONSTANTS"
          "U idx" <- w60
          "D idx" <- w60
          "Q idx" <- i32[] [0, 1, 2, 3, 4, 5, 6, 7, 8, 9, 10] ("Q idx 2")
          "DAQ CH OUT" <- "O1" ("DAQ CH OUT 2")
          "DAQ CH 2" <- string[] ["Q1", "Q2", "Q3", "Q4", "Q5", "Q6", "Q7", "Q8", "Q9", "Q10", "Q11"] ("DAQ CH")
          "LSI-D CH 2" <- string[] ["D1", "D2", "D3", "D4", "D5", "D6", "D7", "D8"] ("LSI-D CH")
          "LSI-U CH 2" <- string[] ["U1", "U2", "U3", "U4", "U5", "U6", "U7", "U8"] ("LSI-U CH 3")
        }
      }
      n3 = Get Date/Time In Seconds() -> (seconds since 1Jan1904=w54:timestamp)
      n4 = Format Date/Time String(time format string (%c)="%Y%m%d_%H%M%S_", seconds (now)=w54) -> (date/time string=w32:string)  [unwired: 1 in]
      "date/time string" <- w32
      n5 = Concatenate Strings(w32, "CSV filename suffix", "_DAQ_RAW" ("string"), ".csv" ("string")) -> (w29:string)
      n6 = Concatenate Strings(w32, "CSV filename suffix", "_LSIU" ("string"), w41) -> (w51:string)
      n7 = Concatenate Strings(w32, "CSV filename suffix", "_LSID" ("string"), w41) -> (w40:string)
      n8 = Concatenate Strings(w32, "CSV filename suffix", "_DAQ" ("string"), w41) -> (w49:string)
      n9 = Build Path(base path="base path", name or relative path=w29) -> (appended path=w27:path)
      n10 = Build Path(base path="base path", name or relative path=w51) -> (appended path=w52:path)
      n11 = Build Path(base path="base path", name or relative path=w40) -> (appended path=w39:path)
      n12 = Build Path(base path="base path", name or relative path=w49) -> (appended path=w47:path)
      n13 = Open/Create/Replace File(file path (use dialog)=w52, error in=w46, operation (0:open)=w28) -> (refnum out=w45:refnum<file>)  [unwired: 3 in, 2 out]
      "ref LSI-U" <- w45
      n14 = Open/Create/Replace File(file path (use dialog)=w47, error in=w46, operation (0:open)=w28) -> (refnum out=w44:refnum<file>, error out=w38:errorcluster)  [unwired: 3 in, 1 out]
      "ref DAQ" <- w44
      n15 = Open/Create/Replace File(file path (use dialog)=w39, error in=w38, operation (0:open)=w28) -> (refnum out=w35:refnum<file>, error out=w26:errorcluster)  [unwired: 3 in, 1 out]
      "ref LSI-D" <- w35
      n16 = Open/Create/Replace File(file path (use dialog)=w27, error in=w26, operation (0:open)=w28) -> (refnum out=w24:refnum<file>, error out=w25:errorcluster)  [unwired: 3 in, 1 out]
      "ref RAW" <- w24
      n17 = flat-sequence {
        tunnel: w45 -> [w77]
        tunnel: w25 -> [w76]
        tunnel: [w72] -> w37
        tunnel: w37 -> [w82]
        tunnel: [w81] -> w36
        tunnel: w35 -> [w80]
        tunnel: w36 -> [w100]
        tunnel: w44 -> [w99]
        tunnel: [w98] -> w43
        tunnel: w24 -> [w97]
        frame #0 {
          # "Write the column names"
          n18 = local read "LSI-U CH labels"() -> (w70:string[])
          n19 = Array To Cluster(array=w70) -> (cluster=w69:T3)
          n20 = Unbundle(w69) -> ("LSI-U CH labels[0]"=w68:string, "LSI-U CH labels[1]"=w67:string, "LSI-U CH labels[2]"=w66:string, "LSI-U CH labels[3]"=w65:string, "LSI-U CH labels[4]"=w64:string, "LSI-U CH labels[5]"=w63:string, "LSI-U CH labels[6]"=w62:string, "LSI-U CH labels[7]"=w61:string)  [unwired: 1 out]
          n21 = Format Into String(format string="%s,%s,%s,%s,%s,%s,%s,%s,%s,%s,%s,%s\\n" ("time format string (%c)"), initial string=w77, error in=w76, "INDEX" ("input 1"), "Datetime" ("input 1"), "UNIX_time" ("input 1"), "LV_time" ("input 1"), w68, w67, w66, w65, w64, w63, w62, w61) -> (error out=w72:errorcluster)  [unwired: 1 out]
        }
        frame #1 {
          # "Write the column names"
          n22 = local read "LSI-D CH labels"() -> (w87:string[])
          n23 = Array To Cluster(array=w87) -> (cluster=w88:T4)
          n24 = Unbundle(w88) -> ("LSI-D CH labels[0]"=w89:string, "LSI-D CH labels[1]"=w90:string, "LSI-D CH labels[2]"=w91:string, "LSI-D CH labels[3]"=w92:string, "LSI-D CH labels[4]"=w93:string, "LSI-D CH labels[5]"=w94:string, "LSI-D CH labels[6]"=w95:string, "LSI-D CH labels[7]"=w96:string)  [unwired: 1 out]
          n25 = Format Into String(format string="%s,%s,%s,%s,%s,%s,%s,%s,%s,%s,%s,%s\\n" ("time format string (%c)"), initial string=w80, error in=w82, "INDEX" ("input 1"), "Datetime" ("input 1"), "UNIX_time" ("input 1"), "LV_time" ("input 1"), w89, w90, w91, w92, w93, w94, w95, w96) -> (error out=w81:errorcluster)  [unwired: 1 out]
        }
        frame #2 {
          n26 = stacked-sequence {
            tunnel: w100 -> [w116 w135]
            tunnel: w99 -> [w115 _]
            tunnel: [w114 _] -> w98
            tunnel: w97 -> [_ w121]
            frame #0 {
              # "Write the column names"
              n27 = local read "NI DAQ AIN labels"() -> (w112:string[])
              n28 = Index Array(array=w112) -> (element #1=w111:string, element #2=w110:string, element #3=w109:string, element #4=w108:string, element #5=w106:string, element #6=w107:string, element #7=w105:string, element #8=w104:string, element #9=w103:string, element #10=w102:string, element #11=w101:string)  [unwired: 11 in]
              n29 = Format Into String(format string="%s,%s,%s,%s,%s,%s,%s,%s,%s,%s,%s,%s,%s,%s,%s\\n" ("time format string (%c)"), initial string=w115, error in=w116, "INDEX" ("input 1"), "Datetime" ("input 1"), "UNIX_time" ("input 1"), "LV_time" ("input 1"), w111, w110, w109, w108, w106, w107, w105, w104, w103, w102, w101) -> (error out=w114:errorcluster)  [unwired: 1 out]
            }
            frame #1 {
              # "Write the column names"
              n30 = local read "NI DAQ AIN labels"() -> (w133:string[])
              n31 = Index Array(array=w133) -> (element #1=w132:string, element #2=w131:string, element #3=w130:string, element #4=w129:string, element #5=w127:string, element #6=w128:string, element #7=w126:string, element #8=w125:string, element #9=w124:string, element #10=w123:string, element #11=w122:string)  [unwired: 11 in]
              n32 = Format Into String(format string="%s,%s,%s,%s,%s,%s,%s,%s,%s,%s,%s,%s,%s,%s,%s\\n" ("time format string (%c)"), initial string=w121, error in=w135, "INDEX" ("input 1"), "Datetime" ("input 1"), "UNIX_time" ("input 1"), "LV_time" ("input 1"), w132, w131, w130, w129, w127, w128, w126, w125, w124, w123, w122) -> ()  [unwired: 2 out]
            }
          }
        }
      }
      "error out\n(file creation)" <- w43
    }
    frame #1 {
      # "DAQ config"
      n33 = feedback #1() -> (w140:errorcluster)  [unwired: 1 in]
      n34 = stacked-sequence {
        tunnel: [w145 _] -> w141
        tunnel: [w146 _] -> w144
        tunnel: [_ w174] -> w143
        tunnel: [_ w173] -> w142
        tunnel: w140 -> [_ w166]
        frame #0 {
          # "read task"
          n35 = local read "date/time string"() -> (w156:string)
          n36 = Concatenate Strings(w156, "AI" ("new task name")) -> (w154:string)
          n37 = call <vilib>:"DAQmx Create Task.vi"("new task name"=w154, "error in"=errorcluster {"status"=FALSE, "code"=0, "source"=""}) -> ("task out"=w152:refnum<k21>, "error out"=w153:errorcluster)  [unwired: 12 in]
          n38 = for {
            shift-right: [w165] -> w147
            shift-left: w153 -> [w164]
            shift-right: [w163] -> w148
            shift-left: w152 -> [w162]
            tunnel: "DAQ analog channels" -> [w161] mode=indexing
            tunnel: "V_min(in)" -> [w160] mode=indexing
            tunnel: "V_max(in)" -> [w159] mode=indexing
            w158 = 10106 items=["Default"=-1, "RSE"=10083, "NRSE"=10078, "Differential"=10106, "Pseudodifferential"=12529] ("input terminal configuration")
            n39 = call-poly <vilib>:"DAQmx Create Virtual Channel.vi"("task in"=w162, "maximum value"=w159, "minimum value"=w160, "input terminal configuration"=w158, "physical channels"=w161, "error in"=w164) -> ("task out"=w163:refnum<k21>, "error out"=w165:errorcluster)  [unwired: 8 in]
          }
          n40 = call <vilib>:"DAQmx Start Task.vi"("task/channels in"=w148, "error in"=w147) -> ("task out"=w146:refnum<k21>, "error out"=w145:errorcluster)  [unwired: 12 in]
        }
        frame #1 {
          # "write task"
          n41 = local read "date/time string"() -> (w169:string)
          n42 = Concatenate Strings(w169, "AO" ("new task name")) -> (w167:string)
          n43 = call <vilib>:"DAQmx Create Task.vi"("new task name"=w167, "error in"=w166) -> ("task out"=w171:refnum<k21>, "error out"=w170:errorcluster)  [unwired: 12 in]
          n44 = case shown="True" "DAQ OUT ON?" {
            tunnel: [w176 w183] -> w174
            tunnel: [w175 w182] -> w173
            tunnel: w171 -> [w176 w181]
            tunnel: w170 -> [w175 w180]
            frame False {
            }
            frame True {
              w185 = -1 items=["Default"=-1, "RSE"=10083, "Differential"=10106, "Pseudodifferential"=12529] ("output terminal configuration")
              w184 = 10348 items=["Volts"=10348, "From Custom Scale"=10065] ("units")
              n45 = call-poly <vilib>:"DAQmx Create Virtual Channel.vi"("task in"=w181, "maximum value"="V_max(out)", "minimum value"="V_min(out)", "output terminal configuration"=w185, "physical channels"="DAQ  OUT", "units"=w184, "error in"=w180) -> ("task out"=w187:refnum<k21>, "error out"=w186:errorcluster)  [unwired: 7 in]
              n46 = call <vilib>:"DAQmx Start Task.vi"("task/channels in"=w187, "error in"=w186) -> ("task out"=w183:refnum<k21>, "error out"=w182:errorcluster)  [unwired: 12 in]
            }
          }
        }
      }
      "error out\n(DAQ config)" <- w142
      n47 = feedback-in #1(w141) -> ()
    }
  }
  n48 = while {
    stop <- w188 stop-if-true
    n49 = event shown="[18] \"stop\": Value Change" {
      selector: _ -> [_ _ _ _ _ _ _ _ _ _ _ _ _ _ _ _ _ _ _]
      dyn-events: _ -> [_ _ _ _ _ _ _ _ _ _ _ _ _ _ _ _ _ _ _]
      timeout: _ -> [_ _ _ _ _ _ _ _ _ _ _ _ _ _ _ _ _ _ _]
      tunnel: [_ _ _ _ _ _ _ _ _ _ _ _ _ _ _ _ _ _ TRUE] -> w188
      event "GraphU1 SEL": Value Change {
        n50 = event-data() -> ()  [unwired: 1 in, 6 out]
        n51 = flat-sequence {
          tunnel: [w194] -> w191
          tunnel: [w192] -> w190
          tunnel: w191 -> [w203]
          tunnel: w190 -> [w200]
          frame #0 {
            n52 = control-ref of="LSI-U Grpah 1"() -> (w192:refnum<vi>)
            n53 = for {
              N: 8 -> [_]
              tunnel: [w196] -> w194 mode=indexing
              tunnel: w192 -> [w195]
              i -> [w198]
              n54 = property class="XYGraph (strict)"(reference=w195, error in=errorcluster {"status"=FALSE, "code"=0, "source"=""} ("error in (no error)"), "Active Plot"=w198, "Plot.Visible?"=FALSE ("Plot.Visible")) -> (error out=w196:errorcluster)  [unwired: 1 out]
            }
          }
          frame #1 {
            n55 = local read "GraphU1 SEL"() -> (w204:i32[])
            n56 = Array Size(array=w204) -> (size(s)=w205:i32)
            n57 = for {
              N: w205 -> [_]
              tunnel: w204 -> [w209] mode=indexing
              tunnel: w203 -> [w210] mode=indexing
              tunnel: [w207] -> w201 mode=indexing
              tunnel: w200 -> [w206]
              n58 = property class="XYGraph (strict)"(reference=w206, error in=w210, "Active Plot"=w209, "Plot.Visible?"=TRUE ("Plot.Visible")) -> (error out=w207:errorcluster)  [unwired: 1 out]
            }
            n59 = control-ref of="errors plot cosmetic 1"() -> (w202:refnum<vi>)
            n60 = property class="Arr (strict)"(reference=w202, "Value"=w201) -> ()  [unwired: 1 in, 2 out]
          }
        }
      }
      event "GraphU2 SEL": Value Change {
        n61 = event-data() -> ()  [unwired: 1 in, 6 out]
        n62 = flat-sequence {
          tunnel: [w215] -> w212
          tunnel: [w213] -> w211
          tunnel: w212 -> [w224]
          tunnel: w211 -> [w221]
          frame #0 {
            n63 = control-ref of="LSI-U Grpah 2"() -> (w213:refnum<vi>)
            n64 = for {
              N: 8 -> [_]
              tunnel: [w217] -> w215 mode=indexing
              tunnel: w213 -> [w216]
              i -> [w219]
              n65 = property class="XYGraph (strict)"(reference=w216, error in=errorcluster {"status"=FALSE, "code"=0, "source"=""} ("error in (no error)"), "Active Plot"=w219, "Plot.Visible?"=FALSE ("Plot.Visible")) -> (error out=w217:errorcluster)  [unwired: 1 out]
            }
          }
          frame #1 {
            n66 = local read "GraphU2 SEL"() -> (w225:i32[])
            n67 = Array Size(array=w225) -> (size(s)=w226:i32)
            n68 = for {
              N: w226 -> [_]
              tunnel: w225 -> [w230] mode=indexing
              tunnel: w224 -> [w231] mode=indexing
              tunnel: [w228] -> w222 mode=indexing
              tunnel: w221 -> [w227]
              n69 = property class="XYGraph (strict)"(reference=w227, error in=w231, "Active Plot"=w230, "Plot.Visible?"=TRUE ("Plot.Visible")) -> (error out=w228:errorcluster)  [unwired: 1 out]
            }
            n70 = control-ref of="errors plot cosmetic 1"() -> (w223:refnum<vi>)
            n71 = property class="Arr (strict)"(reference=w223, "Value"=w222) -> ()  [unwired: 1 in, 2 out]
          }
        }
      }
      event "GraphU3 SEL": Value Change {
        n72 = event-data() -> ()  [unwired: 1 in, 6 out]
        n73 = flat-sequence {
          tunnel: [w237] -> w233
          tunnel: [w234] -> w232
          tunnel: w233 -> [w246]
          tunnel: w232 -> [w243]
          frame #0 {
            n74 = control-ref of="LSI-U Grpah 3"() -> (w235:refnum<vi>)
            n75 = for {
              N: 8 -> [_]
              tunnel: [w239] -> w237 mode=indexing
              tunnel: w235 -> [w238]
              tunnel: [w238] -> w234 mode=indexing
              i -> [w241]
              n76 = property class="XYGraph (strict)"(reference=w238, error in=errorcluster {"status"=FALSE, "code"=0, "source"=""} ("error in (no error)"), "Active Plot"=w241, "Plot.Visible?"=FALSE ("Plot.Visible")) -> (error out=w239:errorcluster)  [unwired: 1 out]
            }
          }
          frame #1 {
            n77 = local read "GraphU3 SEL"() -> (w247:i32[])
            n78 = Array Size(array=w247) -> (size(s)=w248:i32)
            n79 = for {
              N: w248 -> [_]
              tunnel: w247 -> [w252] mode=indexing
              tunnel: w246 -> [w253] mode=indexing
              tunnel: [w250] -> w244 mode=indexing
              tunnel: w243 -> [w249] mode=indexing
              n80 = property class="XYGraph (strict)"(reference=w249, error in=w253, "Active Plot"=w252, "Plot.Visible?"=TRUE ("Plot.Visible")) -> (error out=w250:errorcluster)  [unwired: 1 out]
            }
            n81 = control-ref of="errors plot cosmetic 1"() -> (w245:refnum<vi>)
            n82 = property class="Arr (strict)"(reference=w245, "Value"=w244) -> ()  [unwired: 1 in, 2 out]
          }
        }
      }
      event "GraphD1 SEL": Value Change {
        n83 = event-data() -> ()  [unwired: 1 in, 6 out]
        n84 = flat-sequence {
          tunnel: [w258] -> w255
          tunnel: [w256] -> w254
          tunnel: w255 -> [w267]
          tunnel: w254 -> [w264]
          frame #0 {
            n85 = control-ref of="LSI-D Grpah 1"() -> (w256:refnum<vi>)
            n86 = for {
              N: 8 -> [_]
              tunnel: [w260] -> w258 mode=indexing
              tunnel: w256 -> [w259]
              i -> [w262]
              n87 = property class="XYGraph (strict)"(reference=w259, error in=errorcluster {"status"=FALSE, "code"=0, "source"=""} ("error in (no error)"), "Active Plot"=w262, "Plot.Visible?"=FALSE ("Plot.Visible")) -> (error out=w260:errorcluster)  [unwired: 1 out]
            }
          }
          frame #1 {
            n88 = local read "GraphD1 SEL"() -> (w268:i32[])
            n89 = Array Size(array=w268) -> (size(s)=w269:i32)
            n90 = for {
              N: w269 -> [_]
              tunnel: w268 -> [w273] mode=indexing
              tunnel: w267 -> [w274] mode=indexing
              tunnel: [w271] -> w265 mode=indexing
              tunnel: w264 -> [w270]
              n91 = property class="XYGraph (strict)"(reference=w270, error in=w274, "Active Plot"=w273, "Plot.Visible?"=TRUE ("Plot.Visible")) -> (error out=w271:errorcluster)  [unwired: 1 out]
            }
            n92 = control-ref of="errors plot cosmetic 1"() -> (w266:refnum<vi>)
            n93 = property class="Arr (strict)"(reference=w266, "Value"=w265) -> ()  [unwired: 1 in, 2 out]
          }
        }
      }
      event "GraphD2 SEL": Value Change {
        n94 = event-data() -> ()  [unwired: 1 in, 6 out]
        n95 = flat-sequence {
          tunnel: [w279] -> w276
          tunnel: [w277] -> w275
          tunnel: w276 -> [w288]
          tunnel: w275 -> [w285]
          frame #0 {
            n96 = control-ref of="LSI-D Grpah 2"() -> (w277:refnum<vi>)
            n97 = for {
              N: 8 -> [_]
              tunnel: [w281] -> w279 mode=indexing
              tunnel: w277 -> [w280]
              i -> [w283]
              n98 = property class="XYGraph (strict)"(reference=w280, error in=errorcluster {"status"=FALSE, "code"=0, "source"=""} ("error in (no error)"), "Active Plot"=w283, "Plot.Visible?"=FALSE ("Plot.Visible")) -> (error out=w281:errorcluster)  [unwired: 1 out]
            }
          }
          frame #1 {
            n99 = local read "GraphD2 SEL"() -> (w289:i32[])
            n100 = Array Size(array=w289) -> (size(s)=w290:i32)
            n101 = for {
              N: w290 -> [_]
              tunnel: w289 -> [w294] mode=indexing
              tunnel: w288 -> [w295] mode=indexing
              tunnel: [w292] -> w286 mode=indexing
              tunnel: w285 -> [w291]
              n102 = property class="XYGraph (strict)"(reference=w291, error in=w295, "Active Plot"=w294, "Plot.Visible?"=TRUE ("Plot.Visible")) -> (error out=w292:errorcluster)  [unwired: 1 out]
            }
            n103 = control-ref of="errors plot cosmetic 1"() -> (w287:refnum<vi>)
            n104 = property class="Arr (strict)"(reference=w287, "Value"=w286) -> ()  [unwired: 1 in, 2 out]
          }
        }
      }
      event "GraphD3 SEL": Value Change {
        n105 = event-data() -> ()  [unwired: 1 in, 6 out]
        n106 = flat-sequence {
          tunnel: [w300] -> w297
          tunnel: [w298] -> w296
          tunnel: w297 -> [w309]
          tunnel: w296 -> [w306]
          frame #0 {
            n107 = control-ref of="LSI-D Grpah 3"() -> (w298:refnum<vi>)
            n108 = for {
              N: 8 -> [_]
              tunnel: [w302] -> w300 mode=indexing
              tunnel: w298 -> [w301]
              i -> [w304]
              n109 = property class="XYGraph (strict)"(reference=w301, error in=errorcluster {"status"=FALSE, "code"=0, "source"=""} ("error in (no error)"), "Active Plot"=w304, "Plot.Visible?"=FALSE ("Plot.Visible")) -> (error out=w302:errorcluster)  [unwired: 1 out]
            }
          }
          frame #1 {
            n110 = local read "GraphD3 SEL"() -> (w310:i32[])
            n111 = Array Size(array=w310) -> (size(s)=w311:i32)
            n112 = for {
              N: w311 -> [_]
              tunnel: w310 -> [w315] mode=indexing
              tunnel: w309 -> [w316] mode=indexing
              tunnel: [w313] -> w307 mode=indexing
              tunnel: w306 -> [w312]
              n113 = property class="XYGraph (strict)"(reference=w312, error in=w316, "Active Plot"=w315, "Plot.Visible?"=TRUE ("Plot.Visible")) -> (error out=w313:errorcluster)  [unwired: 1 out]
            }
            n114 = control-ref of="errors plot cosmetic 1"() -> (w308:refnum<vi>)
            n115 = property class="Arr (strict)"(reference=w308, "Value"=w307) -> ()  [unwired: 1 in, 2 out]
          }
        }
      }
      event "S.1 SEL": Value Change {
        n116 = event-data() -> ()  [unwired: 1 in, 6 out]
        n117 = flat-sequence {
          tunnel: [w321] -> w317
          tunnel: w317 -> [w330]
          frame #0 {
            n118 = local read "DAQ CONV. OUT"() -> (w319:dbl[])
            n119 = control-ref of="Graph S. 1"() -> (w320:refnum<vi>)
            n120 = Array Size(array=w319) -> (size(s)=w318:i32)
            n121 = for {
              N: w318 -> [_]
              tunnel: [w323] -> w321 mode=indexing
              tunnel: w320 -> [w322]
              i -> [w325]
              n122 = property class="XYGraph (strict)"(reference=w322, error in=errorcluster {"status"=FALSE, "code"=0, "source"=""} ("error in (no error)"), "Active Plot"=w325, "Plot.Visible?"=FALSE ("Plot.Visible")) -> (error out=w323:errorcluster)  [unwired: 1 out]
            }
          }
          frame #1 {
            n123 = local read "S.1 SEL"() -> (w331:i32[])
            n124 = control-ref of="Graph S. 1"() -> (w327:refnum<vi>)
            n125 = Array Size(array=w331) -> (size(s)=w332:i32)
            n126 = for {
              N: w332 -> [_]
              tunnel: w331 -> [w336] mode=indexing
              tunnel: w330 -> [w337] mode=indexing
              tunnel: [w334] -> w328 mode=indexing
              tunnel: w327 -> [w333]
              n127 = property class="XYGraph (strict)"(reference=w333, error in=w337, "Active Plot"=w336, "Plot.Visible?"=TRUE ("Plot.Visible")) -> (error out=w334:errorcluster)  [unwired: 1 out]
            }
            n128 = control-ref of="errors plot cosmetic 1"() -> (w329:refnum<vi>)
            n129 = property class="Arr (strict)"(reference=w329, "Value"=w328) -> ()  [unwired: 1 in, 2 out]
          }
        }
      }
      event "S.2 SEL": Value Change {
        n130 = event-data() -> ()  [unwired: 1 in, 6 out]
        n131 = flat-sequence {
          tunnel: [w342] -> w338
          tunnel: w338 -> [w351]
          frame #0 {
            n132 = local read "DAQ CONV. OUT"() -> (w341:dbl[])
            n133 = control-ref of="Graph S. 2"() -> (w339:refnum<vi>)
            n134 = Array Size(array=w341) -> (size(s)=w340:i32)
            n135 = for {
              N: w340 -> [_]
              tunnel: [w344] -> w342 mode=indexing
              tunnel: w339 -> [w343]
              i -> [w346]
              n136 = property class="XYGraph (strict)"(reference=w343, error in=errorcluster {"status"=FALSE, "code"=0, "source"=""} ("error in (no error)"), "Active Plot"=w346, "Plot.Visible?"=FALSE ("Plot.Visible")) -> (error out=w344:errorcluster)  [unwired: 1 out]
            }
          }
          frame #1 {
            n137 = local read "S.2 SEL"() -> (w352:i32[])
            n138 = control-ref of="Graph S. 2"() -> (w348:refnum<vi>)
            n139 = Array Size(array=w352) -> (size(s)=w353:i32)
            n140 = for {
              N: w353 -> [_]
              tunnel: w352 -> [w357] mode=indexing
              tunnel: w351 -> [w358] mode=indexing
              tunnel: [w355] -> w349 mode=indexing
              tunnel: w348 -> [w354]
              n141 = property class="XYGraph (strict)"(reference=w354, error in=w358, "Active Plot"=w357, "Plot.Visible?"=TRUE ("Plot.Visible")) -> (error out=w355:errorcluster)  [unwired: 1 out]
            }
            n142 = control-ref of="errors plot cosmetic 1"() -> (w350:refnum<vi>)
            n143 = property class="Arr (strict)"(reference=w350, "Value"=w349) -> ()  [unwired: 1 in, 2 out]
          }
        }
      }
      event "S.3 SEL": Value Change {
        n144 = event-data() -> ()  [unwired: 1 in, 6 out]
        n145 = flat-sequence {
          tunnel: [w363] -> w359
          tunnel: w359 -> [w372]
          frame #0 {
            n146 = local read "DAQ CONV. OUT"() -> (w362:dbl[])
            n147 = control-ref of="Graph S. 3"() -> (w360:refnum<vi>)
            n148 = Array Size(array=w362) -> (size(s)=w361:i32)
            n149 = for {
              N: w361 -> [_]
              tunnel: [w365] -> w363 mode=indexing
              tunnel: w360 -> [w364]
              i -> [w367]
              n150 = property class="XYGraph (strict)"(reference=w364, error in=errorcluster {"status"=FALSE, "code"=0, "source"=""} ("error in (no error)"), "Active Plot"=w367, "Plot.Visible?"=FALSE ("Plot.Visible")) -> (error out=w365:errorcluster)  [unwired: 1 out]
            }
          }
          frame #1 {
            n151 = local read "S.3 SEL"() -> (w373:i32[])
            n152 = control-ref of="Graph S. 3"() -> (w369:refnum<vi>)
            n153 = Array Size(array=w373) -> (size(s)=w374:i32)
            n154 = for {
              N: w374 -> [_]
              tunnel: w373 -> [w378] mode=indexing
              tunnel: w372 -> [w379] mode=indexing
              tunnel: [w376] -> w370 mode=indexing
              tunnel: w369 -> [w375]
              n155 = property class="XYGraph (strict)"(reference=w375, error in=w379, "Active Plot"=w378, "Plot.Visible?"=TRUE ("Plot.Visible")) -> (error out=w376:errorcluster)  [unwired: 1 out]
            }
            n156 = control-ref of="errors plot cosmetic 1"() -> (w371:refnum<vi>)
            n157 = property class="Arr (strict)"(reference=w371, "Value"=w370) -> ()  [unwired: 1 in, 2 out]
          }
        }
      }
      event "S.4 SEL": Value Change {
        n158 = event-data() -> ()  [unwired: 1 in, 6 out]
        n159 = flat-sequence {
          tunnel: [w384] -> w380
          tunnel: w380 -> [w393]
          frame #0 {
            n160 = local read "DAQ CONV. OUT"() -> (w383:dbl[])
            n161 = control-ref of="Graph S. 4"() -> (w381:refnum<vi>)
            n162 = Array Size(array=w383) -> (size(s)=w382:i32)
            n163 = for {
              N: w382 -> [_]
              tunnel: [w386] -> w384 mode=indexing
              tunnel: w381 -> [w385]
              i -> [w388]
              n164 = property class="XYGraph (strict)"(reference=w385, error in=errorcluster {"status"=FALSE, "code"=0, "source"=""} ("error in (no error)"), "Active Plot"=w388, "Plot.Visible?"=FALSE ("Plot.Visible")) -> (error out=w386:errorcluster)  [unwired: 1 out]
            }
          }
          frame #1 {
            n165 = local read "S.4 SEL"() -> (w394:i32[])
            n166 = control-ref of="Graph S. 4"() -> (w390:refnum<vi>)
            n167 = Array Size(array=w394) -> (size(s)=w395:i32)
            n168 = for {
              N: w395 -> [_]
              tunnel: w394 -> [w399] mode=indexing
              tunnel: w393 -> [w400] mode=indexing
              tunnel: [w397] -> w391 mode=indexing
              tunnel: w390 -> [w396]
              n169 = property class="XYGraph (strict)"(reference=w396, error in=w400, "Active Plot"=w399, "Plot.Visible?"=TRUE ("Plot.Visible")) -> (error out=w397:errorcluster)  [unwired: 1 out]
            }
            n170 = control-ref of="errors plot cosmetic 1"() -> (w392:refnum<vi>)
            n171 = property class="Arr (strict)"(reference=w392, "Value"=w391) -> ()  [unwired: 1 in, 2 out]
          }
        }
      }
      event "S.5 SEL": Value Change {
        n172 = event-data() -> ()  [unwired: 1 in, 6 out]
        n173 = flat-sequence {
          tunnel: [w405] -> w401
          tunnel: w401 -> [w414]
          frame #0 {
            n174 = local read "DAQ CONV. OUT"() -> (w404:dbl[])
            n175 = control-ref of="Graph S. 5"() -> (w402:refnum<vi>)
            n176 = Array Size(array=w404) -> (size(s)=w403:i32)
            n177 = for {
              N: w403 -> [_]
              tunnel: [w407] -> w405 mode=indexing
              tunnel: w402 -> [w406]
              i -> [w409]
              n178 = property class="XYGraph (strict)"(reference=w406, error in=errorcluster {"status"=FALSE, "code"=0, "source"=""} ("error in (no error)"), "Active Plot"=w409, "Plot.Visible?"=FALSE ("Plot.Visible")) -> (error out=w407:errorcluster)  [unwired: 1 out]
            }
          }
          frame #1 {
            n179 = local read "S.5 SEL"() -> (w415:i32[])
            n180 = control-ref of="Graph S. 5"() -> (w411:refnum<vi>)
            n181 = Array Size(array=w415) -> (size(s)=w416:i32)
            n182 = for {
              N: w416 -> [_]
              tunnel: w415 -> [w420] mode=indexing
              tunnel: w414 -> [w421] mode=indexing
              tunnel: [w418] -> w412 mode=indexing
              tunnel: w411 -> [w417]
              n183 = property class="XYGraph (strict)"(reference=w417, error in=w421, "Active Plot"=w420, "Plot.Visible?"=TRUE ("Plot.Visible")) -> (error out=w418:errorcluster)  [unwired: 1 out]
            }
            n184 = control-ref of="errors plot cosmetic 1"() -> (w413:refnum<vi>)
            n185 = property class="Arr (strict)"(reference=w413, "Value"=w412) -> ()  [unwired: 1 in, 2 out]
          }
        }
      }
      event "S.6 SEL": Value Change {
        n186 = event-data() -> ()  [unwired: 1 in, 6 out]
        n187 = flat-sequence {
          tunnel: [w426] -> w422
          tunnel: w422 -> [w435]
          frame #0 {
            n188 = local read "DAQ CONV. OUT"() -> (w425:dbl[])
            n189 = control-ref of="Graph S. 6"() -> (w423:refnum<vi>)
            n190 = Array Size(array=w425) -> (size(s)=w424:i32)
            n191 = for {
              N: w424 -> [_]
              tunnel: [w428] -> w426 mode=indexing
              tunnel: w423 -> [w427]
              i -> [w430]
              n192 = property class="XYGraph (strict)"(reference=w427, error in=errorcluster {"status"=FALSE, "code"=0, "source"=""} ("error in (no error)"), "Active Plot"=w430, "Plot.Visible?"=FALSE ("Plot.Visible")) -> (error out=w428:errorcluster)  [unwired: 1 out]
            }
          }
          frame #1 {
            n193 = local read "S.6 SEL"() -> (w436:i32[])
            n194 = control-ref of="Graph S. 6"() -> (w432:refnum<vi>)
            n195 = Array Size(array=w436) -> (size(s)=w437:i32)
            n196 = for {
              N: w437 -> [_]
              tunnel: w436 -> [w441] mode=indexing
              tunnel: w435 -> [w442] mode=indexing
              tunnel: [w439] -> w433 mode=indexing
              tunnel: w432 -> [w438]
              n197 = property class="XYGraph (strict)"(reference=w438, error in=w442, "Active Plot"=w441, "Plot.Visible?"=TRUE ("Plot.Visible")) -> (error out=w439:errorcluster)  [unwired: 1 out]
            }
            n198 = control-ref of="errors plot cosmetic 1"() -> (w434:refnum<vi>)
            n199 = property class="Arr (strict)"(reference=w434, "Value"=w433) -> ()  [unwired: 1 in, 2 out]
          }
        }
      }
      event "log/linear 1": Value Change {
        n200 = event-data() -> ()  [unwired: 1 in, 6 out]
        n201 = flat-sequence {
          frame #0 {
            n202 = control-ref of="Graph S. 1"() -> (w447:refnum<vi>)
            n203 = local read "log/linear 1"() -> (w446:bool)
            n204 = Boolean To (0,1)(Boolean=w446) -> (0, 1=w445:i16)
            n205 = control-ref of="error plot cosmetic 2"() -> (w444:refnum<vi>)
            n206 = property class="XYGraph (strict)"(reference=w447, error in=errorcluster {"status"=FALSE, "code"=0, "source"=""} ("error in (no error)"), "YScale.Mapping Mode"=w445) -> (error out=w443:errorcluster)  [unwired: 1 out]
            n207 = property class="Clust (strict)"(reference=w444, "Value"=w443) -> ()  [unwired: 1 in, 2 out]
          }
        }
      }
      event "log/linear 2": Value Change {
        n208 = event-data() -> ()  [unwired: 1 in, 6 out]
        n209 = flat-sequence {
          frame #0 {
            n210 = control-ref of="Graph S. 2"() -> (w449:refnum<vi>)
            n211 = local read "log/linear 2"() -> (w453:bool)
            n212 = Boolean To (0,1)(Boolean=w453) -> (0, 1=w452:i16)
            n213 = control-ref of="error plot cosmetic 2"() -> (w451:refnum<vi>)
            n214 = property class="XYGraph (strict)"(reference=w449, error in=errorcluster {"status"=FALSE, "code"=0, "source"=""} ("error in (no error)"), "YScale.Mapping Mode"=w452) -> (error out=w450:errorcluster)  [unwired: 1 out]
            n215 = property class="Clust (strict)"(reference=w451, "Value"=w450) -> ()  [unwired: 1 in, 2 out]
          }
        }
      }
      event "log/linear 3": Value Change {
        n216 = event-data() -> ()  [unwired: 1 in, 6 out]
        n217 = flat-sequence {
          frame #0 {
            n218 = control-ref of="Graph S. 3"() -> (w455:refnum<vi>)
            n219 = local read "log/linear 3"() -> (w459:bool)
            n220 = Boolean To (0,1)(Boolean=w459) -> (0, 1=w458:i16)
            n221 = control-ref of="error plot cosmetic 2"() -> (w457:refnum<vi>)
            n222 = property class="XYGraph (strict)"(reference=w455, error in=errorcluster {"status"=FALSE, "code"=0, "source"=""} ("error in (no error)"), "YScale.Mapping Mode"=w458) -> (error out=w456:errorcluster)  [unwired: 1 out]
            n223 = property class="Clust (strict)"(reference=w457, "Value"=w456) -> ()  [unwired: 1 in, 2 out]
          }
        }
      }
      event "log/linear 4": Value Change {
        n224 = event-data() -> ()  [unwired: 1 in, 6 out]
        n225 = flat-sequence {
          frame #0 {
            n226 = control-ref of="Graph S. 4"() -> (w461:refnum<vi>)
            n227 = local read "log/linear 4"() -> (w465:bool)
            n228 = Boolean To (0,1)(Boolean=w465) -> (0, 1=w464:i16)
            n229 = control-ref of="error plot cosmetic 2"() -> (w463:refnum<vi>)
            n230 = property class="XYGraph (strict)"(reference=w461, error in=errorcluster {"status"=FALSE, "code"=0, "source"=""} ("error in (no error)"), "YScale.Mapping Mode"=w464) -> (error out=w462:errorcluster)  [unwired: 1 out]
            n231 = property class="Clust (strict)"(reference=w463, "Value"=w462) -> ()  [unwired: 1 in, 2 out]
          }
        }
      }
      event "log/linear 5": Value Change {
        n232 = event-data() -> ()  [unwired: 1 in, 6 out]
        n233 = flat-sequence {
          frame #0 {
            n234 = control-ref of="Graph S. 5"() -> (w467:refnum<vi>)
            n235 = local read "log/linear 5"() -> (w471:bool)
            n236 = Boolean To (0,1)(Boolean=w471) -> (0, 1=w470:i16)
            n237 = control-ref of="error plot cosmetic 2"() -> (w469:refnum<vi>)
            n238 = property class="XYGraph (strict)"(reference=w467, error in=errorcluster {"status"=FALSE, "code"=0, "source"=""} ("error in (no error)"), "YScale.Mapping Mode"=w470) -> (error out=w468:errorcluster)  [unwired: 1 out]
            n239 = property class="Clust (strict)"(reference=w469, "Value"=w468) -> ()  [unwired: 1 in, 2 out]
          }
        }
      }
      event "log/linear 6": Value Change {
        n240 = event-data() -> ()  [unwired: 1 in, 6 out]
        n241 = flat-sequence {
          frame #0 {
            n242 = control-ref of="Graph S. 6"() -> (w473:refnum<vi>)
            n243 = local read "log/linear 6"() -> (w477:bool)
            n244 = Boolean To (0,1)(Boolean=w477) -> (0, 1=w476:i16)
            n245 = control-ref of="error plot cosmetic 2"() -> (w475:refnum<vi>)
            n246 = property class="XYGraph (strict)"(reference=w473, error in=errorcluster {"status"=FALSE, "code"=0, "source"=""} ("error in (no error)"), "YScale.Mapping Mode"=w476) -> (error out=w474:errorcluster)  [unwired: 1 out]
            n247 = property class="Clust (strict)"(reference=w475, "Value"=w474) -> ()  [unwired: 1 in, 2 out]
          }
        }
      }
      event "stop": Value Change {
        n248 = event-data() -> ()  [unwired: 1 in, 6 out]
      }
    }
    n249 = flat-sequence {
      frame #0 {
      }
    }
    n250 = flat-sequence {
      frame #0 {
      }
    }
    n251 = flat-sequence {
      frame #0 {
      }
    }
    n252 = control-ref of="LSI-U Grpah 3"() -> ()  [unwired: 1 out]
    n253 = control-ref of="LSI-D Grpah 2"() -> ()  [unwired: 1 out]
    n254 = control-ref of="LSI-U Grpah 2"() -> ()  [unwired: 1 out]
    n255 = control-ref of="LSI-D Grpah 1"() -> ()  [unwired: 1 out]
    n256 = control-ref of="LSI-U Grpah 1"() -> ()  [unwired: 1 out]
    n257 = control-ref of="LSI-D Grpah 3"() -> ()  [unwired: 1 out]
    n258 = control-ref of="Graph S. 6"() -> ()  [unwired: 1 out]
    n259 = control-ref of="Graph S. 5"() -> ()  [unwired: 1 out]
    n260 = control-ref of="Graph S. 4"() -> ()  [unwired: 1 out]
    n261 = control-ref of="Graph S. 3"() -> ()  [unwired: 1 out]
    n262 = control-ref of="Graph S. 2"() -> ()  [unwired: 1 out]
    n263 = control-ref of="Graph S. 1"() -> ()  [unwired: 1 out]
    n264 = Wait (ms)(milliseconds to wait=u32 500) -> ()  [unwired: 1 out]
  }
  n265 = call "Initialize.vi"("VISA resource name"="VISA LSI218 DOWN", "error in (no error)"=errorcluster {"status"=FALSE, "code"=0, "source"=""}) -> ("VISA resource name out"=w6:refnum<visa-resource-name>, "error out"=w5:errorcluster)  [unwired: 12 in]
  n266 = call "Initialize.vi"("VISA resource name"="VISA LSI218 UP", "error in (no error)"=errorcluster {"status"=FALSE, "code"=0, "source"=""}) -> ("VISA resource name out"=w4:refnum<visa-resource-name>, "error out"=w3:errorcluster)  [unwired: 12 in]
  n267 = while {
    shift-right: [w495] -> _
    shift-left: dbl[] [] -> [w506]
    shift-right: [w498] -> _
    shift-left: dbl[][] [] -> [w499]
    tunnel: w23 -> [w502]
    tunnel: w22 -> [w501]
    shift-right: [w494] -> _
    shift-left: dbl[][] [] -> [w500]
    tunnel: [w490] -> w12
    tunnel: [w489] -> w11
    tunnel: [w488] -> w10
    tunnel: w6 -> [w487]
    tunnel: w5 -> [w486]
    tunnel: w4 -> [w485]
    tunnel: w3 -> [w484]
    shift-right: [w481] -> _
    shift-left: dbl[][] [] -> [w480]
    i -> [w503]
    stop <- "stop" stop-if-true
    n268 = local read "current time"() -> (w504:timestamp)
    n269 = Get Date/Time In Seconds() -> (seconds since 1Jan1904=→"current time":timestamp)
    n270 = To Double Precision Float(number=w504) -> (double precision float=w505:dbl)
    n271 = Multiply(x="Wait (s)", y=1000) -> (x*y=w491:i32)
    n272 = Wait (ms)(milliseconds to wait=w491) -> ()  [unwired: 1 out]
    n273 = Build Array (concatenate)(w506, w505) -> (w495:dbl[])
    n274 = flat-sequence {
      tunnel: w495 -> [w800]
      tunnel: w499 -> [w878]
      tunnel: [w867] -> w496
      tunnel: w487 -> [w874]
      tunnel: w486 -> [w873]
      tunnel: w485 -> [w872]
      tunnel: w484 -> [w871]
      tunnel: [w801] -> w482
      tunnel: w480 -> [w802]
      tunnel: [w890] -> w497
      tunnel: w496 -> [w890]
      tunnel: [w889] -> w483
      tunnel: w482 -> [w889]
      tunnel: [w915] -> w498
      tunnel: w497 -> [w915]
      tunnel: [w910] -> w481
      tunnel: w483 -> [w910]
      frame #0 {
        n275 = call "Data Sensor.vi"("VISA resource name"=w874, "error in (no error)"=w873) -> ("Input 1"=w839:dbl, "Input 2"=w838:dbl, "Input 3"=w837:dbl, "VISA resource name out"=w876:refnum<visa-resource-name>, "Input 4"=w836:dbl, "Input 5"=w835:dbl, "Input 6"=w834:dbl, "Input 8"=w832:dbl, "Input 7"=w833:dbl, "error out"=w875:errorcluster)  [unwired: 4 in]
        n276 = call "Data Sensor.vi"("VISA resource name"=w872, "error in (no error)"=w871) -> ("Input 1"=w888:dbl, "Input 2"=w887:dbl, "Input 3"=w886:dbl, "VISA resource name out"=w880:refnum<visa-resource-name>, "Input 4"=w870:dbl, "Input 5"=w885:dbl, "Input 6"=w884:dbl, "Input 8"=w882:dbl, "Input 7"=w883:dbl, "error out"=w881:errorcluster)  [unwired: 4 in]
        n277 = local read "LSI-U CH labels"() -> (→"LSI-U CH indic,":string[])
        n278 = local read "LSI-D CH labels"() -> (→"LSI-D CH indic.":string[])
        n279 = Build Array(w839, w838, w837, w836, w835, w834, w833, w832) -> (w803:dbl[])
        "LSI-D out" <- w803
        n280 = call "Close.vi"("VISA resource name"=w876, "error in (no error)"=w875) -> ("error out"=→"error out \n(LSID)":errorcluster)  [unwired: 13 in]
        n281 = Build Array(w888, w887, w886, w870, w885, w884, w883, w882) -> (w868:dbl[])
        "LSI-U out" <- w868
        n282 = call "Close.vi"("VISA resource name"=w880, "error in (no error)"=w881) -> ("error out"=→"error out \n(LSIU)":errorcluster)  [unwired: 13 in]
        n283 = Array Size(array=w868) -> ()  [unwired: 1 out]
        n284 = Build Array (concatenate)(w878, w868) -> (w867:dbl[][])
        n285 = Build Array (concatenate)(w802, w803) -> (w801:dbl[][])
        n286 = Index Array(array=w867, index (col) #1=0 ("disabled index (col)"), index (col) #2=1 ("index (col)"), index (col) #3=2 ("index (col)"), index (col) #4=3 ("index (col)"), index (col) #5=4 ("index (col)"), index (col) #6=5 ("index (col)"), index (col) #7=6 ("index (col)"), index (col) #8=7 ("index (col)"), index (col) #9=8 ("index (col)")) -> (element #1=w865:dbl[], element #2=w856:dbl[], element #3=w855:dbl[], element #4=w854:dbl[], element #5=w853:dbl[], element #6=w852:dbl[], element #7=w851:dbl[], element #8=w850:dbl[], element #9=w849:dbl[])  [unwired: 9 in]
        n287 = Index Array(array=w801, index (col) #1=0 ("disabled index (col)"), index (col) #2=1 ("index (col)"), index (col) #3=2 ("index (col)"), index (col) #4=3 ("index (col)"), index (col) #5=4 ("index (col)"), index (col) #6=5 ("index (col)"), index (col) #7=6 ("index (col)"), index (col) #8=7 ("index (col)"), index (col) #9=8 ("index (col)")) -> (element #1=w805:dbl[], element #2=w814:dbl[], element #3=w815:dbl[], element #4=w816:dbl[], element #5=w817:dbl[], element #6=w818:dbl[], element #7=w819:dbl[], element #8=w820:dbl[], element #9=w821:dbl[])  [unwired: 9 in]
        n288 = Bundle(w800, w865) -> (w848:cluster{dbl[], dbl[]})  [unwired: 1 in]
        n289 = Bundle(w800, w856) -> (w847:cluster{dbl[], dbl[]})  [unwired: 1 in]
        n290 = Bundle(w800, w855) -> (w846:cluster{dbl[], dbl[]})  [unwired: 1 in]
        n291 = Bundle(w800, w854) -> (w845:cluster{dbl[], dbl[]})  [unwired: 1 in]
        n292 = Bundle(w800, w853) -> (w844:cluster{dbl[], dbl[]})  [unwired: 1 in]
        n293 = Bundle(w800, w852) -> (w843:cluster{dbl[], dbl[]})  [unwired: 1 in]
        n294 = Bundle(w800, w851) -> (w842:cluster{dbl[], dbl[]})  [unwired: 1 in]
        n295 = Bundle(w800, w850) -> (w841:cluster{dbl[], dbl[]})  [unwired: 1 in]
        n296 = Bundle(w800, w849) -> (w840:cluster{dbl[], dbl[]})  [unwired: 1 in]
        n297 = Bundle(w800, w805) -> (w822:cluster{dbl[], dbl[]})  [unwired: 1 in]
        n298 = Bundle(w800, w814) -> (w823:cluster{dbl[], dbl[]})  [unwired: 1 in]
        n299 = Bundle(w800, w815) -> (w824:cluster{dbl[], dbl[]})  [unwired: 1 in]
        n300 = Bundle(w800, w816) -> (w825:cluster{dbl[], dbl[]})  [unwired: 1 in]
        n301 = Bundle(w800, w817) -> (w826:cluster{dbl[], dbl[]})  [unwired: 1 in]
        n302 = Bundle(w800, w818) -> (w827:cluster{dbl[], dbl[]})  [unwired: 1 in]
        n303 = Bundle(w800, w819) -> (w828:cluster{dbl[], dbl[]})  [unwired: 1 in]
        n304 = Bundle(w800, w820) -> (w829:cluster{dbl[], dbl[]})  [unwired: 1 in]
        n305 = Bundle(w800, w821) -> (w830:cluster{dbl[], dbl[]})  [unwired: 1 in]
        n306 = Build Array(w848, w847, w846, w845, w844, w843, w842, w841, w840) -> (w799:cluster{dbl[], dbl[]}[])
        n307 = Build Array(w822, w823, w824, w825, w826, w827, w828, w829, w830) -> (w795:cluster{dbl[], dbl[]}[])
        n308 = control-ref of="LSI-U Grpah 1"() -> (w784:refnum<vi>)
        n309 = property class="XYGraph (strict)"(reference=w784, error in=errorcluster {"status"=FALSE, "code"=0, "source"=""} ("error in (no error)"), "Value"=w799) -> (error out=w797:errorcluster)  [unwired: 1 out]
        n310 = control-ref of="LSI-D Grpah 1"() -> (w787:refnum<vi>)
        n311 = property class="XYGraph (strict)"(reference=w787, error in=errorcluster {"status"=FALSE, "code"=0, "source"=""} ("error in (no error)"), "Value"=w795) -> (error out=w793:errorcluster)  [unwired: 1 out]
        n312 = control-ref of="LSI-U Grpah 2"() -> (w783:refnum<vi>)
        n313 = property class="XYGraph (strict)"(reference=w783, error in=w797, "Value"=w799) -> (error out=w796:errorcluster)  [unwired: 1 out]
        n314 = control-ref of="LSI-D Grpah 2"() -> (w786:refnum<vi>)
        n315 = property class="XYGraph (strict)"(reference=w786, error in=w793, "Value"=w795) -> (error out=w792:errorcluster)  [unwired: 1 out]
        n316 = control-ref of="LSI-U Grpah 3"() -> (w782:refnum<vi>)
        n317 = control-ref of="LSI-D Grpah 3"() -> (w785:refnum<vi>)
        n318 = property class="XYGraph (strict)"(reference=w782, error in=w796, "Value"=w799) -> (error out=w788:errorcluster)  [unwired: 1 out]
        n319 = property class="XYGraph (strict)"(reference=w785, error in=w792, "Value"=w795) -> (error out=w790:errorcluster)  [unwired: 1 out]
        n320 = control-ref of="error plot content"() -> (w789:refnum<vi>)
        n321 = control-ref of="error plot content"() -> (w791:refnum<vi>)
        n322 = property class="Clust (strict)"(reference=w789, "Value"=w788) -> ()  [unwired: 1 in, 2 out]
        n323 = property class="Clust (strict)"(reference=w791, "Value"=w790) -> ()  [unwired: 1 in, 2 out]
      }
      frame #1 {
      }
      frame #2 {
        n324 = local read "LSI-D out"() -> (w891:dbl[])
        n325 = local read "LSI-U out"() -> (w926:dbl[])
        n326 = local read "current time"() -> (w906:timestamp)
        n327 = local read "current time"() -> (w914:timestamp)
        n328 = local read "error out\n(file creation)"() -> (w893:errorcluster)
        n329 = local read "error out\n(file creation)"() -> (w929:errorcluster)
        n330 = Array To Cluster(array=w891) -> (cluster=w896:T5)
        n331 = Array To Cluster(array=w926) -> (cluster=w925:T6)
        n332 = local read "ref LSI-D"() -> (w892:refnum<file>)
        n333 = local read "ref LSI-U"() -> (w930:refnum<file>)
        n334 = local read "Cycle #"() -> (w909:i32)
        n335 = local read "Cycle #"() -> (w911:i32)
        n336 = To Double Precision Float(number=w906) -> (double precision float=w894:dbl)
        n337 = To Double Precision Float(number=w914) -> (double precision float=w928:dbl)
        n338 = call "LV_UNIX.vi"("current time"=w906) -> ("date/time string"=w908:string, "UNIX time (s)"=w907:dbl)  [unwired: 9 in]
        n339 = call "LV_UNIX.vi"("current time"=w914) -> ("date/time string"=w912:string, "UNIX time (s)"=w913:dbl)  [unwired: 9 in]
        n340 = Unbundle(w896) -> ("LSI-D out[0]"=w897:dbl, "LSI-D out[1]"=w898:dbl, "LSI-D out[2]"=w899:dbl, "LSI-D out[3]"=w900:dbl, "LSI-D out[4]"=w901:dbl, "LSI-D out[5]"=w902:dbl, "LSI-D out[6]"=w903:dbl, "LSI-D out[7]"=w904:dbl)  [unwired: 1 out]
        n341 = Unbundle(w925) -> ("LSI-U out[0]"=w924:dbl, "LSI-U out[1]"=w923:dbl, "LSI-U out[2]"=w922:dbl, "LSI-U out[3]"=w921:dbl, "LSI-U out[4]"=w920:dbl, "LSI-U out[5]"=w919:dbl, "LSI-U out[6]"=w918:dbl, "LSI-U out[7]"=w917:dbl)  [unwired: 1 out]
        n342 = Format Into String(format string="%d,%s,%10.4f,%10.4f,%5.6f,%5.6f,%5.6f,%5.6f,%5.6f,%5.6f,%5.6f,%5.6f\\n", initial string=w892, error in=w893, w909, w908, w907, w894, w897, w898, w899, w900, w901, w902, w903, w904) -> (error out=→"error out \n(record LSID)":errorcluster)  [unwired: 1 out]
        n343 = Format Into String(format string="%d,%s,%10.4f,%10.4f,%5.6f,%5.6f,%5.6f,%5.6f,%5.6f,%5.6f,%5.6f,%5.6f\\n", initial string=w930, error in=w929, w911, w912, w913, w928, w924, w923, w922, w921, w920, w919, w918, w917) -> (error out=→"error out \n(record LSIU)":errorcluster)  [unwired: 1 out]
      }
    }
    n344 = stacked-sequence {
      tunnel: w502 -> [w614 _]
      tunnel: w501 -> [_ w772]
      tunnel: [_ w770] -> w489
      tunnel: w500 -> [w596 _]
      tunnel: [w566 _] -> w494
      tunnel: w495 -> [w531 _]
      tunnel: [w595 _] -> w490
      tunnel: [_ w768] -> w488
      frame #0 {
        n345 = local read "NI DAQ AIN labels"() -> (→"NI-DAQ CH indic.":string[])
        n346 = local read "error out\n(DAQ config)"() -> (w610:errorcluster)
        n347 = local read "DAQ sample #"() -> (w591:i32)
        n348 = call <vilib>:"DAQmx Read (Analog 2D DBL NChan NSamp).vi"("task/channels in"=w614, "number of samples per channel"=w591, "timeout"=100.0, "error in"=w610) -> ("task out"=w595:refnum<k21>, "data"=w540:dbl[][], "error out"=→"error out \n(DAQ IN)":errorcluster)  [unwired: 9 in]
        n349 = Index Array(array=w540, index (col)=0 ("disabled index (col)")) -> (element=→"RAW (V)":dbl[])  [unwired: 1 in]
        n350 = Array Size(array=w540) -> (size(s)=→"size(s)":i32[])
        n351 = Index Array(array=w540, index (row) #1=0 ("index (row)"), index (row) #2=1 ("index (row)"), index (row) #3=2 ("index (row)"), index (row) #4=3 ("index (row)"), index (row) #5=4 ("disabled index (col)"), index (row) #6=5 ("index (col)"), index (row) #7=6 ("disabled index (row)"), index (row) #8=7 ("disabled index (row)"), index (row) #9=8 ("disabled index (row)"), index (row) #10=9 ("index (row)"), index (row) #11=10 ("index (row)")) -> (element #1=w575:dbl[], element #2=w580:dbl[], element #3=w584:dbl[], element #4=w577:dbl[], element #5=w576:dbl[], element #6=w574:dbl[], element #7=w570:dbl[], element #8=w569:dbl[], element #9=w568:dbl[], element #10=w543:dbl[], element #11=w542:dbl[])  [unwired: 11 in]
        n352 = stacked-sequence {
          tunnel: [w682 _ _ _ _ _ _ _ _ _ _] -> w594
          tunnel: [_ w691 _ _ _ _ _ _ _ _ _] -> w592
          tunnel: w591 -> [w680 w687 w696 w705 w714 w723 w733 w741 w753 w761 w767]
          tunnel: [_ _ w698 _ _ _ _ _ _ _ _] -> w590
          tunnel: w580 -> [_ w688 _ _ _ _ _ _ _ _ _]
          tunnel: [_ _ _ w707 _ _ _ _ _ _ _] -> w587
          tunnel: [_ _ _ _ w716 _ _ _ _ _ _] -> w586
          tunnel: [_ _ _ _ _ w725 _ _ _ _ _] -> w585
          tunnel: w584 -> [_ _ w697 _ _ _ _ _ _ _ _]
          tunnel: [_ _ _ _ _ _ w732 _ _ _ _] -> w583
          tunnel: w577 -> [_ _ _ w706 _ _ _ _ _ _ _]
          tunnel: w576 -> [_ _ _ _ w715 _ _ _ _ _ _]
          tunnel: w575 -> [w678 _ _ _ _ _ _ _ _ _ _]
          tunnel: w574 -> [_ _ _ _ _ w724 _ _ _ _ _]
          tunnel: w570 -> [_ _ _ _ _ _ w734 _ _ _ _]
          tunnel: w569 -> [_ _ _ _ _ _ _ w743 _ _ _]
          tunnel: w568 -> [_ _ _ _ _ _ _ _ w754 _ _]
          tunnel: [_ _ _ _ _ _ _ w742 _ _ _] -> w567
          tunnel: w543 -> [_ _ _ _ _ _ _ _ _ w760 _]
          tunnel: w542 -> [_ _ _ _ _ _ _ _ _ _ w766]
          tunnel: [_ _ _ _ _ _ _ _ _ _ w765] -> w541
          tunnel: [_ _ _ _ _ _ _ _ w752 _ _] -> w530
          tunnel: [_ _ _ _ _ _ _ _ _ w759 _] -> w529
          tunnel: [_ _ _ _ _ _ _ _ _ _ w762] -> w510
          tunnel: [_ _ _ _ _ _ _ _ w750 _ _] -> w511
          tunnel: [_ _ _ _ _ _ _ _ _ w756 _] -> w514
          tunnel: [_ _ _ _ _ _ _ _ _ w756 _] -> w513
          frame #0 {
            # "0"
            # "P (4K)"
            n353 = Add Array Elements(numeric array=w678) -> (sum=w681:dbl)
            n354 = Divide(x=w681, y=w680) -> (x/y=w679:dbl)
            n355 = call "scaling_calculator.vi"("x1"=1.0, "y1"=0.0 ("x1"), "x"=w679, "x2"=3.0 ("x1"), "y2"=100000.0 ("x1")) -> ("y"=w682:dbl)  [unwired: 2 in]
          }
          frame #1 {
            # "1"
            # "LM"
            n356 = Add Array Elements(numeric array=w688) -> (sum=w690:dbl)
            n357 = Divide(x=w690, y=w687) -> (x/y=w689:dbl)
            n358 = call "scaling_calculator.vi"("x1"=0.0, "y1"=0.0 ("x1"), "x"=w689, "x2"=0.1 ("x1"), "y2"=100.0 ("x1")) -> ("y"=w691:dbl)  [unwired: 2 in]
          }
          frame #2 {
            # "2"
            # "Delta P He 3"
            n359 = Add Array Elements(numeric array=w697) -> (sum=w700:dbl)
            n360 = Divide(x=w700, y=w696) -> (x/y=w699:dbl)
            n361 = call "scaling_calculator.vi"("x1"=1.0, "y1"=0.0 ("x1"), "x"=w699, "x2"=5.0 ("x1"), "y2"=20000.0 ("x1")) -> ("y"=w698:dbl)  [unwired: 2 in]
          }
          frame #3 {
            # "3"
            # "Delta P He 4"
            n362 = Add Array Elements(numeric array=w706) -> (sum=w709:dbl)
            n363 = Divide(x=w709, y=w705) -> (x/y=w708:dbl)
            n364 = call "scaling_calculator.vi"("x1"=1.0, "y1"=0.0 ("x1"), "x"=w708, "x2"=5.0 ("x1"), "y2"=1000.0 ("x1")) -> ("y"=w707:dbl)  [unwired: 2 in]
          }
          frame #4 {
            # "4"
            # "FM He4"
            n365 = Add Array Elements(numeric array=w715) -> (sum=w718:dbl)
            n366 = Divide(x=w718, y=w714) -> (x/y=w717:dbl)
            n367 = call "scaling_calculator.vi"("x1"=0.0, "y1"=0.0 ("x1"), "x"=w717, "x2"=5.0 ("x1"), "y2"=500.0 ("x1")) -> ("y"=w716:dbl)  [unwired: 2 in]
          }
          frame #5 {
            # "5"
            # "FM He3"
            n368 = Add Array Elements(numeric array=w724) -> (sum=w727:dbl)
            n369 = Divide(x=w727, y=w723) -> (x/y=w726:dbl)
            n370 = call "scaling_calculator.vi"("x1"=0.0, "y1"=0.0 ("x1"), "x"=w726, "x2"=5.0 ("x1"), "y2"=200.0 ("x1")) -> ("y"=w725:dbl)  [unwired: 2 in]
          }
          frame #6 {
            # "LM1300"
            # "6"
            n371 = Add Array Elements(numeric array=w734) -> (sum=w740:dbl)
            n372 = Divide(x=w740, y=w733) -> (x/y=w739:dbl)
            n373 = call "scaling_calculator.vi"("x1"=0.0, "y1"=0.0 ("x1"), "x"=w739, "x2"=10.0 ("x1"), "y2"=100.0 ("x1")) -> ("y"=w732:dbl)  [unwired: 2 in]
          }
          frame #7 {
            # "7"
            # "AI16 P 4He IN"
            n374 = Add Array Elements(numeric array=w743) -> (sum=w749:dbl)
            n375 = Divide(x=w749, y=w741) -> (x/y=w744:dbl)
            n376 = call "scaling_calculator.vi"("x1"=1.0, "y1"=0.0 ("x1"), "x"=w744, "x2"=5.0 ("x1"), "y2"=200000.0 ("x1")) -> ("y"=w742:dbl)  [unwired: 2 in]
          }
          frame #8 {
            # "8"
            # "AI17 P 3He OUT"
            n377 = Add Array Elements(numeric array=w754) -> (sum=w755:dbl)
            n378 = Divide(x=w755, y=w753) -> (x/y=w750:dbl)
            n379 = call "scaling_calculator_baratron.vi"("x"=w750, "offset subt"="idx 8 Vbar offset") -> ("y (Pa)"=w752:dbl)  [unwired: 4 in, 1 out]
          }
          frame #9 {
            # "9"
            # "BARATRON"
            n380 = Add Array Elements(numeric array=w760) -> (sum=w757:dbl)
            n381 = Divide(x=w757, y=w761) -> (x/y=w756:dbl)
            n382 = call "scaling_calculator_baratron.vi"("x"=w756, "offset subt"="idx 9 Vbar offset") -> ("y (Pa)"=w759:dbl)  [unwired: 4 in, 1 out]
          }
          frame #10 {
            # "10"
            # "BARATRON"
            n383 = Add Array Elements(numeric array=w766) -> (sum=w763:dbl)
            n384 = Divide(x=w763, y=w767) -> (x/y=w762:dbl)
            n385 = call "scaling_calculator_baratron.vi"("x"=w762, "offset subt"="idx 10 Vbar offset") -> ("y (Pa)"=w765:dbl)  [unwired: 4 in, 1 out]
          }
        }
        n386 = Subtract(x=w510, y=w513) -> (x-y=→"V10 - V9":dbl)
        n387 = Subtract(x=w514, y=w511) -> (x-y=→"V9 - V8":dbl)
        n388 = Subtract(x=w510, y=w511) -> (x-y=→"V10 - V8":dbl)
        n389 = local read "current time"() -> (w565:timestamp)
        n390 = Build Array(w594, w592, w590, w587, w586, w585, w583, w567, w530, w529, w541) -> (w528:dbl[])
        "DAQ CONV. OUT" <- w528
        n391 = local read "Cycle #"() -> (w562:i32)
        n392 = To Double Precision Float(number=w565) -> (double precision float=w609:dbl)
        n393 = call "LV_UNIX.vi"("current time"=w565) -> ("date/time string"=w563:string, "UNIX time (s)"=w564:dbl)  [unwired: 9 in]
        n394 = Build Array (concatenate)(w596, w528) -> (w566:dbl[][])
        n395 = Index Array(array=w528) -> (element #1=w517:dbl, element #2=w527:dbl, element #3=w526:dbl, element #4=w525:dbl, element #5=w524:dbl, element #6=w523:dbl, element #7=w522:dbl, element #8=w521:dbl, element #9=w520:dbl, element #10=w519:dbl, element #11=w518:dbl)  [unwired: 11 in]
        n396 = case shown="True" TRUE {
          tunnel: w609 -> [_ w628]
          tunnel: w564 -> [_ w629]
          tunnel: w563 -> [_ w630]
          tunnel: w562 -> [_ w631]
          tunnel: w527 -> [_ w645]
          tunnel: w526 -> [_ w644]
          tunnel: w525 -> [_ w643]
          tunnel: w524 -> [_ w642]
          tunnel: w523 -> [_ w641]
          tunnel: w522 -> [_ w640]
          tunnel: w521 -> [_ w639]
          tunnel: w520 -> [_ w638]
          tunnel: w519 -> [_ w637]
          tunnel: w518 -> [_ w636]
          tunnel: w517 -> [_ w635]
          frame False {
          }
          frame True {
            w634 = "%d,%s,%10.4f,%10.4f,%5.6f,%5.6f,%5.6f,%5.6f,%5.6f,%5.6f,%5.6f,%9.6f,%9.6f,%9.6f,%9.6f\\n" ("format string")
            n397 = local read "error out\n(file creation)"() -> (w615:errorcluster)
            n398 = local read "ref RAW"() -> (w633:refnum<file>)
            n399 = local read "RAW (V)"() -> (w627:dbl[])
            n400 = Index Array(array=w627) -> (element #1=w626:dbl, element #2=w625:dbl, element #3=w624:dbl, element #4=w623:dbl, element #5=w622:dbl, element #6=w621:dbl, element #7=w620:dbl, element #8=w619:dbl, element #9=w618:dbl, element #10=w617:dbl, element #11=w616:dbl)  [unwired: 11 in]
            n401 = Format Into String(format string=w634, initial string=w633, error in=w615, w631, w630, w629, w628, w626, w625, w624, w623, w622, w621, w620, w619, w618, w617, w616) -> (error out=w632:errorcluster)  [unwired: 1 out]
            n402 = local read "ref DAQ"() -> (w646:refnum<file>)
            n403 = Format Into String(format string=w634, initial string=w646, error in=w632, w631, w630, w629, w628, w635, w645, w644, w643, w642, w641, w640, w639, w638, w637, w636) -> (error out=→"error out \n(record DAQ)":errorcluster)  [unwired: 1 out]
          }
        }
        n404 = Index Array(array=w566, index (col) #1=0 ("disabled index (col)"), index (col) #2=1 ("disabled index (col)"), index (col) #3=2 ("disabled index (col)"), index (col) #4=3 ("disabled index (col)"), index (col) #5=4 ("index (col)"), index (col) #6=5 ("index (col)"), index (col) #7=6 ("index (col)"), index (col) #8=7 ("index (col)"), index (col) #9=8 ("index (col)"), index (col) #10=9 ("index (col)"), index (col) #11=10 ("index (col)")) -> (element #1=w607:dbl[], element #2=w605:dbl[], element #3=w603:dbl[], element #4=w601:dbl[], element #5=w598:dbl[], element #6=w597:dbl[], element #7=w581:dbl[], element #8=w557:dbl[], element #9=w556:dbl[], element #10=w535:dbl[], element #11=w533:dbl[])  [unwired: 11 in]
        n405 = Bundle(w531, w603) -> (w555:cluster{dbl[], dbl[]})  [unwired: 1 in]
        n406 = Bundle(w531, w601) -> (w554:cluster{dbl[], dbl[]})  [unwired: 1 in]
        n407 = Bundle(w531, w598) -> (w553:cluster{dbl[], dbl[]})  [unwired: 1 in]
        n408 = Bundle(w531, w597) -> (w552:cluster{dbl[], dbl[]})  [unwired: 1 in]
        n409 = Bundle(w531, w557) -> (w551:cluster{dbl[], dbl[]})  [unwired: 1 in]
        n410 = Bundle(w531, w581) -> (w550:cluster{dbl[], dbl[]})  [unwired: 1 in]
        n411 = Bundle(w531, w556) -> (w548:cluster{dbl[], dbl[]})  [unwired: 1 in]
        n412 = Bundle(w531, w535) -> (w534:cluster{dbl[], dbl[]})  [unwired: 1 in]
        n413 = Bundle(w531, w533) -> (w532:cluster{dbl[], dbl[]})  [unwired: 1 in]
        n414 = Bundle(w531, w605) -> (w560:cluster{dbl[], dbl[]})  [unwired: 1 in]
        n415 = Bundle(w531, w607) -> (w561:cluster{dbl[], dbl[]})  [unwired: 1 in]
        n416 = Build Array(w561, w560, w555, w554, w553, w552, w551, w550, w548, w534, w532) -> (w547:cluster{dbl[], dbl[]}[])
        n417 = stacked-sequence {
          tunnel: w547 -> [w650 w656 w661 w666 w671 w676]
          frame #0 {
            n418 = control-ref of="Graph S. 1"() -> (w651:refnum<vi>)
            n419 = property class="XYGraph (strict)"(reference=w651, error in=errorcluster {"status"=FALSE, "code"=0, "source"=""} ("error in (no error)"), "Value"=w650) -> (error out=w648:errorcluster)  [unwired: 1 out]
            n420 = control-ref of="error plot content"() -> (w649:refnum<vi>)
            n421 = property class="Clust (strict)"(reference=w649, "Value"=w648) -> ()  [unwired: 1 in, 2 out]
          }
          frame #1 {
            n422 = control-ref of="Graph S. 2"() -> (w653:refnum<vi>)
            n423 = property class="XYGraph (strict)"(reference=w653, error in=errorcluster {"status"=FALSE, "code"=0, "source"=""} ("error in (no error)"), "Value"=w656) -> (error out=w654:errorcluster)  [unwired: 1 out]
            n424 = control-ref of="error plot content"() -> (w655:refnum<vi>)
            n425 = property class="Clust (strict)"(reference=w655, "Value"=w654) -> ()  [unwired: 1 in, 2 out]
          }
          frame #2 {
            n426 = control-ref of="Graph S. 3"() -> (w658:refnum<vi>)
            n427 = property class="XYGraph (strict)"(reference=w658, error in=errorcluster {"status"=FALSE, "code"=0, "source"=""} ("error in (no error)"), "Value"=w661) -> (error out=w659:errorcluster)  [unwired: 1 out]
            n428 = control-ref of="error plot content"() -> (w660:refnum<vi>)
            n429 = property class="Clust (strict)"(reference=w660, "Value"=w659) -> ()  [unwired: 1 in, 2 out]
          }
          frame #3 {
            n430 = control-ref of="Graph S. 4"() -> (w663:refnum<vi>)
            n431 = property class="XYGraph (strict)"(reference=w663, error in=errorcluster {"status"=FALSE, "code"=0, "source"=""} ("error in (no error)"), "Value"=w666) -> (error out=w664:errorcluster)  [unwired: 1 out]
            n432 = control-ref of="error plot content"() -> (w665:refnum<vi>)
            n433 = property class="Clust (strict)"(reference=w665, "Value"=w664) -> ()  [unwired: 1 in, 2 out]
          }
          frame #4 {
            n434 = control-ref of="Graph S. 5"() -> (w668:refnum<vi>)
            n435 = property class="XYGraph (strict)"(reference=w668, error in=errorcluster {"status"=FALSE, "code"=0, "source"=""} ("error in (no error)"), "Value"=w671) -> (error out=w669:errorcluster)  [unwired: 1 out]
            n436 = control-ref of="error plot content"() -> (w670:refnum<vi>)
            n437 = property class="Clust (strict)"(reference=w670, "Value"=w669) -> ()  [unwired: 1 in, 2 out]
          }
          frame #5 {
            n438 = control-ref of="Graph S. 6"() -> (w673:refnum<vi>)
            n439 = property class="XYGraph (strict)"(reference=w673, error in=errorcluster {"status"=FALSE, "code"=0, "source"=""} ("error in (no error)"), "Value"=w676) -> (error out=w674:errorcluster)  [unwired: 1 out]
            n440 = control-ref of="error plot content"() -> (w675:refnum<vi>)
            n441 = property class="Clust (strict)"(reference=w675, "Value"=w674) -> ()  [unwired: 1 in, 2 out]
          }
        }
      }
      frame #1 {
        n442 = local read "error out \n(DAQ IN)"() -> (w769:errorcluster)
        n443 = local read "DAQ OUT ON?"() -> (w771:bool)
        n444 = case shown="True" w771 {
          tunnel: w772 -> [w774 w779]
          tunnel: [w774 w778] -> w770
          tunnel: w769 -> [w773 w776]
          tunnel: [w773 w775] -> w768
          frame False {
          }
          frame True {
            n445 = call <vilib>:"DAQmx Write (Analog 1D DBL 1Chan NSamp).vi"("task/channels in"=w779, "data"="DAQ OUT SET Volt", "timeout"=100.0, "error in"=w776) -> ("task out"=w778:refnum<k21>, "number of samples written per channel"=→"DAQ OUT \nsample #":u32, "error out"=w775:errorcluster)  [unwired: 9 in]
          }
        }
        "error out\n(DAQ OUT)" <- w768
      }
    }
    "Cycle #" <- w503
  }
  n446 = call <vilib>:"DAQmx Stop Task.vi"("task/channels in"=w12, "error in"=w10) -> ("task out"=w14:refnum<k21>, "error out"=w13:errorcluster)  [unwired: 12 in]
  n447 = call <vilib>:"DAQmx Clear Task.vi"("task in"=w14, "error in"=w13) -> ("error out"=w16:errorcluster)  [unwired: 13 in]
  n448 = call <vilib>:"DAQmx Stop Task.vi"("task/channels in"=w11, "error in"=w16) -> ("task out"=w18:refnum<k21>, "error out"=w15:errorcluster)  [unwired: 12 in]
  n449 = call <vilib>:"DAQmx Clear Task.vi"("task in"=w18, "error in"=w15) -> ("error out"=→"error out DAQ close":errorcluster)  [unwired: 13 in]
